vi "VR Controler 8.5.vi"() -> ()   [LabVIEW 2017]
uses:
  Sub VIs/Reward zone location enum.ctl
  Sub VIs/Record enum.ctl
  Sub VIs/Socket enum.ctl
  Sub VIs/Main program enum2.ctl
  <vilib>/vision/Image Controls.llb/IMAQ Image.ctl
  c98a875a-e3b8-49f2-a6fc-eefafe62491b.vi
  5779e0b0-41b7-4506-a67f-138f79383ca8.vi
  b241f941-595d-4c0c-9393-2e10ae48b17b.vi
  1da1cb31-40b1-4a67-a7e6-56ad72bdf787.vi
  <vilib>/DAQmx/write.llb/DAQmx Write (Digital Bool 1Line 1Point).vi
  eb595f88-4225-414f-83f1-01d5d940fc66.vi
  1662c5e6-2776-4c60-b5b4-ceaeea1864d3.vi
  fb6b5c9d-106e-453b-a883-cc93056fac18.vi
  6954e0aa-8682-46cf-8e13-c82c99879c30.vi
  6235507b-2202-4f21-86ca-b7b41428e472.vi
  835dcb76-40d0-41c5-8fe3-3989c1fd9891.vi
  4796a129-a1f4-4c2b-9c8a-39875efc01cf.vi
  bf4008ee-ae26-4c0a-87de-22156137ce73.vi
  cfabecd4-7210-4e1d-87ea-acbfc879dca4.vi
  636e59bd-2132-4706-8f21-063dc2cad597.vi
  fa866b4b-dc6c-4481-bc67-f1512cbbaaf9.vi
  f0a6b648-ccd6-4e98-b62c-d3930b5e7adb.vi
  6f1d6b9c-7e66-4bfa-a54a-0bf9111e914d.vi
  4b664865-0372-4337-9de9-faa9f3913aab.vi
  63df5311-9246-4ffc-851f-b70ac2e65be5.vi
  <vilib>/DAQmx/read.llb/DAQmx Read (Analog 2D DBL NChan NSamp).vi
  <vilib>/DAQmx/read.llb/DAQmx Read (Digital 2D U8 NChan NSamp).vi
  <vilib>/DAQmx/read.llb/DAQmx Read (Counter 1D DBL 1Chan NSamp).vi
  <vilib>/DAQmx/create/channels.llb/DAQmx Create Channel (DO-Digital Output).vi
  <vilib>/Utility/file.llb/Read Delimited Spreadsheet (string).vi
  <vilib>/DAQmx/create/channels.llb/DAQmx Create Channel (CO-Pulse Generation-Frequency).vi
  <vilib>/DAQmx/configure/timing.llb/DAQmx Timing (Implicit).vi
  <vilib>/DAQmx/miscellaneous.llb/DAQmx Fill In Error Info.vi
  <vilib>/DAQmx/create/channels.llb/DAQmx Create Channel (AI-Voltage-Basic).vi
  <vilib>/DAQmx/create/channels.llb/DAQmx Create Channel (DI-Digital Input).vi
  <vilib>/DAQmx/configure/timing.llb/DAQmx Timing (Sample Clock).vi
  <vilib>/Utility/file.llb/Write Delimited Spreadsheet (string).vi
  <vilib>/Analysis/NI_AALBase.lvlib
  3ac8b79d-dcd6-4b4b-a391-90696fb8637b.vi
  <resource>/objmgr/daqmx.rc
  2d51e364-e5e4-467f-ae98-a57dce561a7d.vi
  b1e57f22-ab38-4a20-aa80-3e76a4c4245a.vi
  e4fbd320-8e96-403f-b1da-5dadb21a4556.vi
  13745751-d4af-40e9-a17d-77a3f366e404.vi
  fbb1eb04-9408-43f0-a0c5-a56a247c35dd.vi
  <vilib>/vision/driver/NI_Vision_Acquisition_Software.lvlib
  <vilib>/Analysis/baseanly.llb/Mean (DBL).vi
  <vilib>/DAQmx/configure/task.llb/DAQmx Configure Logging (TDMS).vi
panel:
  out "Start mask stim":bool
  out "Stop mask stim":bool
  out "Mask prot command":u16
  out "Stim prot command":u16
  out "Valve open":bool
  out "Within Reward zone":bool
  out "Reward given":bool
  out "Lick":bool
  out "Masking light 2":bool
  out "Unity connected":bool
  out "Mate":bool
  out "Start light stim":bool
  out "Light ON":bool
  out "Stop light stim":bool
  out "Header":string
  in  "Software version":string
  in  "Shuffle":bool
  out "Write loop stopped":bool
  out "msg tag":string
  in  "Tab Control 4":enum32{"0", "1", "2", "3", "4"}(tab)
  in  "Tab Control 3":enum32{"0", "1", "2", "3", "4"}(tab)
  in  "Gain":dbl
  in  "sound cue presented":bool
  out "Store prev encoder count":dbl
  out "Read loop stopped":bool
  in  "index":i32
  out "Water cnt. reset":i32
  out "lick signal":i8[](array[numeric])
  out "My tdms file":refnum<k34>
  out "Trial counted":bool
  out "Stim trial":bool
  out "Write":bool
  out "read":bool
  in  "select trial":bool
  out "delta distance cm":dbl[](array[numeric])
  in  "VR Controller":enum32{"Main panel", "Settings"}(tab)
  out "Frame signal indicator 2":bool
  in  "Timed reward (s)":u32
  in  "Various GUI elements":enum32{"Misc", "Eye tracker", "Security camera"}(tab)
  in  "VR start pos":T1(ring)
  out "Opt stim command":dbl[](graph)
  out "Current stim. protocol":string
  out "Random start pos":bool=TRUE
  out "Next trial stim. protocol":string
  out "Current mask protocol":string
  out "Next mask protocol":string
  in  "start with ramp":bool
  out "stim loop rate":dbl
  out "Pupille image saved":bool
  in  "Record Button 2":bool
  in  "Black Level":dbl(slide)=0.9896907216494839 min=-32.0 max=31.75 scale=-32.0..32.0
  in  "Gain":dbl(slide)=8.879999999999999 min=0.0 max=24.0 step=1.0 scale=0.0..24.0
  in  "Exposure Time (ms)":dbl(slide)=15144.329896907217 min=1.0 max=15.0 scale=0.0..15.0
  in  "Target frame rate":dbl=60.0 min=1.0 max=144.0 step=1.0
  out "Pupille image":T2(plugin-control)
  out "Frame rate":dbl
  in  "Image Format Control::Offset X":i64(slide) min=0 max=450 step=2 scale=0.0..450.0
  in  "Image Format Control::Offset Y":i64(slide) min=0 max=350 step=2 scale=0.0..350.0
  out "Lost Image Count":u32
  out "Total Images Transferred":u32
  out "Security cam image":T2(plugin-control)
  in  "Cam ON /OFF":bool
  out "Stim. count":i32
  in  "Random reward":bool
  out "Frame signal indicator":bool
  in  "Hybrid licking":bool
  in  "Boolean":bool
  in  "SciScan":bool
  in  "Comment":string
  out "Photodiode":bool
  out "Trial type ettings":enum32{"Page 1", "Page 2"}(tab)
  in  "mask. num. 5":u16
  in  "Mask prot 5":u16(ring) items=["none", "20 Hz sinus from -80 to rew int. 100 % duty cycle 0 %", "20 Hz sinus from -50 to 10 int. 100 % duty cycle 0 %", "20 Hz sinus from 10 to 130 int. 100 % duty cycle 0 %", "20 Hz sinus from 10 to 20 int. 100 % duty cycle 0 %", "20 Hz sinus from 10 to 70 int. 100 % duty cycle 0 %", "20 Hz sinus from 10 to rew int. 100 % duty cycle 0 %", "20 Hz sinus from 0 to 70 int. 100 % duty cycle 0 %", "20 Hz sinus from 0 to 70 int. 50 % duty cycle 0 %", "continuous from 0 to 70 int. 100 % duty cycle 0 %"]
  in  "mask. num. 4":u16
  in  "Mask prot 4":u16(ring) items=["none", "20 Hz sinus from -80 to rew int. 100 % duty cycle 0 %", "20 Hz sinus from -50 to 10 int. 100 % duty cycle 0 %", "20 Hz sinus from 10 to 130 int. 100 % duty cycle 0 %", "20 Hz sinus from 10 to 20 int. 100 % duty cycle 0 %", "20 Hz sinus from 10 to 70 int. 100 % duty cycle 0 %", "20 Hz sinus from 10 to rew int. 100 % duty cycle 0 %", "20 Hz sinus from 0 to 70 int. 100 % duty cycle 0 %", "20 Hz sinus from 0 to 70 int. 50 % duty cycle 0 %", "continuous from 0 to 70 int. 100 % duty cycle 0 %"]
  in  "mask. num. 3":u16
  in  "Mask prot 3":u16(ring) items=["none", "20 Hz sinus from -80 to rew int. 100 % duty cycle 0 %", "20 Hz sinus from -50 to 10 int. 100 % duty cycle 0 %", "20 Hz sinus from 10 to 130 int. 100 % duty cycle 0 %", "20 Hz sinus from 10 to 20 int. 100 % duty cycle 0 %", "20 Hz sinus from 10 to 70 int. 100 % duty cycle 0 %", "20 Hz sinus from 10 to rew int. 100 % duty cycle 0 %", "20 Hz sinus from 0 to 70 int. 100 % duty cycle 0 %", "20 Hz sinus from 0 to 70 int. 50 % duty cycle 0 %", "continuous from 0 to 70 int. 100 % duty cycle 0 %"]
  in  "mask. num. 2":u16
  in  "Mask prot 2":u16(ring) items=["none", "20 Hz sinus from -80 to rew int. 100 % duty cycle 0 %", "20 Hz sinus from -50 to 10 int. 100 % duty cycle 0 %", "20 Hz sinus from 10 to 130 int. 100 % duty cycle 0 %", "20 Hz sinus from 10 to 20 int. 100 % duty cycle 0 %", "20 Hz sinus from 10 to 70 int. 100 % duty cycle 0 %", "20 Hz sinus from 10 to rew int. 100 % duty cycle 0 %", "20 Hz sinus from 0 to 70 int. 100 % duty cycle 0 %", "20 Hz sinus from 0 to 70 int. 50 % duty cycle 0 %", "continuous from 0 to 70 int. 100 % duty cycle 0 %"]
  out "mask. num. 1":u16
  out "Mask prot 1":u16(ring) items=["none", "20 Hz sinus from -80 to rew int. 100 % duty cycle 0 %", "20 Hz sinus from -50 to 10 int. 100 % duty cycle 0 %", "20 Hz sinus from 10 to 130 int. 100 % duty cycle 0 %", "20 Hz sinus from 10 to 20 int. 100 % duty cycle 0 %", "20 Hz sinus from 10 to 70 int. 100 % duty cycle 0 %", "20 Hz sinus from 10 to rew int. 100 % duty cycle 0 %", "20 Hz sinus from 0 to 70 int. 100 % duty cycle 0 %", "20 Hz sinus from 0 to 70 int. 50 % duty cycle 0 %", "continuous from 0 to 70 int. 100 % duty cycle 0 %"]
  in  "stim. num. 5":u16
  in  "Stim. prot 5":u16(ring) items=["none", "20 Hz sinus from -80 to rew int. 100 % duty cycle 0 %", "20 Hz sinus from -50 to 10 int. 100 % duty cycle 0 %", "20 Hz sinus from 10 to 130 int. 100 % duty cycle 0 %", "20 Hz sinus from 10 to 20 int. 100 % duty cycle 0 %", "20 Hz sinus from 10 to 70 int. 100 % duty cycle 0 %", "20 Hz sinus from 10 to rew int. 100 % duty cycle 0 %", "20 Hz sinus from 0 to 70 int. 100 % duty cycle 0 %", "20 Hz sinus from 0 to 70 int. 50 % duty cycle 0 %", "continuous from 0 to 70 int. 100 % duty cycle 0 %"]
  in  "stim. num. 4":u16
  in  "Stim. prot 4":u16(ring) items=["none", "20 Hz sinus from -80 to rew int. 100 % duty cycle 0 %", "20 Hz sinus from -50 to 10 int. 100 % duty cycle 0 %", "20 Hz sinus from 10 to 130 int. 100 % duty cycle 0 %", "20 Hz sinus from 10 to 20 int. 100 % duty cycle 0 %", "20 Hz sinus from 10 to 70 int. 100 % duty cycle 0 %", "20 Hz sinus from 10 to rew int. 100 % duty cycle 0 %", "20 Hz sinus from 0 to 70 int. 100 % duty cycle 0 %", "20 Hz sinus from 0 to 70 int. 50 % duty cycle 0 %", "continuous from 0 to 70 int. 100 % duty cycle 0 %"]
  in  "stim. num. 3":u16
  in  "Stim. prot 3":u16(ring) items=["none", "20 Hz sinus from -80 to rew int. 100 % duty cycle 0 %", "20 Hz sinus from -50 to 10 int. 100 % duty cycle 0 %", "20 Hz sinus from 10 to 130 int. 100 % duty cycle 0 %", "20 Hz sinus from 10 to 20 int. 100 % duty cycle 0 %", "20 Hz sinus from 10 to 70 int. 100 % duty cycle 0 %", "20 Hz sinus from 10 to rew int. 100 % duty cycle 0 %", "20 Hz sinus from 0 to 70 int. 100 % duty cycle 0 %", "20 Hz sinus from 0 to 70 int. 50 % duty cycle 0 %", "continuous from 0 to 70 int. 100 % duty cycle 0 %"]
  in  "stim. num. 2":u16
  in  "Stim. prot 2":u16(ring) items=["none", "20 Hz sinus from -80 to rew int. 100 % duty cycle 0 %", "20 Hz sinus from -50 to 10 int. 100 % duty cycle 0 %", "20 Hz sinus from 10 to 130 int. 100 % duty cycle 0 %", "20 Hz sinus from 10 to 20 int. 100 % duty cycle 0 %", "20 Hz sinus from 10 to 70 int. 100 % duty cycle 0 %", "20 Hz sinus from 10 to rew int. 100 % duty cycle 0 %", "20 Hz sinus from 0 to 70 int. 100 % duty cycle 0 %", "20 Hz sinus from 0 to 70 int. 50 % duty cycle 0 %", "continuous from 0 to 70 int. 100 % duty cycle 0 %"]
  out "stim. num. 1":u16
  out "Stim. prot 1":u16(ring) items=["none", "20 Hz sinus from -80 to rew int. 100 % duty cycle 0 %", "20 Hz sinus from -50 to 10 int. 100 % duty cycle 0 %", "20 Hz sinus from 10 to 130 int. 100 % duty cycle 0 %", "20 Hz sinus from 10 to 20 int. 100 % duty cycle 0 %", "20 Hz sinus from 10 to 70 int. 100 % duty cycle 0 %", "20 Hz sinus from 10 to rew int. 100 % duty cycle 0 %", "20 Hz sinus from 0 to 70 int. 100 % duty cycle 0 %", "20 Hz sinus from 0 to 70 int. 50 % duty cycle 0 %", "continuous from 0 to 70 int. 100 % duty cycle 0 %"]
  in  "Trial block":u16 max=100
  in  "Primary masking light":T3(ring)
  in  "Location of reward zone":T4 items=["80 cm", "120 cm", "180  cm", "270 cm", "400 cm"]
  in  "Enable stim.":bool
  out "GUI version":enum32{"Page 1", "Page 2"}(tab)
  out "Hit trials stim.":i32
  out "?":dbl(slide) scale=-140.0..190.0
  in  "Reset top plot":bool=TRUE caption="Reset"
  in  "Reset bottom plot":bool=TRUE caption="Reset"
  out "Hit trials ctrl.":i32
  out "P stim. Hit":dbl(slide) scale=0.0..1.0
  out "P ctrl. Hit":dbl(slide) scale=0.0..1.0
  out "Control hit trials %":dbl
  out "Stim. hit trials %":dbl
  out "Tab Control":enum32{"0", "1", "2", "3", "4"}(tab)
  out "Tab Control 2":enum32{"0", "1", "2", "3", "4"}(tab)
  out "Next":bool
  out "Top Graph":cluster{"Y":dbl[], "Y":dbl[]}[](graph) caption="XY Graph"
  out "Bottom Graph":cluster{"Y":dbl[], "Y":dbl[]}[](graph) caption="XY Graph"
  out "Hit trials %":dbl format="%#.1g"
  out "Hit trials":i16
  out "Wheel position graph":cluster{"Y":dbl[], "Y":dbl[]}[](graph) caption="XY Graph"
  in  "Reset wheel pos. graph":bool=TRUE caption="Reset"
  out "P hit trials":dbl(slide) scale=0.0..1.0
  out "Lick and reward chart 2":cluster{dbl, i16}(graph)
  out "%":dbl format="%#_3g"
  in  "Weight":dbl
  in  "Lab book notes":string
  in  "Open valve":bool
  in  "Reward freq. (cm)":dbl
  in  "Reward zone":bool
  out "Distance (m)":dbl format="%#.2g"
  in  "Record Button":bool
  in  "Reset water count":bool
  out "Water received (ul)":dbl
  in  "VR Mode":bool
  out "All trials":i32
  out "Ctrl. count":i32
  out "Unique ID":i8 format="%2d"
  in  "Stop recording":bool
  in  "Start recording":bool
  out "Laps":i32
  in  "Exit program":bool
  in  "counter reset (F)":bool caption="stop (F)"
  out "total distance cm":sgl[](array[numeric])
  out "Position on the wheel":dbl(knob) scale=0.0..157.0
  out "Experiment time (s)":dbl
  in  "Give reward":bool
  in  "Repetition":i32
  out "Date":string
  out "Run experiment":bool
  out "Velocity chart":dbl(graph)
  out "Lick and reward chart":cluster{dbl, i16}(graph)
  out "Record":bool
  out "Time (min)":dbl format="%#.2g"
  in  "Active licking":bool
  out "Mouse name":string
  in  "Scrollbar":i32(c297)
  out "Velocity chart 2":dbl(graph)
  out "Laser ON":bool
  in  "Extra stop triggers":bool
  in  "Photo diode threshold":dbl=1.5
  out "stim started":bool
  in  "Eable eye cam":bool
  out "start of stim":bool
  out "Waveform Graph":dynamicdata(graph)
  in  "Duty cycle (%)":u8=50 max=100 step=1
  out "Relative position":dbl
  out "random rew":dbl
  out "offset tag":string
  out "Masking light prot":string
  out "velocity (cm/s)":dbl
  out "Security camera":string
  out "2P imaging":string
  out "hit trial":bool
  out "Session start:":string
  out "miss trial":bool
  out "Distance (cm)":dbl
  out "Prev. rew. pos.":dbl
  out "encoder ticks per rev":dbl
  out "prev. diode position":dbl
  out "Stimulus protocol":string
  out "Laser stimulus calibration":string
  out "Original weight":dbl
  out "Last calibration":string
  in  "Edit mouse list":bool
  out "Socket read loop rate":u32(graph)
  out "Delta time (ms)":u32(graph)
  out "No. of smpl. per ch.":i32
  out "Loop rate":dbl
  out "Sample rate":dbl
  out "reward zone end":dbl
  out "reward zone start":dbl
  in  "Corridor length":i32
  out "delta time (s)":dbl format="%#.8g"
  out "Experiment time (ms)":u32
  out "Start time":u32
  in  "Sound duration (ms)":u32=25
  in  "Valve open dur. (ms)":u32=25
  in  "working directory":path=path ""
  in  "command line":string
  in  "Recording folder":path
  out "Wheel circumference":dbl
  in  "Record enum":T5
  in  "Reward size (ul)":dbl min=0.0 step=inf format="%#.2g"
  in  "working directory 2":path=path ""
  out "Record loop state":T5
  out "Reward read loop rate":u32(graph)
  out "shuffled array":i16[](array[numeric])
  in  "Current mice":string[][](array[string])
  out "Trial types":u16[][](array[numeric])
  out "Last saved reward size":dbl
  out "Encoder count":dbl
  out "Lick indicator":dbl
  out "Lab book file":path
  out "Filename":string
  out "Frame signal":i8[](array[numeric])
  out "Water count":i32
  out "Unity position:":sgl
  out "Raw position:":dbl
  out "Photodiode signal":sgl[](array[numeric])
  out "Trial type array":i8[][](array[numeric])
  out "Valve signal":i8[](array[numeric])
  out "SciScan start":refnum<k21>
  out "Photo stimulus signal":sgl[](array[numeric])
  in  "NBC Gain":dbl
  out "Encoder signal":sgl[](array[numeric])
  out "analog lick":sgl[](array[numeric])
  out "protocol array":string[][](array[string])
  in  "Stim protocols":u16(ring) items=["none", "20 Hz sinus from -80 to rew int. 100 % duty cycle 0 %", "20 Hz sinus from -50 to 10 int. 100 % duty cycle 0 %", "20 Hz sinus from 10 to 130 int. 100 % duty cycle 0 %", "20 Hz sinus from 10 to 20 int. 100 % duty cycle 0 %", "20 Hz sinus from 10 to 70 int. 100 % duty cycle 0 %", "20 Hz sinus from 10 to rew int. 100 % duty cycle 0 %", "20 Hz sinus from 0 to 70 int. 100 % duty cycle 0 %", "20 Hz sinus from 0 to 70 int. 50 % duty cycle 0 %", "continuous from 0 to 70 int. 100 % duty cycle 0 %"]
  in  "Stim type":u16(ring) items=["none", "10 Hz sinus", "20 Hz sinus", "40 Hz sinus", "continuous", "10 Hz square", "20 Hz square", "40 Hz square"]
  in  "from reward":bool
  in  "to reward":bool
  in  "Intensity (%)":u8=100 max=100 step=1
  in  "stop (cm)":i32
  in  "start (cm)":i32
  out "prev. stim. type":string
  out "prev. max stim. V":dbl
  out "Eye cam frame signal":i8[](array[numeric])
  in  "Eable security cam":bool
  out "Eyecam states":T6(ring)
  out "settings folder":path
  out "Pupil Exp day folder":path
  out "ML signal":sgl[](array[numeric])
  out "Frame signal 2":i8[](array[numeric])
  out "Exit":bool
  out "Stop Unity":bool
  # "All"
  # "This session"
  # "Reward conditions"
  # "Trial type settings"
  # "Determine stimulus protocol and \nreperition (numerator) in relation \nto the denominator!"
  # "%"
  # "%"
  # "%"
  # "Edit stimulus protocols for photo stimulation and/or \na secondary masking light. Chose a protocol from the \nlist and define parameters."
  # "Mouse name               Headbar           Original weight"
  # "Variables"
  # "Reward settings"
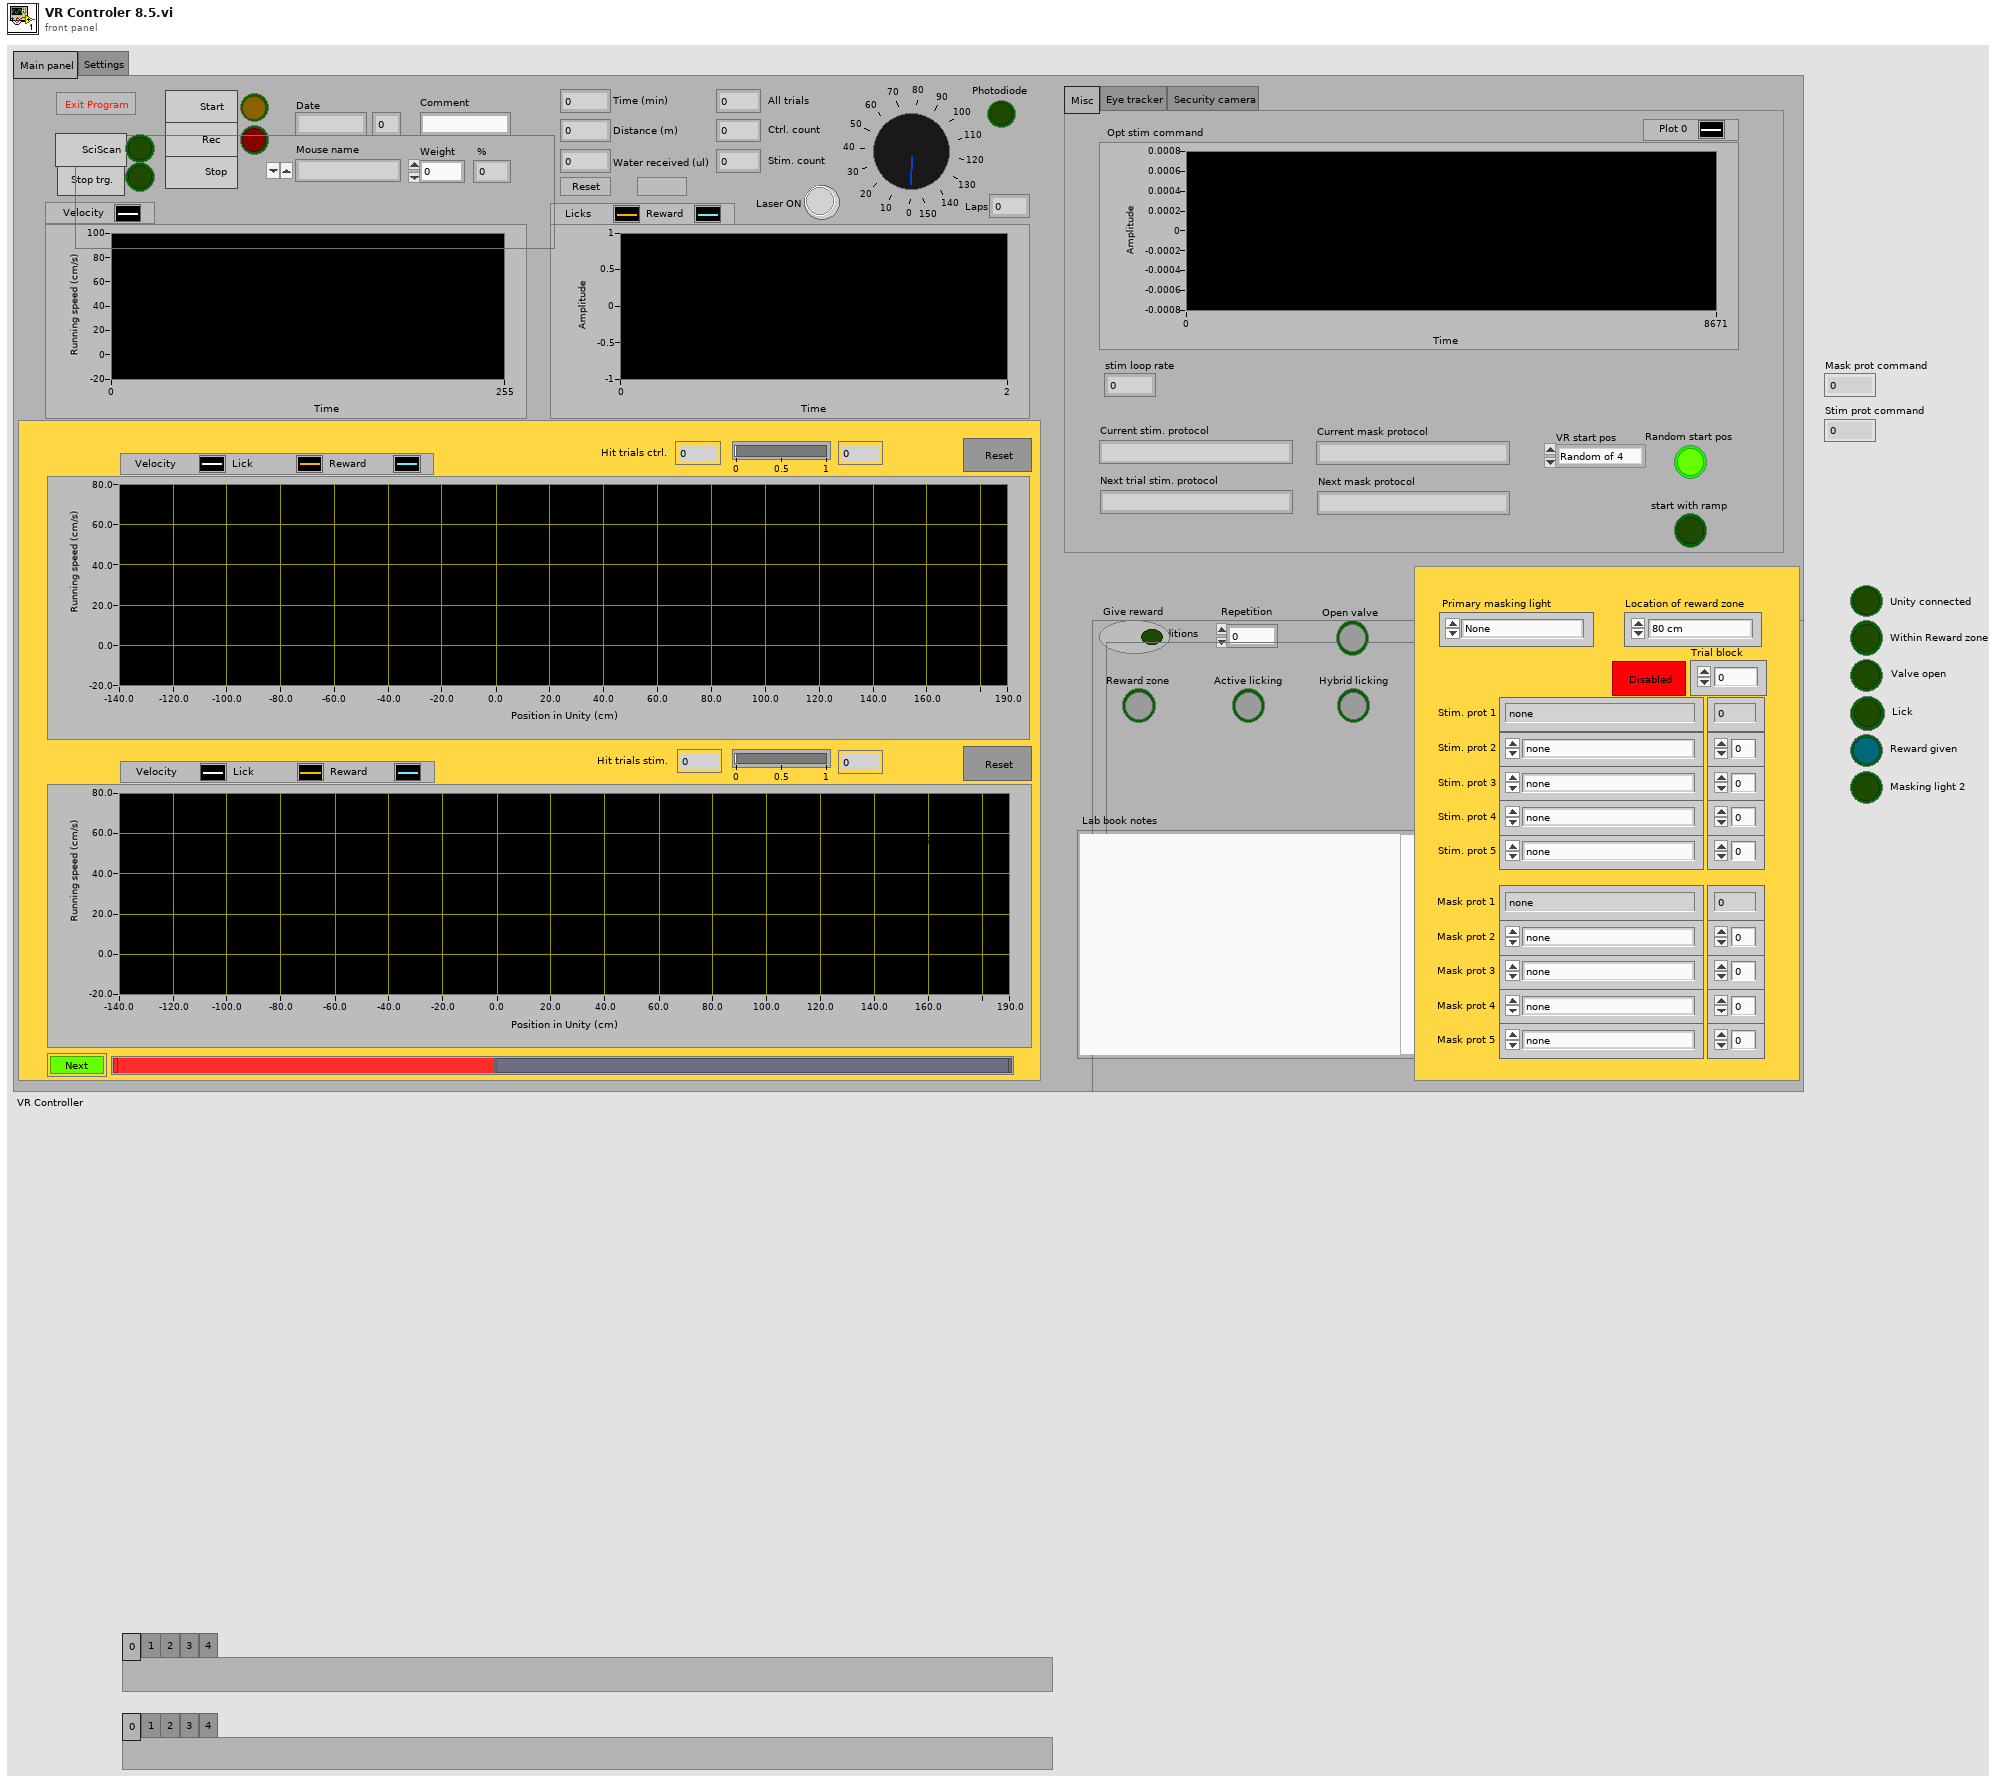
[diagram p1: front panel]
types:
  T1 = enum16{"Random of 4", "Random of 2", "Non-random"}
  T2 = typedef "IMAQ Image.ctl" = refnum<image>
  T3 = enum16{"None", "20 Hz until reward ", "Continuous specified light off trials", "Continuous specified all trials", "20 Hz specified light off trials", "20 Hz specified all trials", "20 Hz full trial", "Continuous full trial"}
  T4 = typedef "Reward zone location enum.ctl" = u16
  T5 = typedef "Record enum.ctl" = enum16{"Idle", "Init recording", "Init data acquisition", "Record VR", "Record", "Stop data acquision"}
  T6 = enum16{"Idle", "Set params", "Start recording", "Record pupille", "Stop recording"}
  T7 = enum8{"Enabled", "Disabled", "Disabled and Grayed Out"}
  T8 = typedef "Main program enum2.ctl" = enum16{"Init program", "Idle", "Init recording ", "Record", "Record VR", "Stop Recording", "Exit program"}
  T9 = typedef "Socket enum.ctl" = enum16{"Socket not connected", "Init socket", "Socket connected", "Close socket"}
  T10 = cluster{"Type":u32, "Version":u32, "Flags":u32, "SerialNumberHigh":u32, "SerialNumberLow":u32, "BusType":u32, "InterfaceName":string, "VendorName":string, "ModelName":string, "CameraFileName":string, "CameraAttributeURL":string}[]
  T11 = enum16{"open", "replace", "create", "open or create", "replace or create", "replace or create with confirmation"}
  T12 = enum16{"Init program", "Idle", "Init recording ", "Record", "Record VR", "Stop Recording", "Exit program"}
  T13 = enum16{"None", "Full trial 40 Hz sinus ", "Full trial 20 Hz sinus", "Continuous light ON", "Until reward 40 Hz sinus"}
  T14 = enum16{"None", "20 Hz until reward ", "Continuous specified light off trials", "Continuous specified all trials", "20 Hz specified light off trials", "20 Hz specified all trials"}
  T15 = typedef "LVStringsAndValuesArrayTypeDef_U16.ctl" = cluster{"String":string, "Value":u16}[]
  T16 = enum16{"open", "open or create", "create or replace", "create", "open (read-only)"}
  T17 = enum16{"Standard", "Buffered", "CRLF", "Immediate"}
  T18 = enum16{"None", "20 Hz until reward ", "Continuous specified light off trials", "Continuous specified all trials", ""}
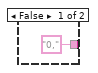
[diagram p2: hidden frame]
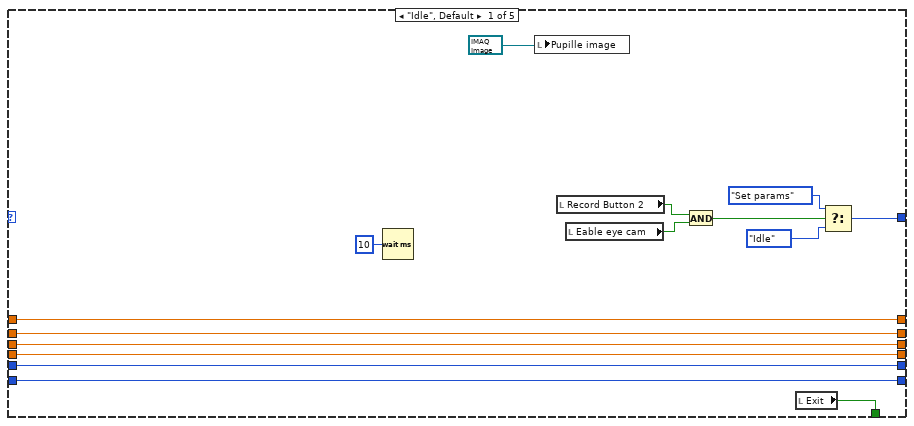
[diagram p5: hidden frame]
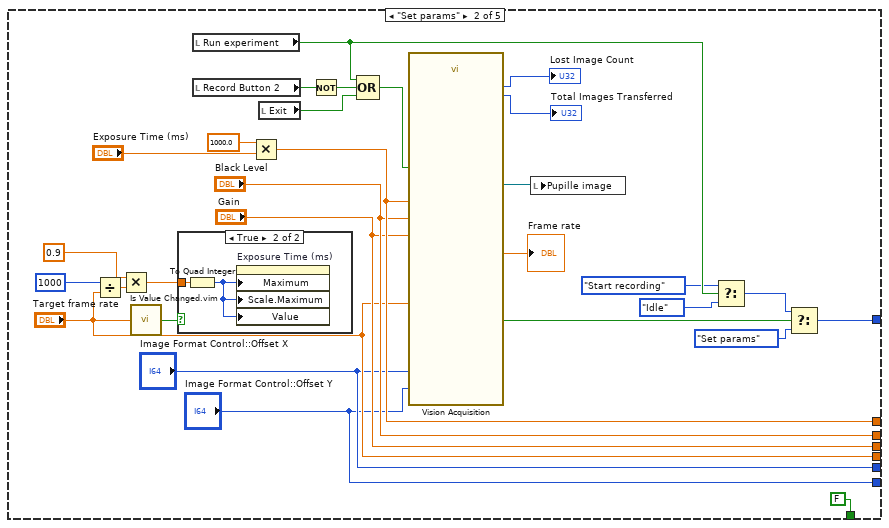
[diagram p6: hidden frame]
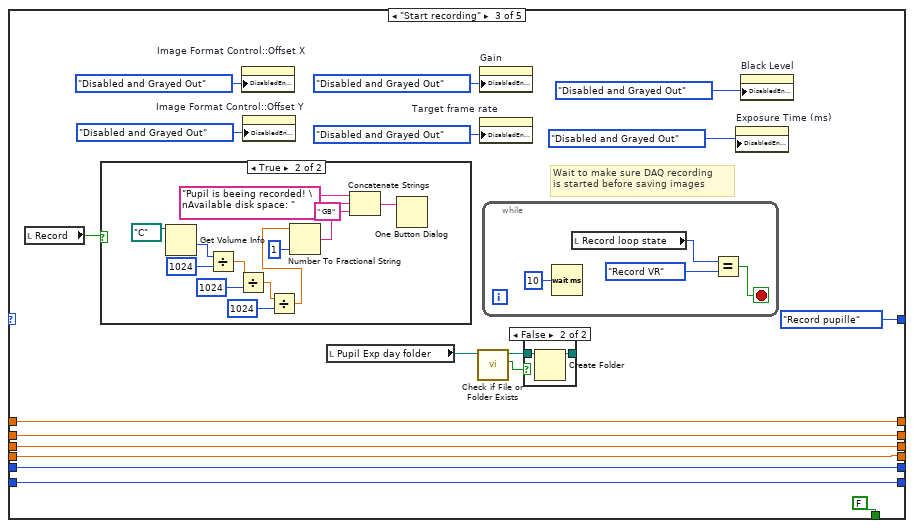
[diagram p8: hidden frame]
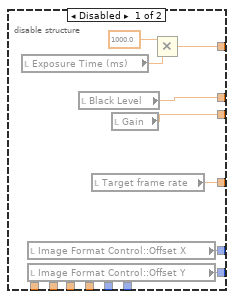
[diagram p11: hidden frame]
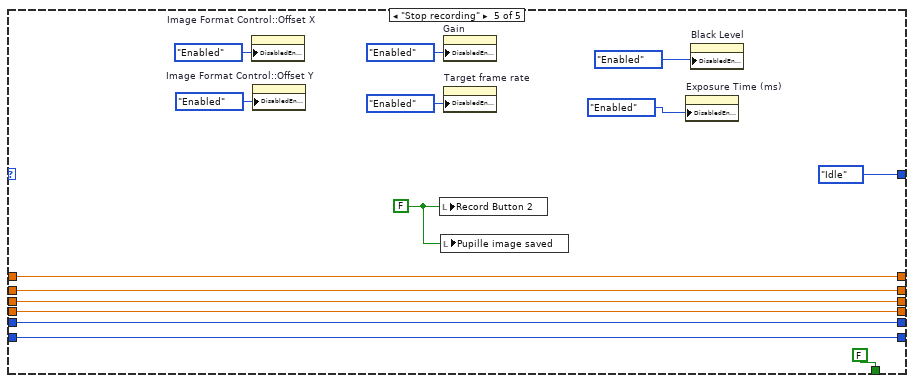
[diagram p12: hidden frame]
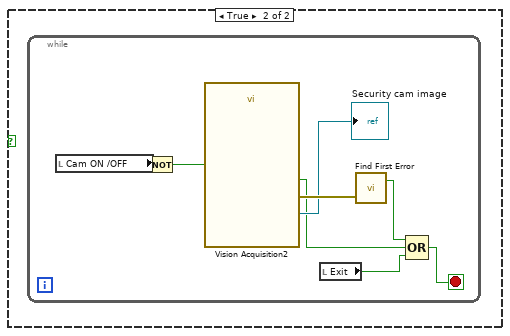
[diagram p13: hidden frame]
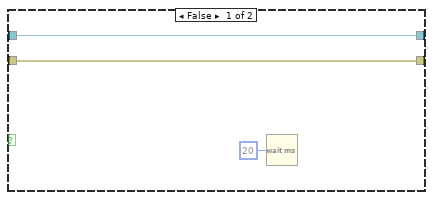
[diagram p18: hidden frame]
diagram:
  w5 = FALSE ("Eable eye cam")
  w6 = FALSE ("Record Button 2")
  w7 = 60 ("y")
  w39 = "rew" ("regular expression")
  w37 = "rew" ("regular expression")
  w31 = "continuous" ("regular expression")
  w33 = "none" ("regular expression")
  w51 = "rew" ("regular expression")
  w53 = "rew" ("regular expression")
  w59 = "continuous" ("regular expression")
  w57 = "none" ("regular expression")
  (unwired) string[] ["Photo-diode", "Time (s)", "Delta Time (ms)", "Distance (cm)", "Valve open", "Frame signal", "Lick signal", "Photo stimulus signal", "Laser ON", "Position in Unity", "Corridor indicator"] ("channel name(s) in (Untitled)")
  (unwired) path "C:/Users/vrsetup/Desktop/VR Controller/Laser stimulus calibration.txt" ("file path (dialog if empty)")
  w77 = FALSE ("Reset")
  # "Defaults"
  # "Keep order of default variables:\nUser:\tMate\nLoop rate:\t100\nSampling rate:\t3000\nEncoder tisks:\t4000\nRecording folder:\tC:\\Users\\vrsetup\\Desktop\nEnable VR more(Y/N):\tY\n..."
  # "File versions:\n-8.5 User profile selector\n\n-8.3 Camera control added> Pupil imaging and security camera\nTimed reward\n\n-8.2 with 8.4 unity version: \nNew task without cue\nImportant bugfixes in photo-stimulation, start stimulus with ramp option is added\nSafety switch shuts off stimulus after 10s \n\n-8.0 - 8.2\nNew task wersionm new optogenetic prorocol solutions\n\n-7.5 - 2019.07.10\nRandom reward option\n\n-7.5\nNew Unity version: coupling error is corrected! (interpolation factor discarded), randomizeable starting point.\nTiki-taka task for Nora\nNew masking light functions : 20Hz specified in light off or all trials\n\n\n-7.3\nMasking light options are added\nMasking light protocol is saved now in labbook\n\n-7.2\nmade GitHub compatible: folder path and some default variables are red from txt file and txt data files are now in separate folder\ndate is formated with different method\n\n-7.1\nsaves Encoder signal and imaging/security camera YES NO indication is added to lab book\nsaves Analog lick signal\n\n-7.0 \nMasking light\n\n-6.9\nData typed are changed back to DBL\n\n-6.8\nDifferent data saving settings to reduce file size by specifying data types\nCorrect trial % corrected after 2018.12.05\nHybrid licking\nPhoto stimulus trials and counting of \"Hit trials \"for Nora\n\n-6.7 \nfor Mate Loop rate from 200 -> 100 Hz  (should not affect VR that is 60 Hz) \nrecorded sampling rate increased 200 -> 3000 Hz\nswitch to show water consumption in current session is added\n\n\n\n..."
  n1 = flat-sequence {
    tunnel: [w137] -> w1
    tunnel: w1 -> [w169]
    tunnel: [Socket_enum."Socket not connected" ("Enum")] -> w129
    tunnel: [Main_program_enum2."Init program" ("main program")] -> w128
    tunnel: [Record_enum."Idle" ("Record enum")] -> w121
    tunnel: [TRUE ("VR Mode")] -> w76
    frame #0 {
      # "Select user profile"
      n2 = call <vilib>:"Recursive File List.vi"("Folder Path"=path "C:/VR Controller/data" ("path")) -> ("All Folders"=w143:path[])  [unwired: 6 in, 4 out]
      n3 = Array Size(array=w143) -> (size(s)=w148:i32)
      n4 = for {
        N: w148 -> [_]
        tunnel: w143 -> [w159] mode=indexing
        shift-right: [w156] -> w145
        shift-left: string[] [] -> [w155]
        i -> [w157]
        n5 = Strip Path(path=w159) -> (name=w158:string)  [unwired: 1 out]
        n6 = Insert Into Array(array=w155, index=w157, new element=w158) -> (w156:string[])
      }
      n7 = Array Size(array=w145) -> (size(s)=w136:i32)
      n8 = Greater?(x=w136, y=1) -> (0:w134:bool)
      n9 = Array Subset(array=w145, index=1, length=w136) -> (w144:string[])
      n10 = case shown="True" w134 {
        tunnel: w144 -> [_ w154]
        tunnel: w143 -> [_ w153]
        tunnel: [path "" ("path") w150] -> w139
        frame False {
        }
        frame True {
          n11 = call "Get User Input.vi"("Strings []"=w154) -> ("user"=w152:u16)  [unwired: 1 in, 9 out]
          n12 = Increment(x=w152) -> (x+1=w151:u16)
          n13 = Index Array(array=w153, index=w151) -> (element=w150:path)
        }
      }
      n14 = Equal?(x=w139, y=path "" ("path")) -> (x = y?=w141:bool)
      n15 = Select(t=path "C:/VR Controller/data", s=w141, f=w139) -> (s? t:f=w137:path)
      "settings folder" <- w137
    }
    frame #1 {
      w174 = 1 ("length")
      w179 = 1 ("length")
      w192 = 1 ("length")
      w195 = 1 ("length")
      w198 = 1 ("length")
      w201 = 1 ("length")
      # "VI version"
      # "Enable VR mode"
      n16 = Build Path(base path=w169, name or relative path="Default variables.txt") -> (appended path=w167:path)
      n17 = call-poly <vilib>:"Read Delimited Spreadsheet.vi"("file path (dialog if empty)"=w167) -> ("all rows"=w170:string[][])  [unwired: 9 in, 5 out]
      n18 = Array Subset(array=w170, index (row)=0 ("index"), length (row)=w201, index (col)=w201, length (col)=w201) -> (w200:string[][])
      n19 = Array Subset(array=w170, index (row)=1 ("index"), length (row)=w198, index (col)=w198, length (col)=w198) -> (w199:string[][])
      n20 = Array Subset(array=w170, index (row)=2 ("index"), length (row)=w179, index (col)=w179, length (col)=w179) -> (w176:string[][])
      n21 = Array Subset(array=w170, index (row)=3 ("index"), length (row)=w195, index (col)=w195, length (col)=w195) -> (w194:string[][])
      n22 = Array Subset(array=w170, index (row)=4 ("index"), length (row)=w192, index (col)=w192, length (col)=w192) -> (w193:string[][])
      n23 = Array Subset(array=w170, index (row)=5 ("index"), length (row)=w174, index (col)=w174, length (col)=w174) -> (w173:string[][])
      n24 = Concatenate Strings(w200) -> (w186:string)
      n25 = Concatenate Strings(w199) -> (w188:string)
      n26 = Concatenate Strings(w176) -> (w180:string)
      n27 = Concatenate Strings(w194) -> (w189:string)
      n28 = Concatenate Strings(w193) -> (w190:string)
      n29 = Concatenate Strings(w173) -> (w172:string)
      n30 = String To Path(string=w190) -> (path=w161:path)
      n31 = Fract/Exp String To Number(string=w180) -> (number=w177:dbl)  [unwired: 3 in, 1 out]
      n32 = Fract/Exp String To Number(string=w189) -> (number=w184:dbl)  [unwired: 3 in, 1 out]
      n33 = Fract/Exp String To Number(string=w188) -> (number=w185:dbl)  [unwired: 3 in, 1 out]
      n34 = Equal?(x=w186, y="Mate") -> (x = y?=w165:bool)
      n35 = Equal?(x=w172, y="Y") -> (x = y?=w166:bool)
      n36 = case shown="True" w166 {
        tunnel: w170 -> [_ w209]
        tunnel: [path "" w207] -> w160
        frame False {
          (unwired) FALSE ("T button?")
        }
        frame True {
          w212 = 1 ("length")
          n37 = Array Subset(array=w209, index (row)=6 ("index"), length (row)=w212, index (col)=w212, length (col)=w212) -> (w210:string[][])
          n38 = Concatenate Strings(w210) -> (w208:string)
          n39 = local write "command line"(w208) -> ()
          n40 = String To Path(string=w208) -> (path=w207:path)
        }
      }
      n41 = local write "Loop rate"(w185) -> ()
      n42 = local write "Sample rate"(w177) -> ()
      n43 = local write "encoder ticks per rev"(w184) -> ()
      n44 = local write "Recording folder"(w161) -> ()
      n45 = local write "Mate"(w165) -> ()
      n46 = case shown="True" w165 {
        frame False {
          n47 = local write "Sound duration (ms)"(u32 0 ("Sound duration (ms)")) -> ()
        }
        frame True {
          n48 = local write "Sound duration (ms)"(u32 5 ("Sound duration (ms)")) -> ()
        }
      }
      n49 = local write "VR Mode"(w166) -> ()
      n50 = Current VI's Path() -> (path=w164:path)
      n51 = case shown="False" w165 {
        tunnel: [enum32{"Page 1", "Page 2"}."Page 2" ("GUI version") w243] -> w204
        tunnel: [enum32{"Page 1", "Page 2"}."Page 1" ("GUI version") w243] -> w203
        frame False {
          n52 = property on="Top Graph" class="XYGraph (strict)"("DisabledEnum"=T7."Disabled" ("Disabled")) -> ()  [unwired: 2 in, 2 out]
          n53 = property on="Bottom Graph" class="XYGraph (strict)"("DisabledEnum"=T7."Disabled" ("Disabled")) -> ()  [unwired: 2 in, 2 out]
          n54 = property on="Wheel position graph" class="XYGraph (strict)"("DisabledEnum"=T7."Enabled" ("Disabled")) -> ()  [unwired: 2 in, 2 out]
          n55 = property on="Lick and reward chart" class="WFChart (strict)"("Visible"=FALSE, "DisabledEnum"=T7."Disabled" ("Disabled")) -> ()  [unwired: 2 in, 2 out]
          n56 = property on="Velocity chart" class="WFChart (strict)"("Visible"=FALSE, "DisabledEnum"=T7."Disabled" ("Disabled")) -> ()  [unwired: 2 in, 2 out]
          n57 = property on="Reset top plot" class="Bool (strict)"("DisabledEnum"=T7."Disabled" ("Disabled")) -> ()  [unwired: 2 in, 2 out]
          n58 = property on="Reset wheel pos. graph" class="Bool (strict)"("DisabledEnum"=T7."Enabled" ("Disabled")) -> ()  [unwired: 2 in, 2 out]
          n59 = property on="Reset bottom plot" class="Bool (strict)"("DisabledEnum"=T7."Disabled" ("Disabled")) -> ()  [unwired: 2 in, 2 out]
          n60 = property on="Lick and reward chart 2" class="WFChart (strict)"("Visible"=TRUE, "DisabledEnum"=T7."Enabled" ("Disabled")) -> ()  [unwired: 2 in, 2 out]
          n61 = property on="Velocity chart 2" class="WFChart (strict)"("Visible"=TRUE, "DisabledEnum"=T7."Enabled" ("Disabled")) -> ()  [unwired: 2 in, 2 out]
        }
        frame True {
          w243 = enum32{"Page 1", "Page 2"}."Page 1" ("GUI version")
          n62 = property on="Lick and reward chart" class="WFChart (strict)"("Visible"=TRUE, "DisabledEnum"=T7."Enabled" ("Disabled")) -> ()  [unwired: 2 in, 2 out]
          n63 = property on="Velocity chart" class="WFChart (strict)"("Visible"=TRUE, "DisabledEnum"=T7."Enabled" ("Disabled")) -> ()  [unwired: 2 in, 2 out]
          n64 = property on="Top Graph" class="XYGraph (strict)"("DisabledEnum"=T7."Enabled" ("Disabled")) -> ()  [unwired: 2 in, 2 out]
          n65 = property on="Bottom Graph" class="XYGraph (strict)"("DisabledEnum"=T7."Enabled" ("Disabled")) -> ()  [unwired: 2 in, 2 out]
          n66 = property on="Wheel position graph" class="XYGraph (strict)"("DisabledEnum"=T7."Disabled" ("Disabled")) -> ()  [unwired: 2 in, 2 out]
          n67 = property on="Reset top plot" class="Bool (strict)"("DisabledEnum"=T7."Enabled" ("Disabled")) -> ()  [unwired: 2 in, 2 out]
          n68 = property on="Reset wheel pos. graph" class="Bool (strict)"("DisabledEnum"=T7."Disabled" ("Disabled")) -> ()  [unwired: 2 in, 2 out]
          n69 = property on="Reset bottom plot" class="Bool (strict)"("DisabledEnum"=T7."Enabled" ("Disabled")) -> ()  [unwired: 2 in, 2 out]
          n70 = property on="Lick and reward chart 2" class="WFChart (strict)"("Visible"=FALSE, "DisabledEnum"=T7."Disabled" ("Disabled")) -> ()  [unwired: 2 in, 2 out]
          n71 = property on="Velocity chart 2" class="WFChart (strict)"("Visible"=FALSE, "DisabledEnum"=T7."Disabled" ("Disabled")) -> ()  [unwired: 2 in, 2 out]
        }
      }
      "GUI version" <- w204
      "Trial type ettings" <- w203
      n72 = Strip Path(path=w164) -> (name=w163:string)  [unwired: 1 out]
      n73 = Strip Path(path=w160) -> (name=w162:string)  [unwired: 1 out]
      n74 = disable-structure shown="Disabled" {
        frame Disabled {
          n75 = local write "command line"("C:\\VR Controller\\corridor1\\LVcontrol_6.exe" ("command line")) -> ()
        }
        frame Enabled {
        }
      }
      n76 = case shown="True" w166 {
        tunnel: ["" ("string") w215] -> w182
        tunnel: w162 -> [_ w214]
        frame False {
        }
        frame True {
          n77 = Concatenate Strings(";    Unity VR version: " ("string"), w214) -> (w215:string)
        }
      }
      n78 = Concatenate Strings(w163, w182, "(2021.11.09)" ("string")) -> (w183:string)
      n79 = local write "Software version"(w183) -> ()
    }
    frame #2 {
      # "Has to be integer!"
      n80 = call <vilib>:"IMAQdx Enumerate Cameras.vi"() -> ("Camera Information Array"=w250:T10)  [unwired: 10 in, 1 out]
      n81 = local read "Sample rate"() -> (w253:dbl)
      n82 = for {
        tunnel: w250 -> [w263] mode=indexing
        # "Eye camera available"
        # "Security camera available"
        n83 = Unbundle By Name(w263) -> ("VendorName"=w260:string)
        n84 = Equal?(x="Microsoft® LifeCam Studio(TM)", y=w260) -> (x = y?=w258:bool)
        n85 = Equal?(x=w260, y="Basler") -> (x = y?=w259:bool)
        n86 = case shown="True" w258 {
          selector: w258 -> [_ w264]
          frame False {
          }
          frame True {
            n87 = local write "Eable security cam"(w264) -> ()
            n88 = property on="Cam ON /OFF" class="Bool (strict)"("DisabledEnum"=T7."Enabled" ("Disabled")) -> ()  [unwired: 2 in, 2 out]
          }
        }
        n89 = case shown="True" w259 {
          selector: w259 -> [_ w266]
          frame False {
          }
          frame True {
            n90 = local write "Eable eye cam"(w266) -> ()
            n91 = property on="Record Button 2" class="Bool (strict)"("DisabledEnum"=T7."Enabled" ("Disabled")) -> ()  [unwired: 2 in, 2 out]
          }
        }
      }
      n92 = local read "Loop rate"() -> (w254:dbl)
      n93 = Divide(x=w253, y=w254) -> (x/y=w255:dbl)
      n94 = local write "No. of smpl. per ch."(w255) -> ()
    }
  }
  n95 = property on="Mate" class="Bool (strict)"("Visible"=FALSE) -> ()  [unwired: 2 in, 2 out]
  n96 = property on="Software version" class="Str"("Visible"=FALSE) -> ()  [unwired: 2 in, 2 out]
  n97 = disable-structure shown="Disabled" {
    frame Disabled {
      n98 = call-poly <vilib>:"DAQmx Configure Logging.vi"() -> ()  [unwired: 14 in, 2 out]
    }
    frame Enabled {
    }
  }
  n99 = disable-structure shown="Disabled" {
    frame Disabled {
      n100 = local read "Unity connected"() -> (w268:bool)
      n101 = case shown="False" w268 {
        frame False {
          n102 = case shown="True" {
            selector: _ -> [_ _]
            frame False {
            }
            frame True {
              n103 = call <vilib>:"System Exec.vi"("wait until completion? (T)"=FALSE, "working directory"="working directory", "command line"="command line") -> ()  [unwired: 5 in, 4 out]
              n104 = Wait (ms)(milliseconds to wait=u32 1000) -> ()  [unwired: 1 out]
            }
          }
        }
        frame True {
        }
      }
    }
    frame Enabled {
    }
  }
  n105 = local write "Eable security cam"(w5) -> ()
  n106 = local write "Eable eye cam"(w5) -> ()
  n107 = property on="Cam ON /OFF" class="Bool (strict)"("DisabledEnum"=T7."Disabled and Grayed Out" ("Disabled")) -> ()  [unwired: 2 in, 2 out]
  n108 = property on="Record Button 2" class="Bool (strict)"("DisabledEnum"=T7."Disabled and Grayed Out" ("Disabled")) -> ()  [unwired: 2 in, 2 out]
  n109 = disable-structure shown="Disabled" {
    frame Disabled {
      # "These computations run only once in a trial when the mouse enters to the RZ"
      n110 = local read "reward zone start"() -> (w277:dbl)
      n111 = local read "Unity position:"() -> (w276:sgl)
      n112 = local read "select trial"() -> (w275:bool)
      n113 = Greater?(x=w276, y=w277) -> (0:w274:bool)
      n114 = Compound Arithmetic op=AND(w274, w275) -> (w273:bool)
      n115 = case shown="True" w273 {
        frame True {
          w280 = FALSE ("Randomize")
          n116 = local read "Random start pos"() -> (w279:bool)
          n117 = local write "Trial counted"(w280) -> ()
          n118 = local write "select trial"(w280) -> ()
          n119 = case shown="True" w279 {
            tunnel: ["0," w282] -> w278
            frame False {
            }
            frame True {
              n120 = Build Array("0,", "2,", "4,", "6,") -> (w285:string[])
              n121 = call "Shuffle 1D Array.vim"("array"=w285) -> ("shuffled array"=w283:string[])  [unwired: 4 in]
              n122 = Index Array(array=w283, index=0) -> (element=w282:string)
            }
          }
          n123 = local write "offset tag"(w278) -> ()
        }
        frame False {
        }
      }
    }
    frame Enabled {
    }
  }
  n124 = property on="Stim trial" class="Bool (strict)"("Visible"=FALSE) -> ()  [unwired: 2 in, 2 out]
  n125 = local write "Reward given"(TRUE ("Reward given")) -> ()
  n126 = property on="msg tag" class="Str"("Visible"=FALSE) -> ()  [unwired: 2 in, 2 out]
  n127 = local write "msg tag"("str," ("msg tag")) -> ()
  n128 = property on="Trial counted" class="Bool (strict)"("Visible"=FALSE) -> ()  [unwired: 2 in, 2 out]
  n129 = property on="VR Mode" class="Bool (strict)"("Visible"=FALSE) -> ()  [unwired: 2 in, 2 out]
  n130 = local write "Security camera"("Security camera: NO" ("Security camera")) -> ()
  n131 = property on="Gain" class="DigNum (strict)"("Visible"=FALSE) -> ()  [unwired: 2 in, 2 out]
  n132 = Divide(x=1000, y=w7) -> (x/y=w9:dbl)
  n133 = property on="lick signal" class="Arr (strict)"("Visible"=FALSE) -> ()  [unwired: 2 in, 2 out]
  n134 = property on="Header" class="Str"("Visible"=FALSE) -> ()  [unwired: 2 in, 2 out]
  n135 = disable-structure shown="Disabled" {
    frame Disabled {
      n136 = Add Array Elements() -> (numeric array=w292:dbl[], sum=w291:dbl)
      n137 = Array Size(array=w292) -> (size(s)=w290:i32)
      n138 = Divide(x=w291, y=w290) -> ()  [unwired: 1 out]
    }
    frame Enabled {
    }
  }
  n139 = local write "Target frame rate"(w7) -> ()
  n140 = local write "Write loop stopped"(TRUE ("Read loop stopped")) -> ()
  n141 = local write "Read loop stopped"(TRUE ("Read loop stopped")) -> ()
  n142 = property on="Read loop stopped" class="Bool (strict)"("Visible"=FALSE) -> ()  [unwired: 2 in, 2 out]
  n143 = property on="Write loop stopped" class="Bool (strict)"("Visible"=FALSE) -> ()  [unwired: 2 in, 2 out]
  n144 = property on="delta distance cm" class="Arr (strict)"("Visible"=FALSE) -> ()  [unwired: 2 in, 2 out]
  n145 = Multiply(x=0.9, y=w9) -> (x*y=w11:dbl)
  n146 = local write "Recording folder"("Recording folder") -> ()
  n147 = To Quad Integer(1:w11) -> (0:w12:i64)
  n148 = Get Date/Time String(date format (0)=enum16{"short", "long", "abbreviated"}."short") -> ()  [unwired: 2 in, 2 out]
  n149 = property on="delta distance cm" class="DigNum (strict)"("Visible"=FALSE) -> ()  [unwired: 2 in, 2 out]
  n150 = local write "to reward"(FALSE ("to reward")) -> ()
  n151 = local write "Encoder count"(0.0 ("Encoder count")) -> ()
  n152 = property on="from reward" class="Bool (strict)"("DisabledEnum"=T7."Disabled and Grayed Out" ("Disabled")) -> ()  [unwired: 2 in, 2 out]
  n153 = property on="Lab book file" class="Path"("Visible"=TRUE) -> ()  [unwired: 2 in, 2 out]
  n154 = local write "Record Button 2"(w6) -> ()
  n155 = property on="Corridor length" class="DigNum (strict)"("Visible"=FALSE) -> ()  [unwired: 2 in, 2 out]
  n156 = local write "Pupille image saved"(w6) -> ()
  n157 = property on="index" class="DigNum (strict)"("Visible"=FALSE) -> ()  [unwired: 2 in, 2 out]
  n158 = property on="Exposure Time (ms)" class="Slide (strict)"("Maximum"=w12, "Scale.Maximum"=w12, "Value"=w12) -> ()  [unwired: 2 in, 2 out]
  n159 = while {
    shift-right: [w293] -> _
    shift-left: w128 -> [w295]
    stop <- w296 stop-if-true
    n160 = case shown="\"Stop Recording\"" w295 {
      tunnel: [T12."Idle" ("main program") w468 w792 T12."Idle" ("main program") T12."Idle" ("main program") w921 w1049] -> w293
      frame "Init program", Default {
        w304 = u16 0 ("Mask prot command")
        w306 = u16 0 items=["none"] ("Stim. prot 1")
        w307 = u16 0 ("stim. num. 2")
        n161 = local write "Unique ID"(i8 0 ("Unique ID")) -> ()
        n162 = local write "Run experiment"(FALSE ("Record")) -> ()
        n163 = local write "SciScan"(FALSE ("SciScan")) -> ()
        n164 = local write "Edit mouse list"(FALSE ("Edit mouse list")) -> ()
        n165 = local write "Trial block"(u16 10 ("Denominator")) -> ()
        n166 = local read "settings folder"() -> (w302:path)
        n167 = call-poly <vilib>:"DAQmx Create Virtual Channel.vi"("lines"=tag "Dev1/port0/line0") -> ("task out"=→"SciScan start":refnum<k21>)  [unwired: 13 in, 1 out]
        n168 = local write "stim. num. 2"(w307) -> ()
        n169 = local write "stim. num. 3"(w307) -> ()
        n170 = local write "stim. num. 4"(w307) -> ()
        n171 = local write "stim. num. 5"(w307) -> ()
        n172 = local write "mask. num. 2"(w307) -> ()
        n173 = local write "mask. num. 3"(w307) -> ()
        n174 = local write "mask. num. 4"(w307) -> ()
        n175 = local write "mask. num. 5"(w307) -> ()
        n176 = Build Path(base path=w302, name or relative path="List of mice.txt") -> (appended path=w301:path)
        n177 = call-poly <vilib>:"Read Delimited Spreadsheet.vi"("file path (dialog if empty)"=w301) -> ("all rows"=w328:string[][])  [unwired: 9 in, 5 out]
        n178 = flat-sequence {
          frame #0 {
            n179 = property on="Stim protocols" class="Ring (strict)"("Strings []"=string[] []) -> ()  [unwired: 2 in, 2 out]
          }
          frame #1 {
            n180 = local read "settings folder"() -> (w333:path)
            n181 = Build Path(base path=w333, name or relative path="Stimprotocols.txt") -> (appended path=w331:path)
            n182 = call-poly <vilib>:"Read Delimited Spreadsheet.vi"("file path (dialog if empty)"=w331) -> ("all rows"=w336:string[][])  [unwired: 9 in, 5 out]
            "protocol array" <- w336
            n183 = Array Size(array=w336) -> (size(s)=w339:i32[])
            n184 = Index Array(array=w339, index=0) -> (element=w337:i32)
            n185 = for {
              N: w337 -> [_]
              tunnel: w336 -> [w350] mode=indexing
              shift-right: [w348] -> w334
              shift-left: string[] [] -> [w347]
              i -> [w349]
              n186 = Concatenate Strings(w350) -> (w344:string)
              n187 = Match Pattern(string=w344, regular expression="none") -> (before substring=w342:string, match substring=w341:string)  [unwired: 1 in, 2 out]
              n188 = Not Equal?(x=w341, y="none") -> (x != y?=w343:bool)
              n189 = Select(t=w342, s=w343, f=w341) -> (s? t:f=w340:string)
              n190 = Insert Into Array(array=w347, index=w349, new element=w340) -> (w348:string[])
            }
            n191 = property on="Stim protocols" class="Ring (strict)"("Strings []"=w334) -> ()  [unwired: 2 in, 2 out]
          }
        }
        n192 = local write "Current mice"(w328) -> ()
        n193 = local write "Enable stim."(TRUE ("Enable stim.")) -> ()
        n194 = local write "Stim. prot 2"(w306) -> ()
        n195 = local write "Stim. prot 3"(w306) -> ()
        n196 = local write "Stim. prot 4"(w306) -> ()
        n197 = local write "Stim. prot 5"(w306) -> ()
        n198 = local write "Mask prot 2"(w306) -> ()
        n199 = local write "Mask prot 3"(w306) -> ()
        n200 = local write "Mask prot 4"(w306) -> ()
        n201 = local write "Mask prot 5"(w306) -> ()
        n202 = local read "settings folder"() -> (w300:path)
        n203 = local write "Mask prot command"(w304) -> ()
        n204 = local write "Stim prot command"(w304) -> ()
        n205 = property on="Stop recording" class="Bool (strict)"("DisabledEnum"=T7."Disabled" ("Disabled")) -> ()  [unwired: 2 in, 2 out]
        n206 = Build Path(base path=w300, name or relative path="Last calibration.txt") -> (appended path=w298:path)
        n207 = Open/Create/Replace File(file path (use dialog)=w298, operation (0:open)=T11."open", access (0:read/write)=enum16{"read/write", "read-only", "write-only"}."read-only") -> (refnum out=w318:refnum<file>)  [unwired: 3 in, 2 out]
        n208 = Read from Text File(file (use dialog)=w318) -> (refnum out=w319:refnum<file>, text=w320:string)  [unwired: 3 in, 2 out]
        n209 = local write "Last calibration"(w320) -> ()
        n210 = Match Pattern(string=w320, regular expression=" ul") -> (before substring=w322:string)  [unwired: 1 in, 3 out]
        n211 = Match Pattern(string=w320, regular expression="ul / ") -> (after substring=w321:string)  [unwired: 1 in, 3 out]
        n212 = Close File(refnum=w319) -> ()  [unwired: 1 in, 2 out]
        n213 = Fract/Exp String To Number(string=w322) -> (number=w323:dbl)  [unwired: 3 in, 1 out]
        "Last saved reward size" <- w323
        n214 = Match Pattern(string=w321, regular expression=" ms ") -> (before substring=w324:string)  [unwired: 1 in, 3 out]
        n215 = local write "Reward size (ul)"(w323) -> ()
        n216 = Decimal String To Number(string=w324) -> (number=w325:i32)  [unwired: 2 in, 1 out]
        n217 = local write "Valve open dur. (ms)"(w325) -> ()
      }
      frame "Idle" {
        w373 = string[] []
        w387 = enum32{"0", "1", "2", "3", "4"}."1" ("Tab Control")
        w365 = u16 0 items=["none"] ("Stim. prot 1")
        w408 = u16[] []
        w379 = u16 0 items=["none"] ("Stim. prot 1")
        w409 = u16[] []
        w451 = 1 ("length")
        w430 = T7."Enabled" ("Disabled")
        # "Save reward calibration data"
        # "Select mouse from the current list of mice"
        n218 = local read "stim. num. 2"() -> (w415:u16)
        n219 = local read "stim. num. 3"() -> (w414:u16)
        n220 = local read "stim. num. 4"() -> (w413:u16)
        n221 = local read "stim. num. 5"() -> (w412:u16)
        n222 = stacked-sequence {
          seq-local: ["Stim protocols" _] -> [_ w531]
          seq-local: [w474 _] -> [_ w554]
          tunnel: [_ w529] -> w425
          frame #0 {
            n223 = call "Is Value Changed.vim"("value"="Stim protocols") -> ("changed or first call?"=w476:bool)
            n224 = local read "protocol array"() -> (w474:string[][])
            n225 = case shown="True" w476 {
              tunnel: w474 -> [_ w480]
              tunnel: "Stim protocols" -> [_ w478]
              frame False {
              }
              frame True {
                n226 = Index Array(array=w480, index (row)=w478, index (col)=2 ("disabled index (col)")) -> (element=w486:string)
                n227 = property on="Stim type" class="Ring (strict)"() -> ("StringsAndValues[]"=w489:T15)  [unwired: 2 in, 2 out]
                n228 = Index Array(array=w480, index (row)=w478, index (col)=0 ("disabled index (col)")) -> (element=w491:string)
                n229 = Index Array(array=w480, index (row)=w478, index (col)=1 ("disabled index (col)")) -> (element=w488:string)
                n230 = Index Array(array=w480, index (row)=w478, index (col)=4 ("disabled index (col)")) -> (element=w479:string)
                n231 = Index Array(array=w480, index (row)=w478, index (col)=3 ("disabled index (col)")) -> (element=w495:string)
                n232 = Match Pattern(string=w486, regular expression="to ") -> (after substring=w487:string)  [unwired: 1 in, 3 out]
                n233 = Match Pattern(string=w488, regular expression="from ") -> (after substring=w501:string)  [unwired: 1 in, 3 out]
                n234 = Not Equal?(x=w487, y="rew") -> (x != y?=w500:bool)
                n235 = Match Pattern(string=w495, regular expression=" int. ") -> (after substring=w494:string)  [unwired: 1 in, 3 out]
                n236 = Not Equal?(x=w501, y="rew") -> (x != y?=w502:bool)
                n237 = Match Pattern(string=w479, regular expression=" duty cycle. ") -> (after substring=w484:string)  [unwired: 1 in, 3 out]
                n238 = Match Pattern(string=w494, regular expression=" %  ") -> (before substring=w493:string)  [unwired: 1 in, 3 out]
                n239 = Match Pattern(string=w484, regular expression=" %  ") -> (before substring=w485:string)  [unwired: 1 in, 3 out]
                n240 = case shown="True" w500 {
                  tunnel: w487 -> [_ w519]
                  frame False {
                    n241 = local write "stop (cm)"(0 ("start (cm)")) -> ()
                    n242 = local write "to reward"(TRUE ("from reward")) -> ()
                  }
                  frame True {
                    n243 = local write "to reward"(FALSE ("from reward")) -> ()
                    n244 = Decimal String To Number(string=w519) -> (number=w518:i32)  [unwired: 2 in, 1 out]
                    n245 = local write "stop (cm)"(w518) -> ()
                  }
                }
                n246 = case shown="True" w502 {
                  tunnel: w501 -> [_ w524]
                  frame False {
                    n247 = local write "from reward"(TRUE ("from reward")) -> ()
                    n248 = local write "start (cm)"(0 ("start (cm)")) -> ()
                  }
                  frame True {
                    n249 = Decimal String To Number(string=w524) -> (number=w523:i32)  [unwired: 2 in, 1 out]
                    n250 = local write "from reward"(FALSE ("from reward")) -> ()
                    n251 = local write "start (cm)"(w523) -> ()
                  }
                }
                n252 = Array Size(array=w489) -> (size(s)=w492:i32)
                n253 = for {
                  N: w492 -> [_]
                  tunnel: w491 -> [w511]
                  tunnel: w489 -> [w510] mode=indexing
                  n254 = Unbundle(w510) -> ("String"=w509:string, "Value"=w513:u16)
                  n255 = Equal?(x=w511, y=w509) -> (x = y?=w512:bool)
                  n256 = case shown="True" w512 {
                    tunnel: w513 -> [_ w514]
                    frame False {
                    }
                    frame True {
                      n257 = local write "Stim type"(w514) -> ()
                    }
                  }
                }
                n258 = Decimal String To Number(string=w485) -> (number=w477:i32)  [unwired: 2 in, 1 out]
                n259 = Decimal String To Number(string=w493) -> (number=w490:i32)  [unwired: 2 in, 1 out]
                n260 = local write "Intensity (%)"(w490) -> ()
                n261 = local write "Duty cycle (%)"(w477) -> ()
              }
            }
          }
          frame #1 {
            w526 = "" ("new element/subarray")
            w528 = 0 ("index (row)")
            n262 = case shown="False" "to reward" {
              tunnel: "stop (cm)" -> [w589 _]
              tunnel: [w588 " to rew"] -> w569
              frame False {
                n263 = Number To Decimal String(number=w589) -> (decimal integer string=w591:string)  [unwired: 1 in]
                n264 = Concatenate Strings(" to " ("string"), w591) -> (w588:string)
                n265 = property on="stop (cm)" class="DigNum (strict)"("DisabledEnum"=T7."Enabled" ("Disabled")) -> ()  [unwired: 2 in, 2 out]
              }
              frame True {
                n266 = property on="stop (cm)" class="DigNum (strict)"("DisabledEnum"=T7."Disabled and Grayed Out" ("Disabled")) -> ()  [unwired: 2 in, 2 out]
              }
            }
            n267 = Number To Decimal String(number="Duty cycle (%)") -> (decimal integer string=w537:string)  [unwired: 1 in]
            n268 = case shown="False" "from reward" {
              tunnel: "start (cm)" -> [_ w586]
              tunnel: [" from rew" w583] -> w568
              frame True {
                n269 = property on="start (cm)" class="DigNum (strict)"("DisabledEnum"=T7."Disabled and Grayed Out" ("Disabled")) -> ()  [unwired: 2 in, 2 out]
              }
              frame False {
                n270 = Number To Decimal String(number=w586) -> (decimal integer string=w584:string)  [unwired: 1 in]
                n271 = property on="start (cm)" class="DigNum (strict)"("DisabledEnum"=T7."Enabled" ("Disabled")) -> ()  [unwired: 2 in, 2 out]
                n272 = Concatenate Strings(" from " ("string"), w584) -> (w583:string)
              }
            }
            n273 = Number To Decimal String(number="Intensity (%)") -> (decimal integer string=w559:string)  [unwired: 1 in]
            n274 = property on="Stim type" class="Ring (strict)"() -> ("RingText.Text"=w540:string)  [unwired: 2 in, 2 out]
            n275 = Concatenate Strings(" int. " ("string"), w559, " %" ("string")) -> (w570:string)
            n276 = Concatenate Strings(" duty cycle " ("string"), w537, " %" ("string")) -> (w533:string)
            n277 = Not Equal?(x=w540, y="none") -> (x != y?=w541:bool)
            n278 = case shown="True" w541 {
              tunnel: w570 -> [w576 _]
              tunnel: w569 -> [w575 _]
              tunnel: w568 -> [w574 _]
              tunnel: [w573 w579] -> w564
              tunnel: w540 -> [w572 w578]
              tunnel: w533 -> [w571 _]
              frame True {
                n279 = Build Array(w572, w574, w575, w576, w571) -> (w573:string[])
              }
              frame False {
                w577 = "" ("element")
                n280 = Build Array(w578, w577, w577, w577, w577) -> (w579:string[])
              }
            }
            n281 = Replace Array Subset(array=w554, new element=w540, index (row)=w531, index (col)=0 ("disabled index (col)")) -> (w565:string[][])
            n282 = Replace Array Subset(array=w565, new element=w568, index (row)=w531, index (col)=1 ("disabled index (col)")) -> (w566:string[][])
            n283 = Replace Array Subset(array=w566, new element=w569, index (row)=w531, index (col)=2 ("disabled index (col)")) -> (w567:string[][])
            n284 = Replace Array Subset(array=w567, new element=w570, index (row)=w531, index (col)=3 ("disabled index (col)")) -> (w532:string[][])
            n285 = Replace Array Subset(array=w532, new element=w533, index (row)=w531, index (col)=4 ("disabled index (col)")) -> (w534:string[][])
            n286 = Replace Array Subset(array=w534, new element="none" ("new element/subarray"), index (row)=w528, index (col)=0 ("disabled index (col)")) -> (w547:string[][])
            n287 = Replace Array Subset(array=w547, new element=w526, index (row)=w528, index (col)=1 ("disabled index (col)")) -> (w546:string[][])
            n288 = Replace Array Subset(array=w546, new element=w526, index (row)=w528, index (col)=2 ("disabled index (col)")) -> (w545:string[][])
            n289 = Replace Array Subset(array=w545, new element=w526, index (row)=w528, index (col)=3 ("disabled index (col)")) -> (w530:string[][])
            n290 = Replace Array Subset(array=w530, new element=w526, index (row)=w528, index (col)=4 ("disabled index (col)")) -> (w529:string[][])
            n291 = local write "protocol array"(w529) -> ()
            n292 = Concatenate Strings(w564) -> (w563:string)
            n293 = property on="Stim protocols" class="Ring (strict)"("RingText.Text"=w563) -> ()  [unwired: 2 in, 2 out]
          }
        }
        n294 = for {
          N: "Trial block" -> [_]
          shift-right: [w690] -> w427
          shift-left: i32[] [] -> [w689]
          i -> [w691]
          n295 = Insert Into Array(array=w689, index=w691, new element=w691) -> (w690:i32[])
        }
        n296 = Compound Arithmetic op=ADD(w415, w414, w413, w412) -> (w411:u16)
        n297 = Build Array(w379, "Stim. prot 2", "Stim. prot 3", "Stim. prot 4", "Stim. prot 5") -> (w374:u16[])
        n298 = for {
          N: "stim. num. 2" -> [_]
          tunnel: "Stim. prot 2" -> [w679]
          shift-right: [w678] -> w423
          shift-left: w409 -> [w677]
          i -> [w680]
          n299 = Insert Into Array(array=w677, index=w680, new element=w679) -> (w678:u16[])
        }
        n300 = for {
          N: "stim. num. 3" -> [_]
          tunnel: "Stim. prot 3" -> [w675]
          shift-right: [w674] -> w424
          shift-left: w409 -> [w673]
          i -> [w676]
          n301 = Insert Into Array(array=w673, index=w676, new element=w675) -> (w674:u16[])
        }
        n302 = for {
          N: "stim. num. 4" -> [_]
          tunnel: "Stim. prot 4" -> [w671]
          shift-right: [w670] -> w421
          shift-left: w409 -> [w669]
          i -> [w672]
          n303 = Insert Into Array(array=w669, index=w672, new element=w671) -> (w670:u16[])
        }
        n304 = for {
          N: "stim. num. 5" -> [_]
          tunnel: "Stim. prot 5" -> [w667]
          shift-right: [w666] -> w420
          shift-left: w409 -> [w665]
          i -> [w668]
          n305 = Insert Into Array(array=w665, index=w668, new element=w667) -> (w666:u16[])
        }
        n306 = Subtract(x="Trial block", y=w411) -> (x-y=w410:u16)
        "stim. num. 1" <- w410
        n307 = for {
          N: w410 -> [_]
          tunnel: w379 -> [w683]
          shift-right: [w682] -> w422
          shift-left: w409 -> [w681]
          i -> [w684]
          n308 = Insert Into Array(array=w681, index=w684, new element=w683) -> (w682:u16[])
        }
        n309 = local write "shuffled array"(w427) -> ()
        n310 = local read "mask. num. 2"() -> (w403:u16)
        n311 = local read "mask. num. 3"() -> (w402:u16)
        n312 = local read "mask. num. 4"() -> (w401:u16)
        n313 = local read "mask. num. 5"() -> (w400:u16)
        n314 = Build Array (concatenate)(w422, w423, w424, w421, w420) -> (w391:u16[])
        n315 = Compound Arithmetic op=ADD(w403, w402, w401, w400) -> (w399:u16)
        n316 = Build Array(w365, "Mask prot 2", "Mask prot 3", "Mask prot 4", "Mask prot 5") -> (w360:u16[])
        n317 = case shown="True" FALSE {
          frame False {
          }
          frame True {
            n318 = One Button Dialog(message="The sum of stimulated trials can lot exceed the denominator!!!") -> ()  [unwired: 1 in, 1 out]
          }
        }
        n319 = Subtract(x="Trial block", y=w399) -> (x-y=w397:u16)
        "mask. num. 1" <- w397
        n320 = for {
          N: "mask. num. 2" -> [_]
          tunnel: "Mask prot 2" -> [w659]
          shift-right: [w658] -> w395
          shift-left: w408 -> [w657]
          i -> [w660]
          n321 = Insert Into Array(array=w657, index=w660, new element=w659) -> (w658:u16[])
        }
        n322 = for {
          N: "mask. num. 3" -> [_]
          tunnel: "Mask prot 3" -> [w655]
          shift-right: [w654] -> w394
          shift-left: w408 -> [w653]
          i -> [w656]
          n323 = Insert Into Array(array=w653, index=w656, new element=w655) -> (w654:u16[])
        }
        n324 = for {
          N: "mask. num. 4" -> [_]
          tunnel: "Mask prot 4" -> [w651]
          shift-right: [w650] -> w393
          shift-left: w408 -> [w649]
          i -> [w652]
          n325 = Insert Into Array(array=w649, index=w652, new element=w651) -> (w650:u16[])
        }
        n326 = for {
          N: w397 -> [_]
          tunnel: w365 -> [w663]
          shift-right: [w662] -> w396
          shift-left: w408 -> [w661]
          i -> [w664]
          n327 = Insert Into Array(array=w661, index=w664, new element=w663) -> (w662:u16[])
        }
        n328 = for {
          N: "mask. num. 5" -> [_]
          tunnel: "Mask prot 5" -> [w647]
          shift-right: [w646] -> w392
          shift-left: w408 -> [w645]
          i -> [w648]
          n329 = Insert Into Array(array=w645, index=w648, new element=w647) -> (w646:u16[])
        }
        n330 = call "Is Value Changed.vim"("value"=w425) -> ("changed or first call?"=w426:bool)
        n331 = case shown="True" w426 {
          tunnel: w425 -> [_ w688]
          frame False {
          }
          frame True {
            n332 = local read "settings folder"() -> (w687:path)
            n333 = Build Path(base path=w687, name or relative path="Stimprotocols.txt") -> (appended path=w685:path)
            n334 = call-poly <vilib>:"Write Delimited Spreadsheet.vi"("file path (dialog if empty)"=w685, "2D data"=w688) -> ()  [unwired: 12 in, 2 out]
          }
        }
        n335 = Build Array (concatenate)(w396, w395, w394, w393, w392) -> (w390:u16[])
        n336 = Build Array(w391, w390) -> (→"Trial types":u16[][])
        n337 = local read "mask. num. 1"() -> (w371:u16)
        n338 = local read "mask. num. 2"() -> (w370:u16)
        n339 = local read "mask. num. 3"() -> (w369:u16)
        n340 = local read "mask. num. 4"() -> (w368:u16)
        n341 = local read "mask. num. 5"() -> (w367:u16)
        n342 = local read "stim. num. 1"() -> (w384:u16)
        n343 = local read "stim. num. 2"() -> (w383:u16)
        n344 = local read "stim. num. 3"() -> (w382:u16)
        n345 = local read "stim. num. 4"() -> (w381:u16)
        n346 = local read "stim. num. 5"() -> (w380:u16)
        n347 = local read "Last saved reward size"() -> (w440:dbl)
        n348 = Build Array(w384, w383, w382, w381, w380) -> (w372:u16[])
        n349 = Build Array(w371, w370, w369, w368, w367) -> (w366:u16[])
        n350 = Array Size(array=w372) -> (size(s)=w386:i32)
        n351 = for {
          N: w386 -> [_]
          tunnel: w360 -> [w608] mode=indexing
          shift-right: [w604] -> w357
          shift-left: w373 -> [w603]
          tunnel: w366 -> [w602] mode=indexing
          tunnel: w374 -> [w596] mode=indexing
          shift-right: [w600] -> w359
          shift-left: w373 -> [w595]
          tunnel: w372 -> [w601] mode=indexing
          i -> [w594]
          n352 = Greater?(x=w602, y=0.0) -> (0:w607:bool)
          n353 = Greater?(x=w601, y=0.0) -> (0:w597:bool)
          n354 = case shown="True" w607 {
            tunnel: w608 -> [_ w643]
            tunnel: w602 -> [_ w642]
            tunnel: ["" w630] -> w605
            frame False {
            }
            frame True {
              n355 = property on="Stim protocols" class="Ring (strict)"() -> ("StringsAndValues[]"=w644:T15)  [unwired: 2 in, 2 out]
              n356 = local read "Trial block"() -> (w635:u16)
              n357 = Number To Decimal String(number=w642) -> (decimal integer string=w637:string)  [unwired: 1 in]
              n358 = Number To Decimal String(number=w635) -> (decimal integer string=w634:string)  [unwired: 1 in]
              n359 = Index Array(array=w644, index=w643) -> (element=w641:cluster{"String":string, "Value":u16})
              n360 = Concatenate Strings(w637, "/" ("string"), w634) -> (w633:string)
              n361 = Unbundle(w641) -> ("String"=w629:string, "Value"=w640:u16)
              n362 = Number To Decimal String(number=w640) -> (decimal integer string=w639:string)  [unwired: 1 in]
              n363 = Match Pattern(string=w629, regular expression="int. ") -> (before substring=w627:string)  [unwired: 1 in, 3 out]
              n364 = Concatenate Strings(w639, ": " ("string"), w633, " " ("string"), w627, "\n" ("string")) -> (w630:string)
            }
          }
          n365 = case shown="True" w597 {
            tunnel: w596 -> [_ w624]
            tunnel: w601 -> [_ w623]
            tunnel: ["" w610] -> w599
            frame False {
            }
            frame True {
              n366 = property on="Stim protocols" class="Ring (strict)"() -> ("StringsAndValues[]"=w625:T15)  [unwired: 2 in, 2 out]
              n367 = local read "Trial block"() -> (w616:u16)
              n368 = Number To Decimal String(number=w623) -> (decimal integer string=w618:string)  [unwired: 1 in]
              n369 = Index Array(array=w625, index=w624) -> (element=w622:cluster{"String":string, "Value":u16})
              n370 = Number To Decimal String(number=w616) -> (decimal integer string=w615:string)  [unwired: 1 in]
              n371 = Unbundle(w622) -> ("String"=w612:string, "Value"=w621:u16)
              n372 = Concatenate Strings(w618, "/" ("string"), w615) -> (w614:string)
              n373 = Number To Decimal String(number=w621) -> (decimal integer string=w620:string)  [unwired: 1 in]
              n374 = Concatenate Strings(w620, ": " ("string"), w614, " " ("string"), w612, "\n" ("string")) -> (w610:string)
            }
          }
          n375 = Insert Into Array(array=w603, index=w594, new element=w605) -> (w604:string[])
          n376 = Insert Into Array(array=w595, index=w594, new element=w599) -> (w600:string[])
        }
        n377 = Not Equal?(x="Reward size (ul)", y=w440) -> (x != y?=w456:bool)
        n378 = case shown="True" w456 {
          tunnel: "Reward size (ul)" -> [_ w703]
          frame False {
          }
          frame True {
            n379 = local write "Last saved reward size"(w703) -> ()
            n380 = local read "settings folder"() -> (w702:path)
            n381 = local read "Valve open dur. (ms)"() -> (w711:u32)
            n382 = local read "Date"() -> (w706:string)
            n383 = Build Path(base path=w702, name or relative path="Last calibration.txt") -> (appended path=w700:path)
            n384 = Number To Decimal String(number=w711) -> (decimal integer string=w712:string)  [unwired: 1 in]
            n385 = Number To Fractional String(number=w703, precision (6)=i16 2) -> (F-format string=w714:string)  [unwired: 2 in]
            n386 = Concatenate Strings(w714, " ul / " ("string"), w712, " ms " ("string"), " (" ("string"), w706, ")" ("string")) -> (w708:string)
            "Last calibration" <- w708
            n387 = Open/Create/Replace File(file path (use dialog)=w700, operation (0:open)=T11."open") -> (refnum out=w715:refnum<file>)  [unwired: 4 in, 2 out]
            n388 = Write to Text File(file (use dialog)=w715, text=w708) -> (refnum out=w716:refnum<file>)  [unwired: 2 in, 2 out]
            n389 = Close File(refnum=w716) -> ()  [unwired: 1 in, 2 out]
          }
        }
        n390 = property on="Stim protocols" class="Ring (strict)"() -> ("Strings []"=w388:string[])  [unwired: 2 in, 2 out]
        n391 = property on="Stim. prot 1" class="Ring (strict)"("Strings []"=w388) -> ()  [unwired: 2 in, 2 out]
        n392 = property on="Stim. prot 2" class="Ring (strict)"("Strings []"=w388) -> ()  [unwired: 2 in, 2 out]
        n393 = property on="Stim. prot 3" class="Ring (strict)"("Strings []"=w388) -> ()  [unwired: 2 in, 2 out]
        n394 = property on="Stim. prot 4" class="Ring (strict)"("Strings []"=w388) -> ()  [unwired: 2 in, 2 out]
        n395 = property on="Stim. prot 5" class="Ring (strict)"("Strings []"=w388) -> ()  [unwired: 2 in, 2 out]
        n396 = local write "Primary masking light"("Primary masking light") -> ()
        n397 = case shown="0, Default" "Location of reward zone" {
          tunnel: [w727 w730 w735 w740 w745] -> w466
          tunnel: [w725 w731 w736 w741 w746] -> w465
          frame 0, Default {
            w727 = 230.0 ("Corridor length")
            n398 = local write "reward zone start"(80.0 ("reward zone start")) -> ()
            n399 = local write "reward zone end"(90.0 ("reward zone end")) -> ()
            n400 = Subtract(x=w727, y=140.0) -> (x-y=w725:dbl)
          }
          frame 1 {
            w730 = 270.0 ("Corridor length")
            n401 = local write "reward zone start"(120.0 ("reward zone start")) -> ()
            n402 = local write "reward zone end"(130.0 ("reward zone end")) -> ()
            n403 = Subtract(x=w730, y=140.0) -> (x-y=w731:dbl)
          }
          frame 2 {
            w735 = 330.0 ("Corridor length")
            n404 = local write "reward zone start"(180.0 ("reward zone start")) -> ()
            n405 = local write "reward zone end"(190.0 ("reward zone end")) -> ()
            n406 = Subtract(x=w735, y=140.0) -> (x-y=w736:dbl)
          }
          frame 3 {
            w740 = 420.0 ("Corridor length")
            n407 = local write "reward zone start"(270.0 ("reward zone start")) -> ()
            n408 = local write "reward zone end"(280.0 ("reward zone end")) -> ()
            n409 = Subtract(x=w740, y=140.0) -> (x-y=w741:dbl)
          }
          frame 4 {
            w745 = 550.0 ("Corridor length")
            n410 = local write "reward zone start"(400.0 ("reward zone start")) -> ()
            n411 = local write "reward zone end"(410.0 ("reward zone end")) -> ()
            n412 = Subtract(x=w745, y=140.0) -> (x-y=w746:dbl)
          }
        }
        n413 = property on="Mask prot 1" class="Ring (strict)"("Strings []"=w388) -> ()  [unwired: 2 in, 2 out]
        n414 = property on="Mask prot 2" class="Ring (strict)"("Strings []"=w388) -> ()  [unwired: 2 in, 2 out]
        n415 = property on="Mask prot 3" class="Ring (strict)"("Strings []"=w388) -> ()  [unwired: 2 in, 2 out]
        n416 = property on="Mask prot 4" class="Ring (strict)"("Strings []"=w388) -> ()  [unwired: 2 in, 2 out]
        n417 = property on="Mask prot 5" class="Ring (strict)"("Strings []"=w388) -> ()  [unwired: 2 in, 2 out]
        n418 = local read "Current mice"() -> (w454:string[][])
        n419 = local write "Run experiment"(FALSE ("Record")) -> ()
        n420 = Array Subset(array=w454, index (row)="Scrollbar", length (row)=w451, index (col)=0 ("index 2"), length (col)=w451) -> (w461:string[][])
        n421 = Array Subset(array=w454, index (row)="Scrollbar", length (row)=w451, index (col)=1 ("index 2"), length (col)=w451) -> (w458:string[][])
        n422 = Array Subset(array=w454, index (row)="Scrollbar", length (row)=w451, index (col)=2 ("index"), length (col)=w451) -> (w450:string[][])
        n423 = local write "Corridor length"(w466) -> ()
        n424 = property class="Slide (strict)"("Scale.Maximum"=w465) -> ()  [unwired: 2 in, 2 out]
        n425 = property on="Top Graph" class="XYGraph (strict)"("XScale.Maximum"=w465) -> ()  [unwired: 2 in, 2 out]
        n426 = property on="Bottom Graph" class="XYGraph (strict)"("XScale.Maximum"=w465) -> ()  [unwired: 2 in, 2 out]
        n427 = Concatenate Strings(w450) -> (w448:string)
        n428 = Format Date/Time String(time format string (%c)="%Y.%m.%d") -> (date/time string=→"Date":string)  [unwired: 2 in]
        n429 = Fract/Exp String To Number(string=w448) -> (number=w447:dbl)  [unwired: 3 in, 1 out]
        "Original weight" <- w447
        n430 = local read "Wheel circumference"() -> (w434:dbl)
        n431 = Concatenate Strings("\nOptical stimulation protocol:\n", w359, "\nMasking protocol (secondary masking light):\n", w357) -> (→"Stimulus protocol":string)
        n432 = local read "Reward freq. (cm)"() -> (w351:dbl)
        n433 = Concatenate Strings(w461, string[][] [["-"]] ("string"), w458) -> (w438:string)
        "Mouse name" <- w438
        n434 = Divide(x="Weight", y=w447) -> (x/y=w445:dbl)
        n435 = case shown="True" "Edit mouse list" {
          frame False {
            n436 = property on="Current mice" class="Arr (strict)"("DisabledEnum"=T7."Disabled and Grayed Out" ("Disabled")) -> ()  [unwired: 2 in, 2 out]
          }
          frame True {
            n437 = local read "settings folder"() -> (w720:path)
            n438 = property on="Current mice" class="Arr (strict)"("DisabledEnum"=T7."Enabled" ("Disabled")) -> ()  [unwired: 2 in, 2 out]
            n439 = Build Path(base path=w720, name or relative path="List of mice.txt") -> (appended path=w718:path)
            n440 = call-poly <vilib>:"Write Delimited Spreadsheet.vi"("file path (dialog if empty)"=w718, "2D data"="Current mice") -> ()  [unwired: 12 in, 2 out]
          }
        }
        n441 = Multiply(x=100.0, y=w445) -> (x*y=→"%":dbl)
        n442 = local read "Exit program"() -> (w471:bool)
        n443 = property on="Primary masking light" class="Enum (strict)"() -> ("RingText.Text"=w353:string)  [unwired: 2 in, 2 out]
        n444 = local read "Mate"() -> (w435:bool)
        n445 = call "Is Value Changed.vim"("value"=w438) -> ("changed or first call?"=w437:bool)
        n446 = local write "Record"("Record Button") -> ()
        n447 = case shown="True" "Record Button" {
          frame False {
          }
          frame True {
            n448 = local read "Unique ID"() -> (w696:i8)
            n449 = Increment(x=w696) -> (x+1=w697:i8)
            n450 = local write "Unique ID"(w697) -> ()
          }
        }
        n451 = Or(x="Start recording", y="Record Button") -> (x .or. y?=w469:bool)
        n452 = case shown="True" w435 {
          tunnel: [w692 w695] -> w436
          tunnel: w351 -> [_ w694]
          tunnel: w434 -> [w692 _]
          frame False {
          }
          frame True {
            n453 = Add(x=w694, y=40.0) -> (x+y=w695:dbl)
          }
        }
        n454 = case shown="True" w437 {
          frame False {
          }
          frame True {
            n455 = local write "Reset water count"(TRUE ("Reset water count")) -> ()
            n456 = local write "Unique ID"(i8 -1 ("Unique ID")) -> ()
          }
        }
        n457 = case shown="False" w471 {
          frame False {
            n458 = flat-sequence {
              frame #0 {
                n459 = Wait (ms)(milliseconds to wait=u32 50) -> ()  [unwired: 1 out]
              }
              frame #1 {
                n460 = local write "Write"(TRUE ("Write")) -> ()
              }
            }
            n461 = local write "read"(FALSE ("read")) -> ()
          }
          frame True {
            n462 = stacked-sequence {
              frame #0 {
                n463 = local write "Encoder count"(100.0 ("Encoder count")) -> ()
                n464 = Wait (ms)(milliseconds to wait=u32 10) -> ()  [unwired: 1 out]
              }
              frame #1 {
                n465 = local write "Encoder count"(110.0 ("Encoder count")) -> ()
                n466 = Wait (ms)(milliseconds to wait=u32 10) -> ()  [unwired: 1 out]
              }
              frame #2 {
                n467 = local write "read"(FALSE ("read")) -> ()
                n468 = local write "Stop Unity"(TRUE ("Exit")) -> ()
              }
            }
            n469 = local read "Write loop stopped"() -> (w751:bool)
            n470 = case shown="True" w751 {
              frame False {
              }
              frame True {
                n471 = local write "Exit program"(FALSE ("Exit program")) -> ()
                n472 = local write "Exit"(TRUE ("Exit")) -> ()
              }
            }
          }
        }
        n473 = property on="Location of reward zone" class="Ring (strict)"("DisabledEnum"=w430) -> ()  [unwired: 2 in, 2 out]
        n474 = property on="Primary masking light" class="Enum (strict)"("DisabledEnum"=w430) -> ()  [unwired: 2 in, 2 out]
        n475 = local write "Valve open dur. (ms)"("Valve open dur. (ms)") -> ()
        n476 = Concatenate Strings("Primary masking light: ", w353) -> (→"Masking light prot":string)
        n477 = property on="Wheel position graph" class="XYGraph (strict)"("XScale.Maximum"=w436) -> ()  [unwired: 2 in, 2 out]
        n478 = local write "Comment"("Comment") -> ()
        n479 = local write "2P imaging"("2P imaging: NO" ("2P imaging")) -> ()
        n480 = local write "msg tag"("str," ("msg tag")) -> ()
        n481 = Select(t=T12."Init recording " ("main program"), s=w469, f=T12."Idle" ("main program")) -> (s? t:f=w468:T12)
        "Tab Control" <- w387
        "Tab Control 2" <- w387
        "Stim. prot 1" <- w379
        "Mask prot 1" <- w365
      }
      frame "Init recording " {
        w761 = T7."Disabled" ("Disabled")
        w765 = u16 0 ("Mask prot command")
        w766 = 0 ("All trials")
        w770 = T7."Disabled and Grayed Out" ("Disabled")
        n482 = local read "reward zone end"() -> (w764:dbl)
        n483 = local write "Edit mouse list"(FALSE ("Edit mouse list")) -> ()
        n484 = Decrement(x=w764) -> (x-1=w763:dbl)
        n485 = local write "Run experiment"(TRUE ("record")) -> ()
        n486 = local write "Write"(TRUE ("Write")) -> ()
        n487 = local write "read"(TRUE ("read")) -> ()
        n488 = local write "Random reward"(FALSE ("Random reward")) -> ()
        n489 = local write "select trial"(TRUE ("Randomize")) -> ()
        n490 = local write "Unity position:"(w763) -> ()
        n491 = local read "VR Mode"() -> (w775:bool)
        n492 = local read "Mate"() -> (w773:bool)
        n493 = property on="Location of reward zone" class="Ring (strict)"("DisabledEnum"=w770) -> ()  [unwired: 2 in, 2 out]
        n494 = property on="Primary masking light" class="Enum (strict)"("DisabledEnum"=w770) -> ()  [unwired: 2 in, 2 out]
        n495 = Not(x=w775) -> (.not. x?=w774:bool)
        n496 = And(x=w773, y=w774) -> (x .and. y?=w772:bool)
        n497 = Not(x=w772) -> (.not. x?=w771:bool)
        n498 = local read "VR Mode"() -> (w776:bool)
        n499 = case shown="False" w771 {
          frame False {
            n500 = local write "Reward zone"(FALSE ("Reward zone")) -> ()
          }
          frame True {
            n501 = local write "Reward zone"(TRUE ("Reward zone")) -> ()
          }
        }
        n502 = case shown="False" w776 {
          frame False {
            n503 = local write "All trials"(-1 ("All trials")) -> ()
          }
          frame True {
            n504 = local write "All trials"(0 ("All trials")) -> ()
          }
        }
        n505 = local write "Mask prot command"(w765) -> ()
        n506 = local write "Stim prot command"(w765) -> ()
        n507 = local write "Prev. rew. pos."(0.0 ("Prev. rew. pos.")) -> ()
        n508 = local write "Active licking"(TRUE ("Active licking")) -> ()
        n509 = local write "Start light stim"(FALSE ("Start light stim")) -> ()
        n510 = local write "miss trial"(FALSE ("miss trial")) -> ()
        n511 = local write "Water count"(0 ("Water count")) -> ()
        n512 = local write "Repetition"(2 ("Repetition")) -> ()
        n513 = local write "Hit trials ctrl."(w766) -> ()
        n514 = local write "Hit trials"(w766) -> ()
        n515 = local write "Hit trials stim."(w766) -> ()
        n516 = local write "Ctrl. count"(w766) -> ()
        n517 = local write "Stim. count"(w766) -> ()
        n518 = local write "Trial type array"(i16[][] [] ("Trial type array")) -> ()
        n519 = local write "Reward given"(TRUE ("Reward given")) -> ()
        n520 = local write "Hybrid licking"(TRUE ("Hybrid licking")) -> ()
        n521 = local write "Trial counted"(FALSE ("Trial counted")) -> ()
        n522 = local write "Shuffle"(FALSE ("Shuffle")) -> ()
        n523 = disable-structure shown="Disabled" {
          frame Disabled {
            n524 = local read "Trial types"() -> (w808:u16[][])
            n525 = local read item#-1() -> ()  [unwired: 1 out]
            n526 = Index Array(array=w808, index (row)=1) -> (element=w810:u16[])  [unwired: 1 in]
            n527 = Add Array Elements(numeric array=w810) -> (sum=w809:u16)
            n528 = Greater?(x=w809, y=i16 0) -> (0:w802:bool)
            n529 = Equal?(y=T13."None" ("Stimulus protocol")) -> (x = y?=w803:bool)  [unwired: 1 in]
            n530 = And(x=w802, y=w803) -> (x .and. y?=w804:bool)
            n531 = case shown="True" w804 {
              frame False {
              }
              frame True {
                n532 = One Button Dialog(message="No stimulus protocol has been selected!") -> ()  [unwired: 1 in, 1 out]
              }
            }
          }
          frame Enabled {
          }
        }
        n533 = local read "SciScan start"() -> (w786:refnum<k21>)
        n534 = local read "Location of reward zone"() -> (w767:T4)
        n535 = local write "SciScan"(FALSE ("SciScan")) -> ()
        n536 = call <vilib>:"DAQmx Start Task.vi"("task/channels in"=w786) -> ("task out"=w787:refnum<k21>, "error out"=w784:errorcluster)  [unwired: 13 in]
        n537 = local write "offset tag"("0," ("offset tag")) -> ()
        n538 = call-poly <vilib>:"DAQmx Write.vi"("task/channels in"=w787, "data"=FALSE, "error in"=w784) -> ("task out"=w783:refnum<k21>)  [unwired: 10 in, 2 out]
        n539 = disable-structure shown="Disabled" {
          frame Disabled {
            n540 = call <vilib>:"DAQmx Stop Task.vi"() -> ()  [unwired: 14 in, 2 out]
          }
          frame Enabled {
          }
        }
        n541 = case shown="4" w767 {
          frame 0, Default {
            n542 = local write "msg tag"("c1") -> ()
          }
          frame 1 {
            n543 = local write "msg tag"("c2") -> ()
          }
          frame 2 {
            n544 = local write "msg tag"("c3") -> ()
          }
          frame 3 {
            n545 = local write "msg tag"("c4") -> ()
          }
          frame 4 {
            n546 = local write "msg tag"("c5") -> ()
          }
        }
        n547 = property on="Record Button" class="Bool (strict)"("DisabledEnum"=w761) -> ()  [unwired: 2 in, 2 out]
        n548 = property on="Stop recording" class="Bool (strict)"("DisabledEnum"=T7."Enabled" ("Disabled")) -> ()  [unwired: 2 in, 2 out]
        n549 = local write "SciScan start"(w783) -> ()
        n550 = property on="Start recording" class="Bool (strict)"("DisabledEnum"=w761) -> ()  [unwired: 2 in, 2 out]
        n551 = local read "VR Mode"() -> (w790:bool)
        n552 = Select(t=T12."Record VR" ("main program"), s=w790, f=T12."Record" ("main program")) -> (s? t:f=w792:T12)
      }
      frame "Stop Recording" {
        w826 = T7."Enabled" ("Disabled")
        n553 = local read "VR Mode"() -> (w831:bool)
        n554 = local write "Run experiment"(FALSE ("Record")) -> ()
        n555 = local write "Start light stim"(FALSE ("Start light stim")) -> ()
        n556 = local write "Timed reward (s)"(u32 0 ("Timed reward (s)")) -> ()
        n557 = local write "Start recording"(FALSE ("Start recording")) -> ()
        n558 = local write "Record Button"(FALSE ("Record Button")) -> ()
        n559 = case shown="True" w831 {
          frame False {
          }
          frame True {
            # "Wait for writing stimulus protocol, etc. to in lab book file"
            n560 = flat-sequence {
              frame #0 {
                n561 = Wait (ms)(milliseconds to wait=u32 100) -> ()  [unwired: 1 out]
              }
              frame #1 {
                n562 = local write "Primary masking light"(T14."None" ("Masking light")) -> ()
              }
            }
          }
        }
        n563 = local read "SciScan start"() -> (w822:refnum<k21>)
        n564 = local write "Frame signal indicator"(FALSE ("Frame signal")) -> ()
        n565 = local write "SciScan"(FALSE ("SciScan")) -> ()
        n566 = case shown="True" "Extra stop triggers" {
          tunnel: w822 -> [w838 w845]
          tunnel: [w837 w840] -> w821
          frame False {
            n567 = call-poly <vilib>:"DAQmx Write.vi"("task/channels in"=w838, "data"=FALSE) -> ("task out"=w837:refnum<k21>)  [unwired: 11 in, 2 out]
          }
          frame True {
            n568 = flat-sequence {
              tunnel: w845 -> [w847]
              tunnel: [w846] -> w844
              tunnel: w844 -> [w851]
              tunnel: [w850] -> w843
              tunnel: w843 -> [w855]
              tunnel: [w854] -> w842
              tunnel: w842 -> [w859]
              tunnel: [w858] -> w841
              tunnel: w841 -> [w864]
              tunnel: [w863] -> w840
              frame #0 {
                n569 = call-poly <vilib>:"DAQmx Write.vi"("task/channels in"=w847, "data"=FALSE) -> ("task out"=w846:refnum<k21>)  [unwired: 11 in, 2 out]
                n570 = Wait (ms)(milliseconds to wait=u32 20) -> ()  [unwired: 1 out]
              }
              frame #1 {
                n571 = call-poly <vilib>:"DAQmx Write.vi"("task/channels in"=w851, "data"=TRUE) -> ("task out"=w850:refnum<k21>)  [unwired: 11 in, 2 out]
                n572 = Wait (ms)(milliseconds to wait=u32 20) -> ()  [unwired: 1 out]
              }
              frame #2 {
                n573 = call-poly <vilib>:"DAQmx Write.vi"("task/channels in"=w855, "data"=FALSE) -> ("task out"=w854:refnum<k21>)  [unwired: 11 in, 2 out]
                n574 = Wait (ms)(milliseconds to wait=u32 50) -> ()  [unwired: 1 out]
              }
              frame #3 {
                n575 = call-poly <vilib>:"DAQmx Write.vi"("task/channels in"=w859, "data"=TRUE) -> ("task out"=w858:refnum<k21>)  [unwired: 11 in, 2 out]
                n576 = Wait (ms)(milliseconds to wait=u32 50) -> ()  [unwired: 1 out]
              }
              frame #4 {
                n577 = call-poly <vilib>:"DAQmx Write.vi"("task/channels in"=w864, "data"=FALSE) -> ("task out"=w863:refnum<k21>)  [unwired: 11 in, 2 out]
                n578 = Wait (ms)(milliseconds to wait=u32 10) -> ()  [unwired: 1 out]
              }
            }
          }
        }
        n579 = property on="Stop recording" class="Bool (strict)"("DisabledEnum"=T7."Disabled" ("Disabled")) -> ()  [unwired: 2 in, 2 out]
        n580 = property on="Record Button" class="Bool (strict)"("DisabledEnum"=w826) -> ()  [unwired: 2 in, 2 out]
        n581 = property on="Start recording" class="Bool (strict)"("DisabledEnum"=w826) -> ()  [unwired: 2 in, 2 out]
        n582 = Wait (ms)(milliseconds to wait=u32 100) -> ()  [unwired: 1 out]
        n583 = call <vilib>:"DAQmx Stop Task.vi"("task/channels in"=w821) -> ("task out"=w823:refnum<k21>)  [unwired: 13 in, 1 out]
        n584 = local write "SciScan start"(w823) -> ()
      }
      frame "Exit program" {
      }
      frame "Record" {
        # "only true if prev. diode pos. <15 cm and reward given changes"
        # "These events happen only once in a trial at the beginning: 10 cm after the diode signal \nand  min ~ 5cm after revard given"
        # "Calculate \"Hit trials\""
        # "These events happen only once in a trial at the second half: 100 cm after diode signal"
        n585 = disable-structure shown="Disabled" {
          frame Disabled {
            # "These events happen only once in a trial at the beginning: 10 cm after the diode signal \nand  min ~ 5cm after revard given"
            n586 = local read "Mate"() -> (w926:bool)
            n587 = case shown="False" w926 {
              tunnel: [w932 w933] -> w928
              frame True {
                n588 = local read "Prev. rew. pos."() -> (w932:dbl)
              }
              frame False {
                n589 = local read "prev. diode position"() -> (w933:dbl)
              }
            }
            n590 = local read "Trial counted"() -> (w931:bool)
            n591 = Not(x=w931) -> (.not. x?=w930:bool)
            n592 = call "Is Value Changed.vim"("value"=w928) -> ("changed or first call?"=w927:bool)
            n593 = And(x=w927, y=w930) -> (x .and. y?=w929:bool)
            n594 = case shown="True" w929 {
              frame False {
              }
              frame True {
                n595 = local read "All trials"() -> (w943:i32)
                n596 = local read "Trial type array"() -> (w940:i8[][])
                n597 = local read "Light ON"() -> (w939:bool)
                n598 = Increment(x=w943) -> (x+1=w934:i32)
                n599 = local write "All trials"(w934) -> ()
                n600 = Boolean To (0,1)(Boolean=w939) -> (0, 1=w938:i16)
                n601 = Build Array(i16 0 ("element"), w938) -> (w937:i16[])
                n602 = Decrement(x=w934) -> (x-1=w936:i32)
                n603 = Insert Into Array(array=w940, index (row)=w936, new element=w937) -> (w941:i8[][])  [unwired: 1 in]
                n604 = local write "Trial type array"(w941) -> ()
                n605 = local write "Trial counted"(TRUE ("Trial counted")) -> ()
              }
            }
          }
          frame Enabled {
          }
        }
        n606 = local read "Trial block"() -> (w884:u16)
        n607 = local read "Trial block"() -> (w890:u16)
        n608 = local read "All trials"() -> (w879:i32)
        n609 = local read "All trials"() -> (w891:i32)
        n610 = local read "Shuffle"() -> (w895:bool)
        n611 = local read "prev. diode position"() -> (w872:dbl)
        n612 = local read "Mate"() -> (w888:bool)
        n613 = case shown="False" w888 {
          tunnel: [w944 w945] -> w887
          frame True {
            n614 = local read "Prev. rew. pos."() -> (w944:dbl)
          }
          frame False {
            n615 = local read "prev. diode position"() -> (w945:dbl)
          }
        }
        n616 = local read "prev. diode position"() -> (w903:dbl)
        n617 = Subtract(x=w884, y=u16 1) -> (x-y=w883:u16)
        n618 = Greater?(x=w879, y=0) -> (0:w877:bool)
        n619 = Quotient & Remainder(x=w891, y=w890) -> (x-y*floor(x/y)=w892:i32)  [unwired: 1 out]
        n620 = local read "total distance cm"() -> (w906:sgl[])
        n621 = local read "Reward given"() -> (w902:bool)
        n622 = local read "Trial counted"() -> (w886:bool)
        n623 = Equal?(x=w892, y=w883) -> (x = y?=w881:bool)
        n624 = Equal?(x=w892, y=0.0) -> (x = y?=w894:bool)
        n625 = First Call?() -> (First Call?: T/F=w873:bool)
        n626 = local read "hit trial"() -> (w885:bool)
        n627 = Compound Arithmetic op=AND(w881, w877) -> (w880:bool)
        n628 = Compound Arithmetic op=AND(w894, w895) -> (w893:bool)
        n629 = Not(x=w873) -> (.not. x?=w870:bool)
        n630 = Greater?(x=w872, y=0.0) -> (0:w869:bool)
        n631 = case shown="True" w880 {
          frame False {
          }
          frame True {
            n632 = local write "Shuffle"(TRUE ("Shuffle")) -> ()
          }
        }
        n633 = case shown="True" w893 {
          frame False {
          }
          frame True {
            n634 = local read "shuffled array"() -> (w999:i16[])
            n635 = call "Shuffle 1D Array.vim"("array"=w999) -> ("shuffled array"=w998:i16[])  [unwired: 4 in]
            n636 = local write "shuffled array"(w998) -> ()
            n637 = local write "Shuffle"(FALSE ("Shuffle")) -> ()
          }
        }
        n638 = Not(x=w886) -> (.not. x?=w875:bool)
        n639 = Array Max & Min(array=w906) -> (max value=w907:sgl)  [unwired: 3 out]
        n640 = call "Is Value Changed.vim"("value"=w887) -> ("changed or first call?"=w874:bool)
        n641 = call "Is Value Changed.vim"("value"=w902) -> ("changed or first call?"=w900:bool)
        n642 = Subtract(x=w907, y=w903) -> (x-y=w904:dbl)
        n643 = Compound Arithmetic op=AND(w874, w875, w870, w869) -> (w876:bool)
        n644 = Less?(x=w904, y=15.0) -> (x < y?=w901:bool)
        n645 = case shown="True" w876 {
          frame False {
          }
          frame True {
            n646 = stacked-sequence {
              frame #0 {
                n647 = local read "Stim trial"() -> (w946:bool)
                n648 = local read "Reward given"() -> (w953:bool)
                n649 = local read "Stim trial"() -> (w948:bool)
                n650 = local read "Reward given"() -> (w951:bool)
                n651 = local read "Stim trial"() -> (w952:bool)
                n652 = local read "hit trial"() -> (w955:bool)
                n653 = local read "hit trial"() -> (w949:bool)
                n654 = case shown="True" w946 {
                  frame False {
                    n655 = local read "Ctrl. count"() -> (w958:i32)
                    n656 = Increment(x=w958) -> (x+1=w959:i32)
                    n657 = local write "Ctrl. count"(w959) -> ()
                  }
                  frame True {
                    n658 = local read "Stim. count"() -> (w961:i32)
                    n659 = Increment(x=w961) -> (x+1=w960:i32)
                    n660 = local write "Stim. count"(w960) -> ()
                  }
                }
                n661 = local read "All trials"() -> (w957:i32)
                n662 = Not(x=w948) -> (.not. x?=w947:bool)
                n663 = Compound Arithmetic op=AND(w953, w955, w947) -> (w954:bool)
                n664 = Compound Arithmetic op=AND(w951, w949, w952) -> (w950:bool)
                n665 = Increment(x=w957) -> (x+1=w956:i32)
                n666 = case shown="True" w954 {
                  frame False {
                  }
                  frame True {
                    n667 = local read "Hit trials ctrl."() -> (w964:i32)
                    n668 = Increment(x=w964) -> (x+1=w965:i32)
                    n669 = local write "Hit trials ctrl."(w965) -> ()
                  }
                }
                n670 = case shown="True" w950 {
                  frame False {
                  }
                  frame True {
                    n671 = local read "Hit trials stim."() -> (w962:i32)
                    n672 = Increment(x=w962) -> (x+1=w963:i32)
                    n673 = local write "Hit trials stim."(w963) -> ()
                  }
                }
                n674 = local write "All trials"(w956) -> ()
              }
              frame #1 {
                w996 = TRUE ("Trial counted")
                # "Build trial type array counting trials \nat the beginning"
                n675 = local read "shuffled array"() -> (w978:i16[])
                n676 = local read "Trial block"() -> (w992:u16)
                n677 = local read "Trial types"() -> (w979:u16[][])
                n678 = local read "All trials"() -> (w990:i32)
                n679 = local write "Trial counted"(w996) -> ()
                n680 = local write "select trial"(w996) -> ()
                n681 = Quotient & Remainder(x=w990, y=w992) -> (x-y*floor(x/y)=w977:i32)  [unwired: 1 out]
                n682 = Increment(x=w977) -> (x+1=w976:i32)
                n683 = Index Array(array=w978, index=w977) -> (element=w991:i16)
                n684 = Index Array(array=w978, index=w976) -> (element=w974:i16)
                n685 = Index Array(array=w979, index (row)=1, index (col)=w991) -> (element=w983:u16)
                n686 = Index Array(array=w979, index (row)=0, index (col)=w991) -> (element=w982:u16)
                n687 = Index Array(array=w979, index (row)=0, index (col)=w974) -> (element=w975:u16)
                n688 = Index Array(array=w979, index (row)=1, index (col)=w974) -> (element=w973:u16)
                n689 = property on="Stim protocols" class="Ring (strict)"() -> ("Strings []"=w989:string[])  [unwired: 2 in, 2 out]
                n690 = Greater?(x=w982, y=i8 0) -> (0:w984:bool)
                n691 = local write "Mask prot command"(w983) -> ()
                n692 = local write "Stim prot command"(w982) -> ()
                n693 = local read "Trial type array"() -> (w994:i8[][])
                n694 = Select(t=TRUE, s=w984, f=FALSE) -> (s? t:f=w981:bool)
                n695 = local read "All trials"() -> (w980:i32)
                n696 = Index Array(array=w989, index=w982) -> (element=w988:string)
                n697 = Index Array(array=w989, index=w975) -> (element=w987:string)
                n698 = Index Array(array=w989, index=w983) -> (element=w986:string)
                n699 = Index Array(array=w989, index=w973) -> (element=w985:string)
                n700 = local write "Stim trial"(w981) -> ()
                n701 = local write "Next mask protocol"(w985) -> ()
                n702 = local write "Current stim. protocol"(w988) -> ()
                n703 = local write "Next trial stim. protocol"(w987) -> ()
                n704 = local write "Current mask protocol"(w986) -> ()
                n705 = Build Array(w982, w983) -> (w993:u16[])
                n706 = Insert Into Array(array=w994, index (row)=w980, new element=w993) -> (w995:i8[][])  [unwired: 1 in]
                n707 = local write "Trial type array"(w995) -> ()
              }
            }
          }
        }
        n708 = Compound Arithmetic op=AND(w900, w885, w901) -> (w899:bool)
        n709 = case shown="True" w899 {
          frame False {
          }
          frame True {
            n710 = local read "Hit trials"() -> (w1008:i16)
            n711 = Increment(x=w1008) -> (x+1=w1007:i16)
            n712 = local write "Hit trials"(w1007) -> ()
          }
        }
        n713 = local read "Mate"() -> (w898:bool)
        n714 = local read "total distance cm"() -> (w909:sgl[])
        n715 = case shown="False" w898 {
          tunnel: [140.0 ("y") w1004] -> w897
          tunnel: [w1001 w1003] -> w896
          frame False {
            n716 = local read "prev. diode position"() -> (w1001:dbl)
          }
          frame True {
            n717 = local read "Prev. rew. pos."() -> (w1003:dbl)
            n718 = local read "Reward freq. (cm)"() -> (w1006:dbl)
            n719 = Subtract(x=w1006, y=15.0) -> (x-y=w1004:dbl)
          }
        }
        n720 = local read "Trial counted"() -> (w917:bool)
        n721 = Array Max & Min(array=w909) -> (max value=w908:sgl)  [unwired: 3 out]
        n722 = Subtract(x=w908, y=w896) -> (x-y=w918:dbl)
        n723 = Greater?(x=w918, y=w897) -> (0:w916:bool)
        n724 = And(x=w916, y=w917) -> (x .and. y?=w915:bool)
        n725 = case shown="True" w915 {
          frame False {
          }
          frame True {
            n726 = local write "Trial counted"(FALSE ("Trial counted")) -> ()
          }
        }
        n727 = local read "SciScan"() -> (w919:bool)
        n728 = local read "Stop recording"() -> (w922:bool)
        n729 = case shown="True" w919 {
          frame False {
          }
          frame True {
            n730 = local read "SciScan start"() -> (w1011:refnum<k21>)
            n731 = local write "2P imaging"("2P imaging: YES" ("2P imaging")) -> ()
            n732 = call-poly <vilib>:"DAQmx Write.vi"("task/channels in"=w1011, "data"=TRUE) -> ()  [unwired: 11 in, 3 out]
          }
        }
        n733 = local read "Exit program"() -> (w923:bool)
        n734 = local read "Hit trials"() -> (w914:i16)
        n735 = local read "All trials"() -> (w913:i32)
        n736 = Divide(x=w914, y=w913) -> (x/y=w911:dbl)
        "P hit trials" <- w911
        n737 = Or(x=w922, y=w923) -> (x .or. y?=w920:bool)
        n738 = Multiply(x=w911, y=100.0) -> (x*y=→"Hit trials %":dbl)
        n739 = Select(t=T12."Stop Recording" ("main program"), s=w920, f=T12."Record" ("main program")) -> (s? t:f=w921:T12)
      }
      frame "Record VR" {
        w1042 = 100.0 ("y")
        # "These computations run only once in a trial when the mouse enters to the RZ"
        # "These computations run only once in a trial at the very beginning"
        n740 = local read "Unity position:"() -> (w1021:sgl)
        n741 = local read "Trial block"() -> (w1013:u16)
        n742 = local read "Trial counted"() -> (w1027:bool)
        n743 = local read "All trials"() -> (w1020:i32)
        n744 = Equal?(x=w1027, y=FALSE) -> (x = y?=w1024:bool)
        n745 = local read "Shuffle"() -> (w1037:bool)
        n746 = Less?(x=w1021, y=0.0) -> (x < y?=w1025:bool)
        n747 = local read "Hit trials stim."() -> (w1044:i32)
        n748 = local read "Stim. count"() -> (w1045:i32)
        n749 = local read "Ctrl. count"() -> (w1047:i32)
        n750 = local read "Hit trials ctrl."() -> (w1046:i32)
        n751 = Compound Arithmetic op=AND(w1024, w1025) -> (w1026:bool)
        n752 = Quotient & Remainder(x=w1020, y=w1013) -> (x-y*floor(x/y)=w1033:i32)  [unwired: 1 out]
        n753 = Decrement(x=w1013) -> (x-1=w1014:u16)
        n754 = case shown="True" w1026 {
          frame False {
          }
          frame True {
            n755 = stacked-sequence {
              frame #0 {
                # "Build trial type array counting trials \nat the beginning"
                n756 = local read "shuffled array"() -> (w1093:i16[])
                n757 = local read "Trial block"() -> (w1114:u16)
                n758 = local read "Trial types"() -> (w1096:u16[][])
                n759 = local read "All trials"() -> (w1112:i32)
                n760 = Quotient & Remainder(x=w1112, y=w1114) -> (x-y*floor(x/y)=w1092:i32)  [unwired: 1 out]
                n761 = Increment(x=w1092) -> (x+1=w1091:i32)
                n762 = Index Array(array=w1093, index=w1092) -> (element=w1113:i16)
                n763 = Index Array(array=w1093, index=w1091) -> (element=w1089:i16)
                n764 = Index Array(array=w1096, index (row)=1, index (col)=w1113) -> (element=w1105:u16)
                n765 = Index Array(array=w1096, index (row)=0, index (col)=w1113) -> (element=w1104:u16)
                n766 = Index Array(array=w1096, index (row)=0, index (col)=w1089) -> (element=w1090:u16)
                n767 = Index Array(array=w1096, index (row)=1, index (col)=w1089) -> (element=w1088:u16)
                n768 = property on="Stim protocols" class="Ring (strict)"() -> ("Strings []"=w1111:string[])  [unwired: 2 in, 2 out]
                n769 = Greater?(x=w1104, y=i8 0) -> (0:w1106:bool)
                n770 = local write "Mask prot command"(w1105) -> ()
                n771 = local write "Stim prot command"(w1104) -> ()
                n772 = local read "Trial type array"() -> (w1116:i8[][])
                n773 = Select(t=TRUE, s=w1106, f=FALSE) -> (s? t:f=w1103:bool)
                n774 = local read "All trials"() -> (w1102:i32)
                n775 = Index Array(array=w1111, index=w1104) -> (element=w1110:string)
                n776 = Index Array(array=w1111, index=w1090) -> (element=w1109:string)
                n777 = Index Array(array=w1111, index=w1105) -> (element=w1108:string)
                n778 = Index Array(array=w1111, index=w1088) -> (element=w1107:string)
                n779 = local write "Stim trial"(w1103) -> ()
                n780 = local write "Next mask protocol"(w1107) -> ()
                n781 = local write "Current stim. protocol"(w1110) -> ()
                n782 = local write "Next trial stim. protocol"(w1109) -> ()
                n783 = local write "Current mask protocol"(w1108) -> ()
                n784 = Build Array(w1104, w1105) -> (w1115:u16[])
                n785 = Insert Into Array(array=w1116, index (row)=w1102, new element=w1115) -> (w1117:i8[][])  [unwired: 1 in]
                n786 = local write "Trial type array"(w1117) -> ()
              }
              frame #1 {
                w1118 = TRUE ("Trial counted")
                n787 = local write "Trial counted"(w1118) -> ()
                n788 = local write "select trial"(w1118) -> ()
                n789 = local read "Stim trial"() -> (w1119:bool)
                n790 = local read "Reward given"() -> (w1126:bool)
                n791 = local read "Stim trial"() -> (w1121:bool)
                n792 = local read "Reward given"() -> (w1124:bool)
                n793 = local read "Stim trial"() -> (w1125:bool)
                n794 = local read "hit trial"() -> (w1128:bool)
                n795 = local read "hit trial"() -> (w1122:bool)
                n796 = case shown="True" w1119 {
                  frame False {
                    n797 = local read "Ctrl. count"() -> (w1131:i32)
                    n798 = Increment(x=w1131) -> (x+1=w1132:i32)
                    n799 = local write "Ctrl. count"(w1132) -> ()
                  }
                  frame True {
                    n800 = local read "Stim. count"() -> (w1134:i32)
                    n801 = Increment(x=w1134) -> (x+1=w1133:i32)
                    n802 = local write "Stim. count"(w1133) -> ()
                  }
                }
                n803 = local read "All trials"() -> (w1130:i32)
                n804 = Not(x=w1121) -> (.not. x?=w1120:bool)
                n805 = Compound Arithmetic op=AND(w1126, w1128, w1120) -> (w1127:bool)
                n806 = Compound Arithmetic op=AND(w1124, w1122, w1125) -> (w1123:bool)
                n807 = Increment(x=w1130) -> (x+1=w1129:i32)
                n808 = case shown="True" w1127 {
                  frame False {
                  }
                  frame True {
                    n809 = local read "Hit trials ctrl."() -> (w1137:i32)
                    n810 = Increment(x=w1137) -> (x+1=w1138:i32)
                    n811 = local write "Hit trials ctrl."(w1138) -> ()
                  }
                }
                n812 = case shown="True" w1123 {
                  frame False {
                  }
                  frame True {
                    n813 = local read "Hit trials stim."() -> (w1135:i32)
                    n814 = Increment(x=w1135) -> (x+1=w1136:i32)
                    n815 = local write "Hit trials stim."(w1136) -> ()
                  }
                }
                n816 = local write "All trials"(w1129) -> ()
              }
            }
          }
        }
        n817 = Equal?(x=w1033, y=w1014) -> (x = y?=w1034:bool)
        n818 = Equal?(x=w1033, y=0.0) -> (x = y?=w1036:bool)
        n819 = Compound Arithmetic op=AND(w1036, w1037) -> (w1035:bool)
        n820 = Divide(x=w1044, y=w1045) -> (x/y=w1040:dbl)
        "P stim. Hit" <- w1040
        n821 = Divide(x=w1046, y=w1047) -> (x/y=w1041:dbl)
        "P ctrl. Hit" <- w1041
        n822 = case shown="True" w1034 {
          frame False {
          }
          frame True {
            n823 = local write "Shuffle"(TRUE ("Shuffle")) -> ()
          }
        }
        n824 = case shown="True" w1035 {
          frame False {
          }
          frame True {
            n825 = local read "shuffled array"() -> (w1144:i16[])
            n826 = call "Shuffle 1D Array.vim"("array"=w1144) -> ("shuffled array"=w1143:i16[])  [unwired: 4 in]
            n827 = local write "shuffled array"(w1143) -> ()
            n828 = local write "Shuffle"(FALSE ("Shuffle")) -> ()
          }
        }
        n829 = Multiply(x=w1041, y=w1042) -> (x*y=→"Control hit trials %":dbl)
        n830 = Multiply(x=w1042, y=w1040) -> (x*y=→"Stim. hit trials %":dbl)
        n831 = local read "reward zone start"() -> (w1015:dbl)
        n832 = local read "Unity position:"() -> (w1016:sgl)
        n833 = local read "select trial"() -> (w1017:bool)
        n834 = Greater?(x=w1016, y=w1015) -> (0:w1018:bool)
        n835 = Compound Arithmetic op=AND(w1018, w1017) -> (w1019:bool)
        n836 = case shown="True" w1019 {
          frame True {
            w1052 = FALSE ("Randomize")
            n837 = disable-structure shown="Disabled" {
              frame Disabled {
                n838 = local read "shuffled array"() -> (w1066:i16[])
                n839 = local read "Trial block"() -> (w1060:u16)
                n840 = local read "Trial types"() -> (w1062:u16[][])
                n841 = local read "All trials"() -> (w1067:i32)
                n842 = Quotient & Remainder(x=w1067, y=w1060) -> (x-y*floor(x/y)=w1065:i32)  [unwired: 1 out]
                n843 = Index Array(array=w1066, index=w1065) -> (element=w1061:i16)
                n844 = Index Array(array=w1062, index (row)=1, index (col)=w1061) -> (element=w1059:u16)
                n845 = Index Array(array=w1062, index (row)=0, index (col)=w1061) -> (element=w1057:u16)
                n846 = Greater?(x=w1057, y=u16 0) -> (0:w1058:bool)
                n847 = local write "Mask prot command"(w1059) -> ()
                n848 = local write "Stim prot command"(w1057) -> ()
                n849 = Select(t=TRUE ("Beaconed"), s=w1058, f=FALSE) -> (s? t:f=w1053:bool)
                n850 = local write "Stim trial"(w1053) -> ()
              }
              frame Enabled {
              }
            }
            n851 = local write "Trial counted"(w1052) -> ()
            n852 = local write "select trial"(w1052) -> ()
            n853 = local read "VR start pos"() -> (w1050:T1)
            n854 = case shown="\"Non-random\"" w1050 {
              tunnel: [w1069 "0," w1080] -> w1051
              frame "Random of 4", Default {
                n855 = local write "Random start pos"(TRUE ("Random start pos")) -> ()
                n856 = Build Array("0,", "2,", "4,", "6,") -> (w1075:string[])
                n857 = call "Shuffle 1D Array.vim"("array"=w1075) -> ("shuffled array"=w1076:string[])  [unwired: 4 in]
                n858 = Index Array(array=w1076, index=0) -> (element=w1069:string)
              }
              frame "Non-random" {
                n859 = local write "Random start pos"(TRUE ("Random start pos")) -> ()
              }
              frame "Random of 2" {
                n860 = local write "Random start pos"(TRUE ("Random start pos")) -> ()
                n861 = Build Array("0,", "6,", "0,", "6,") -> (w1083:string[])
                n862 = call "Shuffle 1D Array.vim"("array"=w1083) -> ("shuffled array"=w1081:string[])  [unwired: 4 in]
                n863 = Index Array(array=w1081, index=0) -> (element=w1080:string)
              }
            }
            n864 = local write "offset tag"(w1051) -> ()
          }
          frame False {
          }
        }
        n865 = local read "SciScan"() -> (w1028:bool)
        n866 = case shown="True" w1028 {
          frame False {
          }
          frame True {
            n867 = local read "SciScan start"() -> (w1140:refnum<k21>)
            n868 = local write "2P imaging"("2P imaging: YES" ("2P imaging")) -> ()
            n869 = call-poly <vilib>:"DAQmx Write.vi"("task/channels in"=w1140, "data"=TRUE) -> ()  [unwired: 11 in, 3 out]
          }
        }
        n870 = local read "Stop recording"() -> (w1029:bool)
        n871 = local read "Exit program"() -> (w1030:bool)
        n872 = disable-structure shown="Disabled" {
          frame Disabled {
            n873 = local write "Gain"("NBC Gain") -> ()
          }
          frame Enabled {
          }
        }
        n874 = Or(x=w1029, y=w1030) -> (x .or. y?=w1048:bool)
        n875 = Select(t=T12."Stop Recording" ("main program"), s=w1048, f=T12."Record VR" ("main program")) -> (s? t:f=w1049:T12)
      }
    }
    n876 = Wait (ms)(milliseconds to wait=u32 3) -> ()  [unwired: 1 out]
    n877 = local read "Exit"() -> (w296:bool)
  }
  n878 = property on="select trial" class="Bool (strict)"("Visible"=FALSE) -> ()  [unwired: 2 in, 2 out]
  n879 = while {
    shift-right: [w1174] -> _
    shift-left: w121 -> [w1173]
    shift-right: [w1170] -> _
    shift-left: _ -> [w1167]
    shift-right: [w1161] -> _
    shift-left: _ -> [w1166]
    shift-right: [w1169] -> _
    shift-left: _ -> [w1163]
    shift-right: [w1168] -> _
    shift-left: _ -> [w1162]
    shift-right: [w1165] -> _
    shift-left: _ -> [w1164]
    shift-right: [w1160] -> _
    shift-left: _ -> [w1159]
    shift-right: [w1156] -> _
    shift-left: _ -> [w1158]
    shift-right: [w1155] -> _
    shift-left: _ -> [w1157]
    shift-right: [w1154] -> _
    shift-left: 0.0 -> [w1153]
    shift-right: [w1152] -> _
    shift-left: _ -> [w1150]
    shift-right: [w1151] -> _
    shift-left: _ -> [w1149]
    shift-right: [w1148] -> _
    shift-left: _ -> [w1147]
    stop <- w1171 stop-if-true
    n880 = case shown="\"Record VR\"" w1173 {
      selector: w1173 -> [w1266 _ w1352 w1383 w1628 w1701]
      tunnel: [w1262 w1312 w1353 Record_enum."Idle" ("Record enum") w1629 w1702] -> w1174
      tunnel: [FALSE ("Exit") FALSE ("Exit") w1351 FALSE ("Exit") FALSE ("Exit") FALSE ("Exit")] -> w1171
      tunnel: [w1210 w1321 w1350 refnum<k21> refnum ("task out") w1610 w1698] -> w1170
      tunnel: [w1208 w1320 w1349 w1372 w1609 w1697] -> w1161
      tunnel: [w1204 w1319 w1346 refnum<k21> refnum ("task out") w1603 w1694] -> w1169
      tunnel: [w1206 w1318 w1345 w1371 w1602 w1693] -> w1168
      tunnel: w1167 -> [w1211 _ w1350 w1375 w1617 w1698]
      tunnel: w1166 -> [w1209 _ w1349 w1376 w1616 w1697]
      tunnel: [w1260 dbl[] [] w1348 w1381 w1542 w1696] -> w1165
      tunnel: w1164 -> [w1260 _ w1348 w1381 w1553 w1696]
      tunnel: w1163 -> [w1205 _ w1346 w1378 w1612 w1694]
      tunnel: w1162 -> [w1207 _ w1345 w1377 w1611 w1693]
      tunnel: [w1259 w1317 w1347 w1380 w1563 w1695] -> w1160
      tunnel: w1159 -> [w1259 _ w1347 w1380 w1599 w1695]
      tunnel: w1158 -> [_ _ _ _ w1588 _]
      tunnel: w1157 -> [_ _ _ _ w1584 _]
      tunnel: [0.0 0.0 0.0 0.0 w1590 0.0] -> w1156
      tunnel: [0.0 0.0 0.0 0.0 w1589 0.0] -> w1155
      tunnel: [w1256 w1307 w1341 w1367 w1567 w1690] -> w1154
      tunnel: w1153 -> [w1256 w1307 w1341 w1367 _ w1690]
      tunnel: [w1202 w1297 w1337 refnum<k21> refnum ("task out") w1559 w1689] -> w1152
      tunnel: [w1200 w1296 w1336 w1362 w1564 w1688] -> w1151
      tunnel: w1150 -> [w1203 _ w1337 w1365 w1562 w1689]
      tunnel: w1149 -> [w1201 _ w1336 w1364 w1565 w1688]
      tunnel: [w1229 dbl[] [] ("data") w1335 w1357 w1517 w1687] -> w1148
      tunnel: w1147 -> [w1229 _ w1335 w1357 _ w1687]
      frame "Init recording" {
        w1186 = " Hz" ("string")
        w1189 = "\n" ("string")
        w1222 = "-" ("string")
        # "Create a \"header\" for the lab book file from those variables that do not change during the recording"
        n881 = local write "Record loop state"(w1266) -> ()
        n882 = local read "Weight"() -> (w1244:dbl)
        n883 = local read "%"() -> (w1242:dbl)
        n884 = local read "Original weight"() -> (w1246:dbl)
        n885 = Number To Fractional String(number=w1242, precision (6)=i16 2) -> (F-format string=w1243:string)  [unwired: 2 in]
        n886 = Number To Fractional String(number=w1244, precision (6)=i16 1) -> (F-format string=w1245:string)  [unwired: 2 in]
        n887 = local read "VR Mode"() -> (w1228:bool)
        n888 = local read "Last calibration"() -> (w1249:string)
        n889 = Number To Fractional String(number=w1246, precision (6)=i16 1) -> (F-format string=w1247:string)  [unwired: 2 in]
        n890 = Concatenate Strings("Weight: " ("string"), w1243, " %   ( " ("string"), w1245, " g ; weight before water restriction: " ("string"), w1247, " g)" ("string")) -> (w1234:string)
        n891 = local read "Sample rate"() -> (w1195:dbl)
        n892 = case shown="True" w1228 {
          tunnel: ["" w1275] -> w1223
          frame False {
          }
          frame True {
            n893 = local read "reward zone start"() -> (w1271:dbl)
            n894 = Number To Decimal String(number=w1271) -> (decimal integer string=w1274:string)  [unwired: 1 in]
            n895 = Concatenate Strings("-" ("string"), w1274, "cm" ("string")) -> (w1275:string)
          }
        }
        n896 = local read "Loop rate"() -> (w1194:dbl)
        n897 = Concatenate Strings("Last calibration of water valve: " ("string"), w1249) -> (w1230:string)
        n898 = Number To Decimal String(number=w1195) -> (decimal integer string=w1192:string)  [unwired: 1 in]
        n899 = Number To Decimal String(number=w1194) -> (decimal integer string=w1188:string)  [unwired: 1 in]
        n900 = local read "Software version"() -> (w1231:string)
        n901 = local read "Mouse name"() -> (w1232:string)
        n902 = call <vilib>:"DAQmx Stop Task.vi"("task/channels in"=w1211, "error in"=w1209) -> ("task out"=w1217:refnum<k21>, "error out"=w1216:errorcluster)  [unwired: 12 in]
        n903 = Concatenate Strings("Sampling rate: " ("string"), w1192, w1186, " Loop rate: " ("string"), w1188, w1186) -> (w1191:string)
        n904 = Format Date/Time String(time format string (%c)="%Y%m%d") -> (date/time string=w1184:string)  [unwired: 2 in]
        n905 = Format Date/Time String(time format string (%c)="%Y.%m.%d %H:%M:%S") -> (date/time string=w1198:string)  [unwired: 2 in]
        n906 = call <vilib>:"DAQmx Start Task.vi"("task/channels in"=w1217, "error in"=w1216) -> ("task out"=w1210:refnum<k21>, "error out"=w1208:errorcluster)  [unwired: 12 in]
        n907 = Concatenate Strings(w1198, "   " ("string"), w1232, w1189, w1189, w1234, w1189, w1230, w1189, w1231, w1189, w1191, w1189, "\n******************************" ("string"), w1189, w1189) -> (w1251:string)
        n908 = local read "Mouse name"() -> (w1227:string)
        n909 = local read "Recording folder"() -> (w1180:path)
        n910 = local read "Unique ID"() -> (w1218:i8)
        n911 = call <vilib>:"DAQmx Stop Task.vi"("task/channels in"=w1205, "error in"=w1207) -> ("task out"=w1214:refnum<k21>, "error out"=w1215:errorcluster)  [unwired: 12 in]
        n912 = local write "Header"(w1251) -> ()
        n913 = local write "Lab book notes"(w1251) -> ()
        n914 = Format Date/Time String(time format string (%c)="%Y.%m.%d") -> (date/time string=w1176:string)  [unwired: 2 in]
        n915 = Format Into String(format string="%02d", w1218) -> (resulting string=w1219:string)  [unwired: 2 in, 1 out]
        n916 = call <vilib>:"DAQmx Start Task.vi"("task/channels in"=w1214, "error in"=w1215) -> ("task out"=w1204:refnum<k21>, "error out"=w1206:errorcluster)  [unwired: 12 in]
        n917 = local read "Comment"() -> (w1221:string)
        n918 = Match Pattern(string=w1227, regular expression="-") -> (before substring=w1225:string, after substring=w1224:string)  [unwired: 1 in, 2 out]
        n919 = Strip Path(path=w1180) -> (stripped path=w1179:path)  [unwired: 1 out]
        n920 = Build Path(base path=w1179, name or relative path="PupilData") -> (appended path=w1177:path)
        n921 = call <vilib>:"DAQmx Stop Task.vi"("task/channels in"=w1203, "error in"=w1201) -> ("task out"=w1213:refnum<k21>, "error out"=w1212:errorcluster)  [unwired: 12 in]
        n922 = Build Path(base path=w1180, name or relative path=w1176) -> (appended path=w1269:path)
        n923 = Build Path(base path=w1177, name or relative path=w1176) -> (appended path=w1175:path)
        n924 = Concatenate Strings(w1225, w1222, w1184, w1222, w1219, w1222, w1224, w1223, w1222, w1221) -> (w1182:string)
        n925 = call <vilib>:"DAQmx Start Task.vi"("task/channels in"=w1213, "error in"=w1212) -> ("task out"=w1202:refnum<k21>, "error out"=w1200:errorcluster)  [unwired: 12 in]
        n926 = call <vilib>:"Check if File or Folder Exists.vi"("path"=w1269) -> ("file or folder exists?"=w1268:bool, "dup path"=w1267:path)  [unwired: 8 in, 1 out]
        n927 = Format Date/Time String(time format string (%c)="Session start: %H:%M:%S\n") -> (date/time string=→"Session start:":string)  [unwired: 2 in]
        n928 = case shown="False" w1268 {
          tunnel: [w1284 w1286] -> w1181
          tunnel: w1267 -> [w1284 w1285]
          frame True {
          }
          frame False {
            n929 = Create Folder(path (use dialog)=w1285) -> (created path=w1286:path)  [unwired: 2 in, 2 out]
          }
        }
        n930 = local write "Pupil Exp day folder"(w1175) -> ()
        n931 = Concatenate Strings(w1182, ".tdms") -> (w1250:string)
        n932 = Concatenate Strings(w1182, ".txt" ("string")) -> (w1254:string)
        n933 = Build Path(base path=w1181, name or relative path=w1254) -> (appended path=w1252:path)
        n934 = Build Path(base path=w1181, name or relative path=w1250) -> (appended path=w1265:path)
        n935 = local write "Filename"(w1182) -> ()
        n936 = local write "Lab book file"(w1252) -> ()
        n937 = call <vilib>:"Check if File or Folder Exists.vi"("path"=w1265) -> ("file or folder exists?"=w1263:bool, "dup path"=w1264:path)  [unwired: 8 in, 1 out]
        n938 = Format Date/Time String() -> ()  [unwired: 3 in, 1 out]
        n939 = case shown="False" w1263 {
          tunnel: w1264 -> [w1280 _]
          tunnel: [Record_enum."Record VR" ("Record enum") Record_enum."Init recording" ("Record enum")] -> w1262
          frame False {
            n940 = TDMS Open(5:FALSE ("create index file? (T)"), 10:T16."create" ("operation (0:open)"), 11:w1280) -> (3:w1277:refnum<k34>)  [unwired: 4 in, 1 out]
            n941 = local write "My tdms file"(w1277) -> ()
          }
          frame True {
            n942 = local read "Unique ID"() -> (w1283:i8)
            n943 = Increment(x=w1283) -> (x+1=w1282:i8)
            n944 = local write "Unique ID"(w1282) -> ()
          }
        }
      }
      frame "Init data acquisition" {
        w1287 = 0 items=["one channel for each line", "one channel for all lines"] ("line grouping")
        w1293 = 10083 items=["Default"=-1, "RSE"=10083, "NRSE"=10078, "Differential"=10106, "Pseudodifferential"=12529] ("input terminal configuration")
        (unwired) tag "Dev1/ai2" ("physical channels")
        w1301 = 10123 items=["Finite Samples"=10178, "Continuous Samples"=10123, "Hardware Timed Single Point"=12522] ("sample mode")
        w1323 = 10123 items=["Finite Samples"=10178, "Continuous Samples"=10123, "Hardware Timed Single Point"=12522] ("sample mode")
        w1329 = 10123 items=["Finite Samples"=10178, "Continuous Samples"=10123, "Hardware Timed Single Point"=12522] ("sample mode")
        (unwired) tag "Dev1/port0/line3" ("lines")
        # "Valve open"
        # "Frame signal"
        # "Encoder"
        # "Lickport"
        n945 = call "Encoder read task.vi"() -> ("error out"=w1328:errorcluster, "task out"=w1327:refnum<k21>)  [unwired: 10 in]
        n946 = local read "Sample rate"() -> (w1324:dbl)
        n947 = call <vilib>:"DAQmx Flatten Channel String.vi"("names in"=string[] ["Dev1/port0/line4", "Dev1/port0/line5", "Dev1/port0/line6", "Dev1/port0/line3"]) -> ("names out"=w1289:string)  [unwired: 13 in, 1 out]
        n948 = call <vilib>:"DAQmx Flatten Channel String.vi"("names in"=string[] ["Dev1/ai0", "Dev1/ai4", "Dev1/ai6", "Dev1/ai1", "Dev1/ai2"]) -> ("names out"=w1299:string)  [unwired: 13 in, 1 out]
        n949 = local read "Sample rate"() -> (w1331:dbl)
        n950 = local read "Sample rate"() -> (w1303:dbl)
        n951 = call-poly <vilib>:"DAQmx Create Virtual Channel.vi"("lines"=w1289, "line grouping"=w1287) -> ("task out"=w1330:refnum<k21>, "error out"=w1332:errorcluster)  [unwired: 12 in]
        n952 = call-poly <vilib>:"DAQmx Create Virtual Channel.vi"("maximum value"=10.0, "minimum value"=-10.0, "input terminal configuration"=w1293, "physical channels"=w1299) -> ("task out"=w1302:refnum<k21>, "error out"=w1304:errorcluster)  [unwired: 10 in]
        n953 = call-poly <vilib>:"DAQmx Timing.vi"("task/channels in"=w1327, "sample mode"=w1323, "rate"=w1324, "source"=tag "/Dev1/di/SampleClock", "error in"=w1328) -> ("task out"=w1325:refnum<k21>, "error out"=w1326:errorcluster)  [unwired: 9 in]
        n954 = call-poly <vilib>:"DAQmx Timing.vi"("task/channels in"=w1330, "sample mode"=w1329, "rate"=w1331, "source"=tag "OnboardClock", "error in"=w1332) -> ("task out"=w1333:refnum<k21>, "error out"=w1334:errorcluster)  [unwired: 9 in]
        n955 = call-poly <vilib>:"DAQmx Timing.vi"("task/channels in"=w1302, "sample mode"=w1301, "rate"=w1303, "source"=tag "/Dev1/di/SampleClock", "error in"=w1304) -> ("task out"=w1305:refnum<k21>, "error out"=w1306:errorcluster)  [unwired: 9 in]
        n956 = call <vilib>:"DAQmx Start Task.vi"("task/channels in"=w1325, "error in"=w1326) -> ("task out"=w1321:refnum<k21>, "error out"=w1320:errorcluster)  [unwired: 12 in]
        n957 = call <vilib>:"DAQmx Start Task.vi"("task/channels in"=w1333, "error in"=w1334) -> ("task out"=w1319:refnum<k21>, "error out"=w1318:errorcluster)  [unwired: 12 in]
        n958 = call <vilib>:"DAQmx Start Task.vi"("task/channels in"=w1305, "error in"=w1306) -> ("task out"=w1297:refnum<k21>, "error out"=w1296:errorcluster)  [unwired: 12 in]
        n959 = local write "prev. diode position"(-157.0 ("prev. diode position")) -> ()
        n960 = local write "Store prev encoder count"(w1307) -> ()
        n961 = local read "Record"() -> (w1315:bool)
        n962 = Tick Count (ms)() -> (millisecond timer value=w1317:u32)
        "Start time" <- w1317
        n963 = local write "index"(0 ("index")) -> ()
        n964 = Select(t=Record_enum."Init recording" ("Record enum"), s=w1315, f=Record_enum."Record VR" ("Record enum")) -> (s? t:f=w1312:T5)
      }
      frame "Idle" {
        n965 = local write "Record loop state"(w1352) -> ()
        n966 = Multiply(x=50.0, y=3.141592653589793) -> (x*y=→"Wheel circumference":dbl)
        n967 = Wait (ms)(milliseconds to wait=u32 20) -> ()  [unwired: 1 out]
        n968 = local read "Run experiment"() -> (w1356:bool)
        n969 = Select(t=Record_enum."Init data acquisition" ("Record enum"), s=w1356, f=Record_enum."Idle" ("Record enum")) -> (s? t:f=w1353:T5)
        n970 = local read "Exit"() -> (w1351:bool)
      }
      frame "Stop data acquision" {
        n971 = local write "Record loop state"(w1383) -> ()
        n972 = local read "Record"() -> (w1370:bool)
        n973 = call <vilib>:"DAQmx Stop Task.vi"("task/channels in"=w1378, "error in"=w1377) -> ("task out"=w1373:refnum<k21>, "error out"=w1379:errorcluster)  [unwired: 12 in]
        n974 = call <vilib>:"DAQmx Stop Task.vi"("task/channels in"=w1365, "error in"=w1364) -> ("task out"=w1363:refnum<k21>, "error out"=w1366:errorcluster)  [unwired: 12 in]
        n975 = call <vilib>:"DAQmx Stop Task.vi"("task/channels in"=w1375, "error in"=w1376) -> ("task out"=w1374:refnum<k21>, "error out"=w1361:errorcluster)  [unwired: 12 in]
        n976 = call <vilib>:"DAQmx Clear Task.vi"("task in"=w1373, "error in"=w1379) -> ("error out"=w1371:errorcluster)  [unwired: 13 in]
        n977 = call <vilib>:"DAQmx Clear Task.vi"("task in"=w1363, "error in"=w1366) -> ("error out"=w1362:errorcluster)  [unwired: 13 in]
        n978 = call <vilib>:"DAQmx Clear Task.vi"("task in"=w1374, "error in"=w1361) -> ("error out"=w1372:errorcluster)  [unwired: 13 in]
        n979 = case shown="True" w1370 {
          frame False {
            n980 = local write "Start recording"(FALSE ("Start recording")) -> ()
          }
          frame True {
            w1387 = "\n"
            # "Write labbook data"
            n981 = local read "My tdms file"() -> (w1429:refnum<k34>)
            n982 = local read "VR Mode"() -> (w1397:bool)
            n983 = local write "Record Button"(FALSE ("Record Button")) -> ()
            n984 = local read "Security camera"() -> (w1389:string)
            n985 = local write "Record"(FALSE ("Logg data")) -> ()
            n986 = local read "2P imaging"() -> (w1388:string)
            n987 = case shown="True" w1397 {
              tunnel: [w1458 w1500] -> w1395
              frame True {
                w1433 = "\n" ("string")
                w1447 = "\n" ("string")
                w1461 = " (" ("string")
                # "VR Variables"
                n988 = local read "Trial types"() -> (w1436:u16[][])
                n989 = local read "Trial type array"() -> (w1446:i8[][])
                n990 = Add Array Elements(numeric array=w1436) -> (sum=w1438:u16)
                n991 = Greater?(x=w1438, y=i16 0) -> (0:w1435:bool)
                n992 = Number To Decimal String(number=w1446) -> (decimal integer string=w1445:string[][])  [unwired: 1 in]
                n993 = case shown="True" w1435 {
                  tunnel: ["" ("Laser stimulus calibration") w1474] -> w1432
                  frame False {
                  }
                  frame True {
                    n994 = local read "Laser stimulus calibration"() -> (w1475:string)
                    n995 = Concatenate Strings("\n" ("string"), w1475) -> (w1474:string)
                  }
                }
                n996 = local read "Stimulus protocol"() -> (w1434:string)
                n997 = Index Array(array=w1445, index (col)=0 ("disabled index (col)")) -> (element=w1444:string[])  [unwired: 1 in]
                n998 = Index Array(array=w1445, index (col)=1 ("disabled index (col)")) -> (element=w1443:string[])  [unwired: 1 in]
                n999 = local read "Masking light prot"() -> (w1456:string)
                n1000 = Concatenate Strings("Trial types (stimulus protocols):\n", w1444, "\nTrial types (masking protocols):\n", w1443) -> (w1431:string)
                n1001 = Concatenate Strings(w1434, w1433, w1431, w1433) -> (w1430:string)
                n1002 = Concatenate Strings(w1447, w1456, w1447, w1430, w1432) -> (w1455:string)
                n1003 = local read "Control hit trials %"() -> (w1449:dbl)
                n1004 = local read "Stim. hit trials %"() -> (w1448:dbl)
                n1005 = local read "Ctrl. count"() -> (w1467:i32)
                n1006 = local read "Stim. count"() -> (w1450:i32)
                n1007 = local read "All trials"() -> (w1470:i32)
                n1008 = local read "reward zone start"() -> (w1457:dbl)
                n1009 = Number To Decimal String(number=w1467) -> (decimal integer string=w1466:string)  [unwired: 1 in]
                n1010 = Number To Decimal String(number=w1470) -> (decimal integer string=w1469:string)  [unwired: 1 in]
                n1011 = Number To Fractional String(number=w1448, precision (6)=i16 2) -> (F-format string=w1460:string)  [unwired: 2 in]
                n1012 = Number To Decimal String(number=w1450) -> (decimal integer string=w1462:string)  [unwired: 1 in]
                n1013 = Number To Fractional String(number=w1449, precision (6)=i16 2) -> (F-format string=w1464:string)  [unwired: 2 in]
                n1014 = Number To Decimal String(number=w1457) -> (decimal integer string=w1453:string)  [unwired: 1 in]
                n1015 = Concatenate Strings("\nReward zone distance: " ("string"), w1453, " cm " ("string"), "\nAll trials: " ("string"), w1469, "\nControl trials: " ("string"), w1466, w1461, w1464, " % hit)\nStimulated trials: " ("string"), w1462, w1461, w1460, " % hit)\n" ("string"), w1455) -> (w1458:string)
              }
              frame False {
                w1476 = "\n" ("string")
                n1016 = local read "Trial types"() -> (w1480:u16[][])
                n1017 = Add Array Elements(numeric array=w1480) -> (sum=w1483:u16)
                n1018 = Greater?(x=w1483, y=i16 0) -> (0:w1482:bool)
                n1019 = case shown="True" w1482 {
                  tunnel: ["" ("Laser stimulus calibration") w1503] -> w1477
                  frame False {
                  }
                  frame True {
                    w1502 = "\n" ("string")
                    n1020 = local read "Stimulus protocol"() -> (w1505:string)
                    n1021 = local read "Laser stimulus calibration"() -> (w1504:string)
                    n1022 = Concatenate Strings(w1505, w1502, w1504, w1502) -> (w1503:string)
                  }
                }
                n1023 = local read "Reward zone"() -> (w1484:bool)
                n1024 = local read "Masking light prot"() -> (w1481:string)
                n1025 = case shown="True" w1484 {
                  tunnel: [w1507 w1510] -> w1485
                  frame True {
                    n1026 = local read "Mate"() -> (w1506:bool)
                    n1027 = case shown="False" w1506 {
                      tunnel: ["Reward zone starts at photo diode (0-6 cm)." ""] -> w1507
                      frame False {
                      }
                      frame True {
                      }
                    }
                  }
                  frame False {
                    n1028 = local read "Reward freq. (cm)"() -> (w1513:dbl)
                    n1029 = Number To Fractional String(number=w1513, precision (6)=i16 0) -> (F-format string=w1511:string)  [unwired: 2 in]
                    n1030 = Concatenate Strings("\nReward frequency (minimum): " ("string"), w1511) -> (w1510:string)
                  }
                }
                n1031 = Concatenate Strings(w1476, w1481, w1476, w1477) -> (w1478:string)
                n1032 = local read "Hit trials"() -> (w1495:i16)
                n1033 = local read "All trials"() -> (w1494:i32)
                n1034 = Divide(x=w1495, y=w1494) -> (x/y=w1493:dbl)
                n1035 = Number To Decimal String(number=w1494) -> (decimal integer string=w1498:string)  [unwired: 1 in]
                n1036 = Multiply(x=w1493, y=100.0) -> (x*y=w1490:dbl)
                n1037 = Number To Decimal String(number=w1495) -> (decimal integer string=w1496:string)  [unwired: 1 in]
                n1038 = Number To Fractional String(number=w1490, precision (6)=i16 2) -> (F-format string=w1488:string)  [unwired: 2 in]
                n1039 = Concatenate Strings(w1485, "\nAll trials: " ("string"), w1498, "\nHit trials: " ("string"), w1496, " (" ("string"), w1488, " % correct)" ("string")) -> (w1486:string)
                n1040 = Concatenate Strings(w1486, w1478) -> (w1500:string)
              }
            }
            n1041 = local read "Reward size (ul)"() -> (w1417:dbl)
            n1042 = TDMS Close(11:w1429) -> ()  [unwired: 1 in, 2 out]
            n1043 = local read "Water count"() -> (w1416:i32)
            n1044 = Concatenate Strings(w1387, w1389, w1387, w1388, w1387) -> (w1386:string)
            n1045 = Multiply(x=w1417, y=w1416) -> (x*y=w1415:dbl)
            n1046 = Number To Fractional String(number=w1415, precision (6)=i16 2) -> (F-format string=w1412:string)  [unwired: 2 in]
            n1047 = Concatenate Strings("\nWater received: " ("string"), w1412, " ul" ("string")) -> (w1396:string)
            n1048 = Format Date/Time String(time format string (%c)="Session stop: %H:%M:%S\n") -> (date/time string=w1391:string)  [unwired: 2 in]
            n1049 = local read "Distance (m)"() -> (w1403:dbl)
            n1050 = local read "Session start:"() -> (w1392:string)
            n1051 = local read "Time (min)"() -> (w1407:dbl)
            n1052 = Number To Fractional String(number=w1407, precision (6)=i16 2) -> (F-format string=w1408:string)  [unwired: 2 in]
            n1053 = local read "Laps"() -> (w1399:i32)
            n1054 = Number To Fractional String(number=w1403, precision (6)=i16 2) -> (F-format string=w1402:string)  [unwired: 2 in]
            n1055 = Number To Decimal String(number=w1399) -> (decimal integer string=w1398:string)  [unwired: 1 in]
            n1056 = Concatenate Strings(w1392, w1391, "Time: " ("string"), w1408, " minutes\n" ("string"), "Distance: " ("string"), w1402, " m\n" ("string"), "Laps completed: " ("string"), w1398, w1396, w1395, w1386, "******************************\n" ("string")) -> (w1394:string)
            n1057 = local read "Lab book notes"() -> (w1424:string)
            n1058 = local read "Lab book file"() -> (w1422:path)
            n1059 = local read "Header"() -> (w1425:string)
            n1060 = Match Pattern(string=w1424, regular expression="***\n") -> (after substring=w1426:string)  [unwired: 1 in, 3 out]
            n1061 = Open/Create/Replace File(file path (use dialog)=w1422, operation (0:open)=T11."create") -> (refnum out=w1423:refnum<file>)  [unwired: 4 in, 2 out]
            n1062 = Concatenate Strings(w1425, w1394, w1426) -> (w1427:string)
            n1063 = Write to Text File(file (use dialog)=w1423, text=w1427) -> (refnum out=w1421:refnum<file>)  [unwired: 2 in, 2 out]
            n1064 = Close File(refnum=w1421) -> ()  [unwired: 1 in, 2 out]
          }
        }
      }
      frame "Record VR" {
        # "Calculate Velocity (cm/s) with 50Hz sampling"
        n1065 = local read "VR Mode"() -> (w1536:bool)
        n1066 = local read "Record"() -> (w1601:bool)
        n1067 = case shown="True" w1601 {
          frame False {
          }
          frame True {
            n1068 = local read "VR Mode"() -> (w1644:bool)
            n1069 = case shown="True" w1644 {
              frame True {
                # "Mate"
                n1070 = local read "Photodiode signal"() -> (w1661:sgl[])
                n1071 = local read "total distance cm"() -> (w1659:sgl[])
                n1072 = local read "Photo stimulus signal"() -> (w1658:sgl[])
                n1073 = local read "Unity position:"() -> (w1662:sgl)
                n1074 = local read "Valve signal"() -> (w1654:i8[])
                n1075 = local read "lick signal"() -> (w1653:i8[])
                n1076 = local read "Frame signal"() -> (w1652:i8[])
                n1077 = local read "Trial type array"() -> (w1664:i8[][])
                n1078 = local read "All trials"() -> (w1665:i32)
                n1079 = local read "No. of smpl. per ch."() -> (w1660:i32)
                n1080 = local read "analog lick"() -> (w1649:sgl[])
                n1081 = local read "Eye cam frame signal"() -> (w1647:i8[])
                n1082 = local read "ML signal"() -> (w1646:sgl[])
                n1083 = local read "Frame signal 2"() -> (w1645:i8[])
                n1084 = local read "Encoder signal"() -> (w1650:sgl[])
                n1085 = Decrement(x=w1665) -> (x-1=w1666:i32)
                n1086 = Index Array(array=w1664, index (row)=w1666, index (col)=0 ("disabled index (col)")) -> (element=w1648:i8)
                n1087 = Initialize Array(w1662, w1660) -> (w1657:sgl[])
                n1088 = Initialize Array(w1648, w1660) -> (w1651:i8[])
                n1089 = Build Array(w1650, w1661, w1659, w1658, w1657, w1654, w1653, w1652, w1651, w1649, w1647, w1646, w1645) -> (w1655:sgl[][])
                n1090 = local read "My tdms file"() -> (w1667:refnum<k34>)
                n1091 = disable-structure shown="Disabled" {
                  frame Disabled {
                    n1092 = local read "Gain"() -> ()  [unwired: 1 out]
                  }
                  frame Enabled {
                  }
                }
                n1093 = TDMS Write(0:w1667, 1:enum16{"decimated", "interleaved"}."decimated" ("data layout (0:decimated)"), 7:string[] ["Encoder signal", "Photo-diode", "Distance (cm)", "Photo stimulus signal", "Position in Unity", "Valve open", "Lick signal", "Frame signal", "Stimulus protocol", "Analog lick signal", "EyeCam frame signal", "Masking light signal", "Frame signal 2"] ("channel name(s) in (Untitled)"), 9:w1655) -> ()  [unwired: 2 in, 4 out]
              }
              frame False {
                # "Nora or Mate non VR"
                n1094 = local read "Encoder signal"() -> (w1671:sgl[])
                n1095 = local read "Photodiode signal"() -> (w1682:sgl[])
                n1096 = local read "total distance cm"() -> (w1680:sgl[])
                n1097 = local read "Photo stimulus signal"() -> (w1679:sgl[])
                n1098 = local read "Valve signal"() -> (w1676:i8[])
                n1099 = local read "lick signal"() -> (w1675:i8[])
                n1100 = local read "Frame signal"() -> (w1674:i8[])
                n1101 = local read "Trial type array"() -> (w1684:i8[][])
                n1102 = local read "All trials"() -> (w1670:i32)
                n1103 = local read "No. of smpl. per ch."() -> (w1681:i32)
                n1104 = local read "Eye cam frame signal"() -> (w1669:i8[])
                n1105 = Index Array(array=w1684, index (row)=w1670, index (col)=0 ("disabled index (col)")) -> (element=w1672:i8)
                n1106 = Initialize Array(w1672, w1681) -> (w1673:i8[])
                n1107 = Build Array(w1671, w1682, w1680, w1679, w1676, w1675, w1674, w1673, w1669) -> (w1677:sgl[][])
                n1108 = local read "My tdms file"() -> (w1685:refnum<k34>)
                n1109 = TDMS Write(0:w1685, 1:enum16{"decimated", "interleaved"}."decimated" ("data layout (0:decimated)"), 7:string[] ["Encoder signal", "Photo-diode", "Distance (cm)", "Photo stimulus signal", "Valve open", "Lick signal", "Frame signal", "Stimulus protocol", "EyeCam frame signal"] ("channel name(s) in (Untitled)"), 9:w1677) -> ()  [unwired: 2 in, 4 out]
              }
            }
          }
        }
        n1110 = case shown="False" w1536 {
          frame True {
          }
          frame False {
            n1111 = local read "prev. diode position"() -> (w1633:dbl)
            n1112 = local read "Distance (cm)"() -> (w1634:dbl)
            n1113 = Subtract(x=w1634, y=w1633) -> (x-y=w1632:dbl)
            n1114 = local write "Relative position"(w1632) -> ()
          }
        }
        n1115 = local read "index"() -> (w1591:i32)
        n1116 = Increment(x=w1591) -> (x+1=w1593:i32)
        n1117 = local read "delta distance cm"() -> (w1573:dbl[])
        n1118 = local read "No. of smpl. per ch."() -> (w1620:i32)
        n1119 = local write "index"(w1593) -> ()
        n1120 = local read "No. of smpl. per ch."() -> (w1566:i32)
        n1121 = local read "Loop rate"() -> (w1579:dbl)
        n1122 = local read "delta time (s)"() -> (w1583:dbl)
        n1123 = local read "No. of smpl. per ch."() -> (w1604:i32)
        n1124 = local read "encoder ticks per rev"() -> (w1543:dbl)
        n1125 = Add Array Elements(numeric array=w1573) -> (sum=w1576:dbl)
        n1126 = Array Size(array=w1573) -> (size(s)=w1575:i32)
        n1127 = local read "Store prev encoder count"() -> (w1569:dbl)
        n1128 = local read "Start time"() -> (w1600:u32)
        n1129 = call-poly <vilib>:"DAQmx Read.vi"("task/channels in"=w1617, "number of samples per channel"=w1620, "error in"=w1616) -> ("task out"=w1610:refnum<k21>, "data"=w1607:dbl[], "error out"=w1609:errorcluster)  [unwired: 10 in]
        n1130 = local read "Wheel circumference"() -> (w1624:dbl)
        n1131 = Divide(x=w1576, y=w1575) -> (x/y=w1574:dbl)
        n1132 = Divide(x=w1579, y=50.0) -> (x/y=w1577:dbl)
        n1133 = Add(x=w1588, y=w1574) -> (x+y=w1582:dbl)
        n1134 = Add(x=w1584, y=w1583) -> (x+y=w1581:dbl)
        n1135 = Subtract(x=w1607, y=40000.0) -> (x-y=w1539:dbl[])
        "Encoder signal" <- w1539
        n1136 = call-poly <vilib>:"DAQmx Read.vi"("task/channels in"=w1562, "number of samples per channel"=w1566, "error in"=w1565) -> ("task out"=w1559:refnum<k21>, "data"=w1526:dbl[][], "error out"=w1564:errorcluster)  [unwired: 10 in]
        n1137 = Index Array(array=w1526, index (row)=2 ("index")) -> (element=→"analog lick":dbl[])  [unwired: 1 in]
        n1138 = Index Array(array=w1526, index (row)=4 ("index")) -> (element=→"ML signal":dbl[])  [unwired: 1 in]
        n1139 = call-poly <vilib>:"DAQmx Read.vi"("task/channels in"=w1612, "number of samples per channel"=w1604, "error in"=w1611) -> ("task out"=w1603:refnum<k21>, "data"=w1518:u8[][], "error out"=w1602:errorcluster)  [unwired: 10 in]
        n1140 = local read "index"() -> (w1592:i32)
        n1141 = Tick Count (ms)() -> (millisecond timer value=w1606:u32)
        n1142 = Index Array(array=w1539, index=0) -> (element=w1568:dbl)
        n1143 = Subtract(x=w1606, y=w1600) -> (x-y=w1563:u32)
        "Experiment time (ms)" <- w1563
        n1144 = Divide(x=w1539, y=w1543) -> (x/y=w1626:dbl[])
        n1145 = Greater Or Equal?(x=w1592, y=w1577) -> (x >= y?=w1580:bool)
        n1146 = Add(x=w1569, y=w1568) -> (x+y=w1567:dbl)
        "Encoder count" <- w1567
        n1147 = Multiply(x=w1626, y=w1624) -> (x*y=w1542:dbl[])
        "total distance cm" <- w1542
        n1148 = Index Array(array=w1518, index (row)=1) -> (element=w1615:u8[])  [unwired: 1 in]
        n1149 = Index Array(array=w1518, index (row)=0) -> (element=w1554:u8[])  [unwired: 1 in]
        n1150 = Index Array(array=w1518, index (row)=3) -> (element=w1519:u8[])  [unwired: 1 in]
        n1151 = Index Array(array=w1526, index (row)=0 ("index")) -> (element=w1523:dbl[])  [unwired: 1 in]
        "Opt stim command" <- w1523
        n1152 = Index Array(array=w1526, index (row)=1 ("index")) -> (element=w1517:dbl[])  [unwired: 1 in]
        "Photodiode signal" <- w1517
        n1153 = Index Array(array=w1526, index (row)=3 ("index")) -> (element=w1529:dbl[])  [unwired: 1 in]
        n1154 = Subtract(x=w1563, y=w1599) -> (x-y=w1586:u32)
        "Delta time (ms)" <- w1586
        n1155 = case shown="True" w1580 {
          tunnel: [w1636 0.0] -> w1589
          tunnel: [w1637 0.0] -> w1590
          tunnel: w1582 -> [w1637 w1641]
          tunnel: w1581 -> [w1636 w1640]
          frame False {
          }
          frame True {
            n1156 = Divide(x=w1641, y=w1640) -> (x/y=w1638:dbl)
            "Velocity chart" <- w1638
            "Velocity chart 2" <- w1638
            n1157 = local write "index"(0 ("index")) -> ()
            n1158 = local write "velocity (cm/s)"(w1638) -> ()
          }
        }
        n1159 = Divide(x=w1615, y=32.0) -> (x/y=w1545:dbl[])
        "lick signal" <- w1545
        n1160 = local write "Photo stimulus signal"(w1523) -> ()
        n1161 = Index Array(array=w1542, index=0) -> (element=w1621:dbl)
        n1162 = Array Max & Min(array=w1517) -> (max value=w1516:dbl)  [unwired: 3 out]
        n1163 = Divide(x=w1554, y=16.0) -> (x/y=→"Frame signal":dbl[])
        n1164 = Divide(x=w1519, y=8.0) -> (x/y=→"Frame signal 2":dbl[])
        n1165 = Divide(x=w1529, y=3.3) -> (x/y=w1530:dbl[])
        n1166 = Quotient & Remainder(x=w1621, y=w1624) -> (x-y*floor(x/y)=→"Position on the wheel":dbl, floor(x/y)=→"Laps":dbl)
        n1167 = Round To Nearest(number=w1530) -> (nearest integer value=→"Eye cam frame signal":dbl[])
        n1168 = Divide(x=w1563, y=1000.0) -> (x/y=w1571:dbl)
        "Experiment time (s)" <- w1571
        n1169 = Divide(x=w1586, y=1000.0) -> (x/y=→"delta time (s)":dbl)
        n1170 = local read "Valve open"() -> (w1597:bool)
        n1171 = Index Array(array=w1518, index (row)=2) -> (element=w1551:u8[])  [unwired: 1 in]
        n1172 = Add Array Elements(numeric array=w1545) -> (sum=w1547:dbl)
        n1173 = Array Size(array=w1545) -> (size(s)=w1546:i32)
        n1174 = Index Array(array=w1545, index=0) -> (element=w1594:dbl)
        n1175 = Array Max & Min(array=w1542) -> (max value=w1541:dbl)  [unwired: 3 out]
        "Distance (cm)" <- w1541
        n1176 = Subtract(x=w1542, y=w1553) -> (x-y=→"delta distance cm":dbl[])
        n1177 = Greater?(x=w1516, y="Photo diode threshold") -> (0:w1552:bool)
        "Photodiode" <- w1552
        n1178 = Divide(x=w1547, y=w1546) -> (x/y=w1544:dbl)
        n1179 = Boolean To (0,1)(Boolean=w1597) -> (0, 1=w1595:i16)
        n1180 = case shown="True" w1552 {
          tunnel: w1541 -> [_ w1635]
          frame False {
          }
          frame True {
            n1181 = local write "prev. diode position"(w1635) -> ()
          }
        }
        n1182 = Array Max & Min(array=w1523) -> (max value=w1535:dbl)  [unwired: 3 out]
        n1183 = local read "Run experiment"() -> (w1631:bool)
        n1184 = Divide(x=w1551, y=64.0) -> (x/y=→"Valve signal":dbl[])
        n1185 = Divide(x=w1541, y=100.0) -> (x/y=→"Distance (m)":dbl)
        n1186 = Divide(x=w1571, y=60.0) -> (x/y=→"Time (min)":dbl)
        n1187 = Bundle(w1594, w1595) -> (→"Lick and reward chart" →"Lick and reward chart 2":cluster{dbl, i16})  [unwired: 1 in]
        n1188 = local write "Lick indicator"(w1544) -> ()
        n1189 = Greater?(x=w1535, y=0.5) -> (0:w1533:bool)
        n1190 = local write "Laser ON"(w1533) -> ()
        n1191 = Select(t=Record_enum."Record VR" ("Record enum"), s=w1631, f=Record_enum."Stop data acquision" ("Record enum")) -> (s? t:f=w1629:T5)
        "Record loop state" <- w1628
      }
      frame "Record" {
        n1192 = local write "Record loop state"(w1701) -> ()
        n1193 = local read "Run experiment"() -> (w1704:bool)
        n1194 = Select(t=Record_enum."Record" ("Record enum"), s=w1704, f=Record_enum."Stop data acquision" ("Record enum")) -> (s? t:f=w1702:T5)
      }
    }
    n1195 = local write "Exit program"("Exit program") -> ()
  }
  n1196 = while {
    shift-right: [w1717] -> _
    shift-left: T6."Idle" ("Eyecam states") -> [w1719]
    shift-right: [w1716] -> _
    shift-left: _ -> [w1710]
    shift-right: [w1715] -> _
    shift-left: _ -> [w1709]
    shift-right: [w1714] -> _
    shift-left: _ -> [w1708]
    shift-right: [w1713] -> _
    shift-left: _ -> [w1707]
    shift-right: [w1712] -> _
    shift-left: _ -> [w1706]
    shift-right: [w1711] -> _
    shift-left: _ -> [w1705]
    stop <- w1718 stop-if-true
    n1197 = case shown="\"Record pupille\"" w1719 {
      tunnel: [w1734 w1758 T6."Record pupille" ("Eyecam states") w1831 T6."Idle" ("Eyecam states")] -> w1717
      tunnel: [w1727 FALSE FALSE ("Exit") FALSE ("Exit") FALSE ("Exit")] -> w1718
      tunnel: [w1720 w1740 w1771 w1809 w1857] -> w1716
      tunnel: [w1721 "Black Level" w1770 w1808 w1856] -> w1715
      tunnel: [w1722 "Gain" w1769 w1807 w1855] -> w1714
      tunnel: [w1723 "Target frame rate" w1768 w1806 w1854] -> w1713
      tunnel: [w1724 "Image Format Control::Offset X" w1767 w1805 w1853] -> w1712
      tunnel: [w1725 "Image Format Control::Offset Y" w1766 w1804 w1852] -> w1711
      tunnel: w1710 -> [w1720 _ w1771 w1809 w1857]
      tunnel: w1709 -> [w1721 _ w1770 w1808 w1856]
      tunnel: w1708 -> [w1722 _ w1769 w1807 w1855]
      tunnel: w1707 -> [w1723 _ w1768 w1806 w1854]
      tunnel: w1706 -> [w1724 _ w1767 w1805 w1853]
      tunnel: w1705 -> [w1725 _ w1766 w1804 w1852]
      frame "Idle", Default {
        n1198 = Wait (ms)(milliseconds to wait=u32 10) -> ()  [unwired: 1 out]
        n1199 = local write "Pupille image"(T2 refnum ("Security cam image")) -> ()
        n1200 = local read "Record Button 2"() -> (w1733:bool)
        n1201 = local read "Eable eye cam"() -> (w1732:bool)
        n1202 = And(x=w1733, y=w1732) -> (x .and. y?=w1731:bool)
        n1203 = local read "Exit"() -> (w1727:bool)
        n1204 = Select(t=T6."Set params" ("Eyecam states"), s=w1731, f=T6."Idle" ("Eyecam states")) -> (s? t:f=w1734:T6)
      }
      frame "Set params" {
        n1205 = Divide(x=1000, y="Target frame rate") -> (x/y=w1748:dbl)
        n1206 = Multiply(x=0.9, y=w1748) -> (x*y=w1746:dbl)
        n1207 = call "Is Value Changed.vim"("value"="Target frame rate") -> ("changed or first call?"=w1743:bool)
        n1208 = case shown="True" w1743 {
          tunnel: w1746 -> [_ w1765]
          frame False {
          }
          frame True {
            n1209 = To Quad Integer(1:w1765) -> (0:w1764:i64)
            n1210 = property on="Exposure Time (ms)" class="Slide (strict)"("Maximum"=w1764, "Scale.Maximum"=w1764, "Value"=w1764) -> ()  [unwired: 2 in, 2 out]
          }
        }
        n1211 = local read "Run experiment"() -> (w1753:bool)
        n1212 = local read "Record Button 2"() -> (w1760:bool)
        n1213 = Multiply(x=1000.0, y="Exposure Time (ms)") -> (x*y=w1740:dbl)
        n1214 = local read "Exit"() -> (w1756:bool)
        n1215 = Not(x=w1760) -> (.not. x?=w1755:bool)
        n1216 = Compound Arithmetic op=OR(w1753, w1755, w1756) -> (w1757:bool)
        n1217 = call "Vision Acquisition"("Analog Control::Gain"="Gain", "Analog Control::Black Level"="Black Level", "Acquisition Control::Exposure Time"=w1740, "Acquisition Control::Acquisition Frame Rate"="Target frame rate", "Image Format Control::Offset X"="Image Format Control::Offset X", "Stop (F)"=w1757, "Image Format Control::Offset Y"="Image Format Control::Offset Y") -> ("Image Out"=w1762:T2, "Lost Image Count"=→"Lost Image Count":u32, "Total Images Transferred"=→"Total Images Transferred":u32, "Frame Rate"=→"Frame rate":dbl, "Stopped"=w1761:bool)  [unwired: 13 in, 3 out]
        n1218 = local write "Pupille image"(w1762) -> ()
        n1219 = Select(t=T6."Start recording" ("Eyecam states"), s=w1753, f=T6."Idle" ("Eyecam states")) -> (s? t:f=w1752:T6)
        n1220 = Select(t=w1752, s=w1761, f=T6."Set params" ("Eyecam states")) -> (s? t:f=w1758:T6)
      }
      frame "Start recording" {
        # "Wait to make sure DAQ recording \nis started before saving images"
        n1221 = local read "Record"() -> (w1772:bool)
        n1222 = case shown="True" w1772 {
          frame False {
          }
          frame True {
            n1223 = Get Volume Info(11:path "C:/" ("path")) -> (1:w1790:i64)  [unwired: 1 in, 5 out]
            n1224 = Divide(x=w1790, y=i64 1024) -> (x/y=w1794:dbl)
            n1225 = Divide(x=w1794, y=i64 1024) -> (x/y=w1795:dbl)
            n1226 = Divide(x=w1795, y=i64 1024) -> (x/y=w1786:dbl)
            n1227 = Number To Fractional String(number=w1786, precision (6)=i16 1) -> (F-format string=w1787:string)  [unwired: 2 in]
            n1228 = Concatenate Strings("Pupil is beeing recorded! \nAvailable disk space: " ("string"), w1787, " GB" ("string")) -> (w1784:string)
            n1229 = One Button Dialog(message=w1784) -> ()  [unwired: 1 in, 1 out]
          }
        }
        n1230 = property on="Image Format Control::Offset X" class="Slide (strict)"("DisabledEnum"=T7."Disabled and Grayed Out" ("Disabled")) -> ()  [unwired: 2 in, 2 out]
        n1231 = property on="Image Format Control::Offset Y" class="Slide (strict)"("DisabledEnum"=T7."Disabled and Grayed Out" ("Disabled")) -> ()  [unwired: 2 in, 2 out]
        n1232 = local read "Pupil Exp day folder"() -> (w1773:path)
        n1233 = call <vilib>:"Check if File or Folder Exists.vi"("path"=w1773) -> ("file or folder exists?"=w1775:bool, "dup path"=w1774:path)  [unwired: 8 in, 1 out]
        n1234 = property on="Gain" class="Slide (strict)"("DisabledEnum"=T7."Disabled and Grayed Out" ("Disabled")) -> ()  [unwired: 2 in, 2 out]
        n1235 = property on="Target frame rate" class="DigNum (strict)"("DisabledEnum"=T7."Disabled and Grayed Out" ("Disabled")) -> ()  [unwired: 2 in, 2 out]
        n1236 = while {
          stop <- w1801 stop-if-true
          n1237 = Wait (ms)(milliseconds to wait=u32 10) -> ()  [unwired: 1 out]
          n1238 = local read "Record loop state"() -> (w1803:T5)
          n1239 = Equal?(x=w1803, y=Record_enum."Record VR" ("Record loop state")) -> (x = y?=w1801:bool)
        }
        n1240 = case shown="False" w1775 {
          tunnel: [w1797 w1799] -> _
          tunnel: w1774 -> [w1797 w1798]
          frame True {
          }
          frame False {
            n1241 = Create Folder(path (use dialog)=w1798) -> (created path=w1799:path)  [unwired: 2 in, 2 out]
          }
        }
        n1242 = property on="Exposure Time (ms)" class="Slide (strict)"("DisabledEnum"=T7."Disabled and Grayed Out" ("Disabled")) -> ()  [unwired: 2 in, 2 out]
        n1243 = property on="Black Level" class="Slide (strict)"("DisabledEnum"=T7."Disabled and Grayed Out" ("Disabled")) -> ()  [unwired: 2 in, 2 out]
      }
      frame "Record pupille" {
        n1244 = disable-structure shown="Enabled" {
          disable-tunnel: [w1845 w1846] -> w1837
          disable-tunnel: [w1844 w1847] -> w1836
          disable-tunnel: [w1843 w1848] -> w1834
          disable-tunnel: [w1842 w1849] -> w1833
          disable-tunnel: [w1841 w1850] -> w1832
          disable-tunnel: [w1838 w1851] -> w1810
          disable-tunnel: w1809 -> [_ w1851]
          disable-tunnel: w1808 -> [_ w1850]
          disable-tunnel: w1807 -> [_ w1849]
          disable-tunnel: w1806 -> [_ w1848]
          disable-tunnel: w1805 -> [_ w1847]
          disable-tunnel: w1804 -> [_ w1846]
          frame Disabled {
            n1245 = local read "Exposure Time (ms)"() -> (w1839:dbl)
            n1246 = local read "Image Format Control::Offset X"() -> (w1844:i64)
            n1247 = local read "Image Format Control::Offset Y"() -> (w1845:i64)
            n1248 = local read "Black Level"() -> (w1841:dbl)
            n1249 = local read "Target frame rate"() -> (w1843:dbl)
            n1250 = local read "Gain"() -> (w1842:dbl)
            n1251 = Multiply(x=1000.0, y=w1839) -> (x*y=w1838:dbl)
          }
          frame Enabled {
          }
        }
        n1252 = local read "Run experiment"() -> (w1829:bool)
        n1253 = local read "Exit"() -> (w1828:bool)
        n1254 = Not(x=w1829) -> (.not. x?=w1827:bool)
        n1255 = Compound Arithmetic op=OR(w1827, w1828) -> (w1826:bool)
        n1256 = call "Vision Acquisition3"("Analog Control::Gain"=w1833, "Analog Control::Black Level"=w1832, "Acquisition Control::Exposure Time"=w1810, "Acquisition Control::Acquisition Frame Rate"=w1834, "Image Format Control::Offset X"=w1836, "Stop (F)"=w1826, "Image Format Control::Offset Y"=w1837) -> ("Image Out"=w1825:T2, "Lost Image Count"=w1811:u32, "Total Images Transferred"=w1812:u32, "Frame Rate"=w1835:dbl, "Stopped"=w1824:bool)  [unwired: 13 in, 3 out]
        n1257 = local write "Frame rate"(w1835) -> ()
        n1258 = local write "Pupille image"(w1825) -> ()
        n1259 = local write "Lost Image Count"(w1811) -> ()
        n1260 = local write "Total Images Transferred"(w1812) -> ()
        n1261 = local read "Pupil Exp day folder"() -> (w1820:path)
        n1262 = local read "Run experiment"() -> (w1815:bool)
        n1263 = local read "Exit"() -> (w1817:bool)
        n1264 = local read "Record"() -> (w1814:bool)
        n1265 = local read "Filename"() -> (w1818:string)
        n1266 = Not(x=w1817) -> (.not. x?=w1816:bool)
        n1267 = Compound Arithmetic op=AND(w1814, w1815, w1816) -> (w1813:bool)
        n1268 = call "SavePupilCameraImages.vi"("Save Format"=enum16{"Png", "Raw"}."Raw", "Save Image?"=w1813, "Block Folder"=w1820, "Subfolder"=w1818, "Refnum in"=w1825) -> ("ImageSaved"=w1819:bool)  [unwired: 5 in, 1 out]
        n1269 = local write "Pupille image saved"(w1819) -> ()
        n1270 = Select(t=T6."Stop recording" ("Eyecam states"), s=w1824, f=T6."Record pupille" ("Eyecam states")) -> (s? t:f=w1831:T6)
      }
      frame "Stop recording" {
        w1858 = FALSE ("Record Button 2")
        n1271 = property on="Image Format Control::Offset X" class="Slide (strict)"("DisabledEnum"=T7."Enabled" ("Disabled")) -> ()  [unwired: 2 in, 2 out]
        n1272 = property on="Image Format Control::Offset Y" class="Slide (strict)"("DisabledEnum"=T7."Enabled" ("Disabled")) -> ()  [unwired: 2 in, 2 out]
        n1273 = local write "Record Button 2"(w1858) -> ()
        n1274 = local write "Pupille image saved"(w1858) -> ()
        n1275 = property on="Gain" class="Slide (strict)"("DisabledEnum"=T7."Enabled" ("Disabled")) -> ()  [unwired: 2 in, 2 out]
        n1276 = property on="Target frame rate" class="DigNum (strict)"("DisabledEnum"=T7."Enabled" ("Disabled")) -> ()  [unwired: 2 in, 2 out]
        n1277 = property on="Exposure Time (ms)" class="Slide (strict)"("DisabledEnum"=T7."Enabled" ("Disabled")) -> ()  [unwired: 2 in, 2 out]
        n1278 = property on="Black Level" class="Slide (strict)"("DisabledEnum"=T7."Enabled" ("Disabled")) -> ()  [unwired: 2 in, 2 out]
      }
    }
    "Eyecam states" <- w1717
  }
  n1279 = while {
    stop <- w1870 stop-if-true
    n1280 = local read "Eable security cam"() -> (w1868:bool)
    n1281 = local read "Cam ON /OFF"() -> (w1869:bool)
    n1282 = Wait (ms)(milliseconds to wait=u32 20) -> ()  [unwired: 1 out]
    n1283 = And(x=w1869, y=w1868) -> (x .and. y?=w1867:bool)
    n1284 = case shown="False" w1867 {
      frame False {
        n1285 = local write "Security cam image"(T2 refnum ("Security cam image")) -> ()
      }
      frame True {
        n1286 = while {
          stop <- w1874 stop-if-true
          n1287 = local read "Cam ON /OFF"() -> (w1880:bool)
          n1288 = Not(x=w1880) -> (.not. x?=w1879:bool)
          n1289 = call "Vision Acquisition2"("Stop (F)"=w1879) -> ("Image Out"=→"Security cam image":T2, "Stopped"=w1876:bool, "error out"=w1878:errorcluster)  [unwired: 24 in]
          n1290 = local read "Exit"() -> (w1873:bool)
          n1291 = call <vilib>:"Find First Error.vi"("error in (no error)"=w1878) -> ("error?"=w1875:bool)  [unwired: 3 in, 1 out]
          n1292 = Compound Arithmetic op=OR(w1875, w1876, w1873) -> (w1874:bool)
        }
      }
    }
    n1293 = local read "Exit"() -> (w1870:bool)
  }
  n1294 = while {
    shift-right: [w1886] -> _
    shift-left: _ -> [w1885]
    shift-right: [w1887] -> _
    shift-left: _ -> [w1884]
    shift-right: [w1882] -> _
    shift-left: w129 -> [w1883]
    stop <- w1881 stop-if-true
    n1295 = case shown="\"Socket connected\"" w1883 {
      tunnel: [w1895 w1931 w2027 w2038] -> w1887
      tunnel: [w1896 w1933 w2028 w2039] -> w1886
      tunnel: w1885 -> [_ w1933 w2030 w2039]
      tunnel: w1884 -> [_ w1931 w2029 w2038]
      tunnel: [w1892 w1930 Socket_enum."Socket not connected" ("Enum") w2037] -> w1882
      tunnel: [w1891 FALSE FALSE ("Exit") w2033] -> w1881
      frame "Init socket", Default {
        n1296 = local read "Unity connected"() -> (w1890:bool)
        n1297 = local write "Read loop stopped"(FALSE ("Read loop stopped")) -> ()
        n1298 = local write "Write loop stopped"(FALSE ("Read loop stopped")) -> ()
        n1299 = local write "Unity connected"(FALSE ("Unity connected")) -> ()
        n1300 = case shown="False" w1890 {
          frame False {
            n1301 = flat-sequence {
              frame #0 {
                n1302 = Wait (ms)(milliseconds to wait=u32 200) -> ()  [unwired: 1 out]
              }
              frame #1 {
                n1303 = local read "command line"() -> (w1903:string)
                n1304 = property on="working directory 2" class="Path"("Visible"=FALSE) -> ()  [unwired: 2 in, 2 out]
                n1305 = call <vilib>:"System Exec.vi"("run minimized? (F)"=FALSE, "wait until completion? (T)"=FALSE, "working directory"="working directory 2", "command line"=w1903) -> ()  [unwired: 4 in, 4 out]
              }
              frame #2 {
                n1306 = Wait (ms)(milliseconds to wait=u32 800) -> ()  [unwired: 1 out]
              }
            }
          }
          frame True {
          }
        }
        n1307 = call <vilib>:"TCP Listen.vi"("timeout ms (wait forever: -1)"=10000, "port"=u16 11000) -> ("error out"=w1893:errorcluster, "connection ID"=w1894:refnum<k5>)  [unwired: 5 in, 3 out]
        n1308 = case shown="No Error" w1893 {
          tunnel: [w1916 w1922] -> w1896
          tunnel: [w1915 w1921] -> w1895
          tunnel: w1894 -> [w1914 w1922]
          tunnel: w1893 -> [w1913 w1921]
          tunnel: [Socket_enum."Socket connected" ("Enum") w1919] -> w1892
          frame No Error {
            n1309 = TCP Write(connection ID=w1914, data in="Start", error in (no error)=w1913, 9:-1 ("timeout ms (25000)")) -> (connection ID out=w1910:refnum<k5>, error out=w1908:errorcluster)  [unwired: 1 out]
            n1310 = TCP Write(connection ID=w1910, data in="Start", error in (no error)=w1908) -> (connection ID out=w1916:refnum<k5>, error out=w1915:errorcluster)  [unwired: 1 in, 1 out]
          }
          frame Error {
            n1311 = local read "VR Mode"() -> (w1920:bool)
            n1312 = Select(t=Socket_enum."Init socket" ("Enum"), s=w1920, f=Socket_enum."Socket not connected" ("Enum")) -> (s? t:f=w1919:T9)
          }
        }
        n1313 = local read "Exit"() -> (w1891:bool)
      }
      frame "Socket connected" {
        n1314 = Tick Count (ms)() -> (millisecond timer value=w1923:u32)
        n1315 = while {
          tunnel: w1933 -> [w1990]
          tunnel: w1931 -> [w1989]
          stop <- w1987 stop-if-true
          n1316 = local read "Write"() -> (w1988:bool)
          n1317 = case shown="True" w1988 {
            tunnel: w1990 -> [_ w2001]
            tunnel: w1989 -> [_ w1998]
            tunnel: [w1991 w1999] -> w1987
            frame False {
              n1318 = local read "Exit"() -> (w1991:bool)
            }
            frame True {
              n1319 = local read "Encoder count"() -> (w1993:dbl)
              n1320 = case shown="False" FALSE {
                tunnel: w1993 -> [w2006 w2009]
                tunnel: [w2005 w2008] -> w1994
                frame False {
                  n1321 = local read "encoder ticks per rev"() -> (w2004:dbl)
                  n1322 = Divide(x=4000.0 ("y"), y=w2004) -> (x/y=w2002:dbl)
                  n1323 = Multiply(x=w2002, y=w2006) -> (x*y=w2005:dbl)
                }
                frame True {
                  n1324 = local read "Gain"() -> (w2010:dbl)
                  n1325 = Multiply(x=w2010, y=w2009) -> (x*y=w2007:dbl)
                  n1326 = To Long Integer(number=w2007) -> (32bit integer=w2008:i32)
                }
              }
              n1327 = local read "Read loop stopped"() -> (w1995:bool)
              n1328 = local read "Stop Unity"() -> (w1997:bool)
              n1329 = And(x=w1997, y=w1995) -> (x .and. y?=w1996:bool)
              n1330 = case shown="False" w1996 {
                tunnel: ["ext,\r\n" w2023] -> w2000
                tunnel: w1994 -> [_ w2022]
                tunnel: [TRUE FALSE] -> w1999
                frame True {
                  n1331 = local write "Write loop stopped"(TRUE ("Read loop stopped")) -> ()
                  n1332 = local write "Write"(FALSE ("Write")) -> ()
                  n1333 = local write "Unity connected"(FALSE ("Unity connected")) -> ()
                  n1334 = Wait (ms)(milliseconds to wait=u32 20) -> ()  [unwired: 1 out]
                }
                frame False {
                  n1335 = local read "offset tag"() -> (w2017:string)
                  n1336 = local read "msg tag"() -> (w2018:string)
                  n1337 = Number To Decimal String(number=w2022) -> (decimal integer string=w2020:string)  [unwired: 1 in]
                  n1338 = Concatenate Strings(w2018, w2017, w2020, "\r\n" ("string")) -> (w2023:string)
                }
              }
              n1339 = TCP Write(connection ID=w2001, data in=w2000, error in (no error)=w1998) -> ()  [unwired: 1 in, 3 out]
            }
          }
          n1340 = Wait (ms)(milliseconds to wait=u32 5) -> ()  [unwired: 1 out]
        }
        n1341 = while {
          tunnel: w1933 -> [w1940]
          tunnel: w1931 -> [w1941]
          shift-right: [w1935] -> _
          shift-left: w1923 -> [w1936]
          stop <- w1939 stop-if-true
          n1342 = local read "read"() -> (w1938:bool)
          n1343 = case shown="True" w1938 {
            tunnel: w1940 -> [_ w1955]
            tunnel: w1941 -> [_ w1956]
            tunnel: [w1944 FALSE] -> w1939
            frame False {
              n1344 = disable-structure shown="Disabled" {
                frame Disabled {
                  n1345 = local write "msg tag"("str," ("msg tag")) -> ()
                }
                frame Enabled {
                }
              }
              n1346 = local write "Read loop stopped"(TRUE ("Read loop stopped")) -> ()
              n1347 = local read "Exit"() -> (w1944:bool)
            }
            frame True {
              # "Correction factor"
              # "msg format: pos + CorridorIndicator + \",\" Position"
              n1348 = TCP Read(connection ID=w1955, bytes to read=20, error in (no error)=w1956, 7:T17."CRLF" ("mode (standard)"), 9:-1 ("timeout ms (25000)")) -> (data out=w1964:string)  [unwired: 2 out]
              n1349 = Match Pattern(string=w1964, regular expression=",", offset (0)=0) -> (after substring=w1970:string)  [unwired: 3 out]
              n1350 = Match Pattern(string=w1964, regular expression="pos") -> (after substring=w1961:string)  [unwired: 1 in, 3 out]
              n1351 = Match Pattern(string=w1961, regular expression="," ("after substring")) -> (before substring=w1960:string)  [unwired: 1 in, 3 out]
              n1352 = Match Pattern(string=w1970, regular expression="\\r\\n" ("after substring")) -> (before substring=w1968:string)  [unwired: 1 in, 3 out]
              n1353 = Decimal String To Number(string=w1960) -> (number=w1950:i32)  [unwired: 2 in, 1 out]
              n1354 = Fract/Exp String To Number(string=w1968) -> (number=w1959:dbl)  [unwired: 3 in, 1 out]
              n1355 = disable-structure shown="Disabled" {
                disable-tunnel: w1959 -> [w1972 _]
                frame Disabled {
                  "Raw position:" <- w1972
                }
                frame Enabled {
                }
              }
              n1356 = Add(x=0.0 ("Correction factor"), y=w1959) -> (x+y=w1966:dbl)
              n1357 = Greater?(x=w1966, y=10.0) -> (0:w1967:bool)
              n1358 = case shown="True" w1967 {
                tunnel: w1966 -> [w1974 w1985]
                tunnel: [w1974 w1984] -> w1949
                tunnel: w1950 -> [w1973 w1975]
                tunnel: [w1973 w1975] -> _
                frame False {
                }
                frame True {
                  n1359 = local read "Corridor length"() -> (w1983:i32)
                  n1360 = local read "offset tag"() -> (w1980:string)
                  n1361 = Decimal String To Number(string=w1980) -> (number=w1979:i32)  [unwired: 2 in, 1 out]
                  n1362 = Subtract(x=w1983, y=60) -> (x-y=w1977:i32)
                  n1363 = Multiply(x=w1979, y=10) -> (x*y=w1981:i32)
                  n1364 = Add(x=w1977, y=w1981) -> (x+y=w1976:i32)
                  n1365 = Subtract(x=w1985, y=w1976) -> (x-y=w1984:dbl)
                }
              }
              n1366 = local read "reward zone start"() -> (w1947:dbl)
              n1367 = local write "Read loop stopped"(FALSE ("Read loop stopped")) -> ()
              n1368 = Add(x=w1949, y=w1947) -> (x+y=w1946:dbl)
              "?" <- w1946
              "Unity position:" <- w1946
              n1369 = local write "Relative position"(w1946) -> ()
            }
          }
          n1370 = local write "Unity connected"(TRUE ("Unity connected")) -> ()
          n1371 = Tick Count (ms)() -> (millisecond timer value=w1935:u32)
          n1372 = Subtract(x=w1935, y=w1936) -> (x-y=→"Socket read loop rate":u32)
          n1373 = Wait (ms)(milliseconds to wait=u32 1) -> ()  [unwired: 1 out]
        }
        n1374 = local read "Stop Unity"() -> (w1927:bool)
        n1375 = local read "Exit"() -> (w1926:bool)
        n1376 = Compound Arithmetic op=OR(w1926, w1927) -> (w1925:bool)
        n1377 = Wait (ms)(milliseconds to wait=u32 10) -> ()  [unwired: 1 out]
        n1378 = Select(t=Socket_enum."Close socket" ("Enum"), s=w1925, f=Socket_enum."Socket connected" ("Enum")) -> (s? t:f=w1930:T9)
      }
      frame "Close socket" {
        n1379 = TCP Close Connection(connection ID=w2030, error in (no error)=w2029) -> (connection ID out=w2028:refnum<k5>, error out=w2027:errorcluster)  [unwired: 1 in]
        n1380 = local write "Unity connected"(FALSE ("Unity connected")) -> ()
      }
      frame "Socket not connected" {
        n1381 = local write "Unity connected"(FALSE ("Unity connected")) -> ()
        n1382 = Wait (ms)(milliseconds to wait=u32 1000) -> ()  [unwired: 1 out]
        n1383 = local read "VR Mode"() -> (w2036:bool)
        n1384 = local read "Exit"() -> (w2033:bool)
        n1385 = Select(t=Socket_enum."Init socket" ("Enum"), s=w2036, f=Socket_enum."Socket not connected" ("Enum")) -> (s? t:f=w2037:T9)
      }
    }
  }
  n1386 = property on="Shuffle" class="Bool (strict)"("Visible"=FALSE) -> ()  [unwired: 2 in, 2 out]
  n1387 = property on="Exit" class="Bool (strict)"("Visible"=FALSE) -> ()  [unwired: 2 in, 2 out]
  n1388 = property on="Stop Unity" class="Bool (strict)"("Visible"=FALSE) -> ()  [unwired: 2 in, 2 out]
  n1389 = local write "Exit program"(FALSE ("Exit program")) -> ()
  n1390 = local write "Stop Unity"(FALSE ("Stop Unity")) -> ()
  n1391 = local write "Exit"(FALSE ("Exit")) -> ()
  n1392 = local write "Record"(FALSE ("Logg data")) -> ()
  n1393 = local write "Reward given"(FALSE ("Reward given")) -> ()
  n1394 = local write "Start recording"(FALSE ("Start recording")) -> ()
  n1395 = local write "Record Button"(FALSE ("Record Button")) -> ()
  n1396 = local write "Gain"(1.0 ("Gain")) -> ()
  n1397 = property on="Write" class="Bool (strict)"("Visible"=FALSE) -> ()  [unwired: 2 in, 2 out]
  n1398 = property on="read" class="Bool (strict)"("Visible"=FALSE) -> ()  [unwired: 2 in, 2 out]
  n1399 = local read "Stim prot command"() -> (w64:u16)
  n1400 = local read "Stim prot command"() -> (w26:u16)
  n1401 = local read "protocol array"() -> (w68:string[][])
  n1402 = local read "protocol array"() -> (w23:string[][])
  n1403 = property on="total distance cm" class="Arr (strict)"("Visible"=FALSE) -> ()  [unwired: 2 in, 2 out]
  n1404 = property on="Experiment time (s)" class="DigNum (strict)"("Visible"=FALSE) -> ()  [unwired: 2 in, 2 out]
  n1405 = local write "Store prev encoder count"(0.0 ("Store prev encoder count")) -> ()
  n1406 = property on="Store prev encoder count" class="DigNum (strict)"("Visible"=FALSE) -> ()  [unwired: 2 in, 2 out]
  n1407 = property on="My tdms file" class="Ref (strict)"("Visible"=FALSE) -> ()  [unwired: 2 in, 2 out]
  n1408 = disable-structure shown="Disabled" {
    frame Disabled {
      n1409 = local read "total distance cm"() -> (w2040:sgl[])
      n1410 = local read "prev. diode position"() -> (w2043:dbl)
      n1411 = local read item#-1() -> (w2042)
      n1412 = Array Max & Min(array=w2040) -> ()  [unwired: 4 out]
      n1413 = Subtract(y=w2043) -> (x-y=w2041:dbl)  [unwired: 1 in]
      n1414 = Greater?(x=w2041, y=w2042) -> ()  [unwired: 1 out]
    }
    frame Enabled {
    }
  }
  n1415 = Index Array(array=w68, index (row)=w64, index (col)=0 ("index (row)")) -> (element=w61:string)
  n1416 = Index Array(array=w68, index (row)=w64, index (col)=1 ("disabled index (col)")) -> (element=w52:string)
  n1417 = Index Array(array=w68, index (row)=w64, index (col)=2 ("disabled index (col)")) -> (element=w47:string)
  n1418 = Index Array(array=w68, index (row)=w64, index (col)=3 ("disabled index (col)")) -> (element=w46:string)
  n1419 = Index Array(array=w23, index (row)=w26, index (col)=0 ("index (row)")) -> (element=w29:string)
  n1420 = Index Array(array=w23, index (row)=w26, index (col)=1 ("disabled index (col)")) -> (element=w38:string)
  n1421 = Index Array(array=w23, index (row)=w26, index (col)=2 ("disabled index (col)")) -> (element=w43:string)
  n1422 = local write "Open valve"(FALSE ("Open valve")) -> ()
  n1423 = local write "Reward freq. (cm)"(100.0 ("Reward freq. (cm)")) -> ()
  n1424 = local write "Timed reward (s)"(u32 0 ("Timed reward (s)")) -> ()
  n1425 = local write "random rew"(0.5 ("random rew")) -> ()
  n1426 = Match Pattern(string=w61, regular expression=w57) -> (match substring=w58:string)  [unwired: 1 in, 3 out]
  n1427 = Match Pattern(string=w61, regular expression=" Hz") -> (before substring=w62:string)  [unwired: 1 in, 3 out]
  n1428 = Match Pattern(string=w61, regular expression=w59) -> (match substring=w60:string)  [unwired: 1 in, 3 out]
  n1429 = Match Pattern(string=w52, regular expression="from ") -> (after substring=w55:string)  [unwired: 1 in, 3 out]
  n1430 = Match Pattern(string=w52, regular expression=w53) -> (match substring=w54:string)  [unwired: 1 in, 3 out]
  n1431 = Match Pattern(string=w47, regular expression="to ") -> (after substring=w49:string)  [unwired: 1 in, 3 out]
  n1432 = Match Pattern(string=w47, regular expression=w51) -> (match substring=w50:string)  [unwired: 1 in, 3 out]
  n1433 = Match Pattern(string=w46, regular expression=" %") -> (before substring=w44:string)  [unwired: 1 in, 3 out]
  n1434 = Match Pattern(string=w29, regular expression=w33) -> (match substring=w32:string)  [unwired: 1 in, 3 out]
  n1435 = Match Pattern(string=w29, regular expression=" Hz") -> (before substring=w28:string)  [unwired: 1 in, 3 out]
  n1436 = Match Pattern(string=w29, regular expression=w31) -> (match substring=w30:string)  [unwired: 1 in, 3 out]
  n1437 = Match Pattern(string=w38, regular expression="from ") -> (after substring=w35:string)  [unwired: 1 in, 3 out]
  n1438 = Match Pattern(string=w38, regular expression=w37) -> (match substring=w36:string)  [unwired: 1 in, 3 out]
  n1439 = Match Pattern(string=w43, regular expression="to ") -> (after substring=w41:string)  [unwired: 1 in, 3 out]
  n1440 = Match Pattern(string=w43, regular expression=w39) -> (match substring=w40:string)  [unwired: 1 in, 3 out]
  n1441 = local write "Water cnt. reset"(0 ("Waret received")) -> ()
  n1442 = call-poly <vilib>:"DAQmx Create Virtual Channel.vi"("lines"=tag "Dev1/port2/line6") -> ("task out"=w101:refnum<k21>)  [unwired: 13 in, 1 out]
  n1443 = call-poly <vilib>:"DAQmx Create Virtual Channel.vi"("lines"=tag "Dev1/port2/line5") -> ("task out"=w103:refnum<k21>)  [unwired: 13 in, 1 out]
  n1444 = local write "Valve open"(FALSE ("Valve open")) -> ()
  n1445 = local write "Repetition"(2 ("Repetition")) -> ()
  n1446 = local write "miss trial"(FALSE ("miss trial")) -> ()
  n1447 = property on="Water cnt. reset" class="DigNum (strict)"("Visible"=FALSE) -> ()  [unwired: 2 in, 2 out]
  n1448 = property on="sound cue presented" class="Bool (strict)"("Visible"=FALSE) -> ()  [unwired: 2 in, 2 out]
  n1449 = Equal?(x=w58, y=w57) -> ()  [unwired: 1 out]
  n1450 = Equal?(x=w60, y=w59) -> ()  [unwired: 1 out]
  n1451 = Equal?(x=w54, y=w53) -> ()  [unwired: 1 out]
  n1452 = Equal?(x=w50, y=w51) -> ()  [unwired: 1 out]
  n1453 = Equal?(x=w32, y=w33) -> ()  [unwired: 1 out]
  n1454 = Equal?(x=w30, y=w31) -> ()  [unwired: 1 out]
  n1455 = Equal?(x=w36, y=w37) -> ()  [unwired: 1 out]
  n1456 = Equal?(x=w40, y=w39) -> ()  [unwired: 1 out]
  n1457 = Decimal String To Number(string=w62) -> ()  [unwired: 2 in, 2 out]
  n1458 = Decimal String To Number(string=w55) -> ()  [unwired: 2 in, 2 out]
  n1459 = Decimal String To Number(string=w49) -> ()  [unwired: 2 in, 2 out]
  n1460 = Decimal String To Number(string=w44) -> ()  [unwired: 2 in, 2 out]
  n1461 = Decimal String To Number(string=w28) -> ()  [unwired: 2 in, 2 out]
  n1462 = Decimal String To Number(string=w35) -> ()  [unwired: 2 in, 2 out]
  n1463 = Decimal String To Number(string=w41) -> ()  [unwired: 2 in, 2 out]
  n1464 = Tick Count (ms)() -> (millisecond timer value=w88:u32)
  n1465 = disable-structure shown="Disabled" {
    frame Disabled {
      w2047 = 10.0 ("y")
      n1466 = local read "delta distance cm"() -> (w2050:dbl[])
      n1467 = local read "delta time (s)"() -> (w2051:dbl)
      n1468 = local read "index"() -> (w2053:i32)
      n1469 = Increment(x=w2053) -> (x+1=w2044:i32)
      n1470 = Insert Into Array(index=w2053, new element=w2050) -> (w2052:dbl[])  [unwired: 1 in]
      n1471 = Insert Into Array(index=w2053, new element=w2051) -> (w2049:dbl[])  [unwired: 1 in]
      n1472 = local write "index"(w2044) -> ()
      n1473 = local read "index"() -> (w2045:i32)
      n1474 = Array Size(array=w2049) -> (size(s)=w2046:i32)
      n1475 = Greater Or Equal?(x=w2045, y=w2047) -> ()  [unwired: 1 out]
      n1476 = Equal?(x=w2046, y=w2047) -> (x = y?=w2048:bool)
      n1477 = case shown="True" w2048 {
        tunnel: w2052 -> [w2055 w2057]
        tunnel: [w2055 _] -> _
        tunnel: [w2054 _] -> _
        tunnel: w2049 -> [w2054 w2058]
        tunnel: [_ 0.0] -> _
        frame False {
        }
        frame True {
          n1478 = Index Array(array=w2057, index=9) -> ()  [unwired: 1 out]
          n1479 = Index Array(array=w2058, index=9) -> ()  [unwired: 1 out]
        }
      }
      n1480 = call-poly <vilib>:"Mean.vi"() -> ()  [unwired: 1 in, 2 out]
    }
    frame Enabled {
    }
  }
  n1481 = while {
    tunnel: w103 -> [w2080]
    tunnel: w101 -> [w2070]
    shift-right: [w2072] -> _
    shift-left: w88 -> [w2071]
    shift-right: [w2062] -> _
    shift-left: _ -> [w2061]
    stop <- w2087 stop-if-true
    n1482 = local read "Repetition"() -> (w2082:i32)
    n1483 = local read "Reward zone"() -> (w2074:bool)
    n1484 = case shown="False" w2074 {
      tunnel: [TRUE w2143] -> w2085
      tunnel: [w2098 w2142] -> w2075
      tunnel: w2061 -> [w2095 _]
      frame False {
        n1485 = local read "Random reward"() -> (w2096:bool)
        n1486 = case shown="True" w2096 {
          tunnel: [w2100 w2119] -> w2098
          tunnel: w2095 -> [w2101 w2127]
          frame True {
            n1487 = local read "Timed reward (s)"() -> (w2110:u32)
            n1488 = local read "Reward freq. (cm)"() -> (w2115:dbl)
            n1489 = local read "random rew"() -> (w2113:dbl)
            n1490 = local read "Prev. rew. pos."() -> (w2117:dbl)
            n1491 = local read "Distance (cm)"() -> (w2118:dbl)
            n1492 = Tick Count (ms)() -> (millisecond timer value=w2109:u32)
            n1493 = Multiply(x=w2110, y=u32 1000) -> (x*y=w2106:u32)
            n1494 = Multiply(x=w2115, y=2.0) -> (x*y=w2112:dbl)
            n1495 = Add(x=w2101, y=w2106) -> (x+y=w2108:u32)
            n1496 = Multiply(x=w2112, y=w2113) -> (x*y=w2111:dbl)
            n1497 = Greater?(x=w2106, y=u32 999) -> (0:w2105:bool)
            n1498 = Greater?(x=w2109, y=w2108) -> (0:w2107:bool)
            n1499 = Add(x=w2117, y=w2111) -> (x+y=w2116:dbl)
            n1500 = And(x=w2107, y=w2105) -> (x .and. y?=w2104:bool)
            n1501 = Greater?(x=w2118, y=w2116) -> (0:w2099:bool)
            n1502 = Or(x=w2099, y=w2104) -> (x .or. y?=w2100:bool)
          }
          frame False {
            n1503 = local read "Timed reward (s)"() -> (w2130:u32)
            n1504 = local read "Reward freq. (cm)"() -> (w2134:dbl)
            n1505 = local read "Reward freq. (cm)"() -> (w2138:dbl)
            n1506 = local read "Prev. rew. pos."() -> (w2135:dbl)
            n1507 = local read "Distance (cm)"() -> (w2136:dbl)
            n1508 = local read "Prev. rew. pos."() -> (w2139:dbl)
            n1509 = local read "Distance (cm)"() -> (w2140:dbl)
            n1510 = Tick Count (ms)() -> (millisecond timer value=w2128:u32)
            n1511 = Multiply(x=w2130, y=u32 1000) -> (x*y=w2124:u32)
            n1512 = Add(x=w2127, y=w2124) -> (x+y=w2126:u32)
            n1513 = Compound Arithmetic op=ADD(w2135, w2134, 20.0 ("value")) -> (w2132:dbl)
            n1514 = Add(x=w2139, y=w2138) -> (x+y=w2137:dbl)
            n1515 = Greater?(x=w2124, y=u32 999) -> (0:w2122:bool)
            n1516 = Greater?(x=w2128, y=w2126) -> (0:w2125:bool)
            n1517 = Greater?(x=w2136, y=w2132) -> (0:w2131:bool)
            n1518 = Greater?(x=w2140, y=w2137) -> (0:w2120:bool)
            n1519 = local write "miss trial"(w2131) -> ()
            n1520 = And(x=w2125, y=w2122) -> (x .and. y?=w2121:bool)
            n1521 = Or(x=w2120, y=w2121) -> (x .or. y?=w2119:bool)
          }
        }
      }
      frame True {
        n1522 = local read "VR Mode"() -> (w2141:bool)
        n1523 = case shown="True" w2141 {
          tunnel: [w2152 w2171] -> w2143
          tunnel: [w2153 w2163] -> w2142
          frame False {
            n1524 = local read "Hybrid licking"() -> (w2144:bool)
            n1525 = local read "Distance (cm)"() -> (w2148:dbl)
            n1526 = local read "prev. diode position"() -> (w2151:dbl)
            n1527 = Subtract(x=w2148, y=w2151) -> (x-y=w2146:dbl)
            n1528 = case shown="True" w2144 {
              tunnel: w2146 -> [_ w2159]
              tunnel: [FALSE w2155] -> w2145
              frame False {
              }
              frame True {
                n1529 = local read "Reward given"() -> (w2161:bool)
                n1530 = Less Or Equal?(x=w2159, y=15.0) -> (x <= y?=w2156:bool)
                n1531 = Greater Or Equal?(x=w2159, y=4.0) -> (x >= y?=w2157:bool)
                n1532 = Not(x=w2161) -> (.not. x?=w2158:bool)
                n1533 = Compound Arithmetic op=AND(w2156, w2157, w2158) -> (w2155:bool)
                n1534 = local write "miss trial"(w2155) -> ()
              }
            }
            n1535 = Less?(x=w2146, y=4.0) -> (x < y?=w2147:bool)
            n1536 = Greater?(x=w2146, y=30.0) -> (0:w2153:bool)
            n1537 = Or(x=w2147, y=w2145) -> (x .or. y?=w2152:bool)
          }
          frame True {
            n1538 = local read "Hybrid licking"() -> (w2168:bool)
            n1539 = local read "Unity position:"() -> (w2166:sgl)
            n1540 = case shown="True" w2168 {
              tunnel: [FALSE w2176] -> w2169
              frame False {
              }
              frame True {
                n1541 = local read "Reward given"() -> (w2180:bool)
                n1542 = local read "Unity position:"() -> (w2181:sgl)
                n1543 = Not(x=w2180) -> (.not. x?=w2179:bool)
                n1544 = Less?(x=w2181, y=sgl -10.0) -> (x < y?=w2178:bool)
                n1545 = Compound Arithmetic op=AND(w2178, w2179) -> (w2176:bool)
                n1546 = local write "miss trial"(w2176) -> ()
              }
            }
            n1547 = local read "reward zone start"() -> (w2173:dbl)
            n1548 = local read "Unity position:"() -> (w2174:sgl)
            n1549 = Greater Or Equal?(x=w2174, y=w2173) -> (x >= y?=w2170:bool)
            n1550 = Less?(x=w2166, y=10.0) -> (x < y?=w2164:bool)
            n1551 = Greater?(x=w2166, y=sgl 0.0) -> (0:w2167:bool)
            n1552 = Compound Arithmetic op=OR(w2170, w2169) -> (w2171:bool)
            n1553 = And(x=w2164, y=w2167) -> (x .and. y?=w2163:bool)
          }
        }
        "Within Reward zone" <- w2143
      }
    }
    n1554 = case shown="True" "Give reward" {
      tunnel: w2070 -> [_ w2185]
      tunnel: w2082 -> [_ w2184]
      frame False {
      }
      frame True {
        n1555 = flat-sequence {
          tunnel: w2185 -> [w2191]
          tunnel: w2184 -> [w2186]
          frame #0 {
            n1556 = local read "Water cnt. reset"() -> (w2189:i32)
            n1557 = for {
              N: w2186 -> [_]
              tunnel: w2191 -> [w2193]
              n1558 = local read "Valve open dur. (ms)"() -> (w2192:u32)
              n1559 = local write "Valve open"(TRUE ("Valve open")) -> ()
              n1560 = call "SendTriggerPulse.vi"("Trigger Duration (ms)"=w2192, "Refnum in"=w2193) -> ()  [unwired: 9 in, 1 out]
            }
            n1561 = local read "Water count"() -> (w2187:i32)
            n1562 = Add(x=w2186, y=w2189) -> (x+y=w2190:i32)
            n1563 = Add(x=w2186, y=w2187) -> (x+y=w2188:i32)
            n1564 = local write "Water cnt. reset"(w2190) -> ()
            n1565 = local write "Water count"(w2188) -> ()
          }
          frame #1 {
            n1566 = local write "Valve open"(FALSE ("Valve open")) -> ()
          }
        }
      }
    }
    n1567 = case shown="True" w2085 {
      tunnel: w2080 -> [_ w2208]
      tunnel: w2070 -> [_ w2206]
      tunnel: [w2197 w2199] -> w2062
      tunnel: w2061 -> [w2197 w2198]
      frame False {
      }
      frame True {
        n1568 = local read "Active licking"() -> (w2204:bool)
        n1569 = local read "miss trial"() -> (w2202:bool)
        n1570 = local read "Reward given"() -> (w2205:bool)
        n1571 = case shown="False" w2204 {
          tunnel: [TRUE w2212] -> w2200
          frame False {
          }
          frame True {
            n1572 = local read "Lick indicator"() -> (w2211:dbl)
            n1573 = Greater?(x=w2211, y=0.1) -> (0:w2212:bool)
          }
        }
        n1574 = Not(x=w2205) -> (.not. x?=w2203:bool)
        n1575 = Compound Arithmetic op=OR(w2200, w2202) -> (w2201:bool)
        n1576 = Compound Arithmetic op=AND(w2201, w2203) -> (w2207:bool)
        n1577 = case shown="True" w2207 {
          tunnel: w2208 -> [_ w2218]
          tunnel: w2206 -> [_ w2217]
          tunnel: [w2213 w2214] -> w2199
          tunnel: w2198 -> [w2213 _]
          frame False {
          }
          frame True {
            n1578 = flat-sequence {
              tunnel: w2218 -> [w2223]
              tunnel: w2217 -> [w2222]
              tunnel: [w2222] -> w2216
              tunnel: [w2219] -> w2215
              tunnel: w2216 -> [w2236]
              tunnel: w2215 -> [w2229]
              tunnel: [w2228] -> w2214
              frame #0 {
                n1579 = local read "miss trial"() -> (w2220:bool)
                n1580 = case shown="False" w2220 {
                  tunnel: w2223 -> [_ w2227]
                  tunnel: [1 ("Repetition") w2225] -> w2219
                  frame True {
                  }
                  frame False {
                    n1581 = local read "Sound duration (ms)"() -> (w2226:u32)
                    n1582 = local read "Repetition"() -> (w2225:i32)
                    n1583 = call "SendTriggerPulse.vi"("Trigger Duration (ms)"=w2226, "Refnum in"=w2227) -> ()  [unwired: 9 in, 1 out]
                  }
                }
                n1584 = Not(x=w2220) -> (.not. x?=w2221:bool)
                n1585 = local write "hit trial"(w2221) -> ()
              }
              frame #1 {
                n1586 = Random Number (0-1)() -> (number: 0 to 1=w2230:dbl)
                n1587 = local read "Water cnt. reset"() -> (w2234:i32)
                n1588 = local write "Reward given"(TRUE ("Reward given")) -> ()
                n1589 = local read "Water count"() -> (w2231:i32)
                n1590 = local write "random rew"(w2230) -> ()
                n1591 = Add(x=w2229, y=w2234) -> (x+y=w2233:i32)
                n1592 = Add(x=w2229, y=w2231) -> (x+y=w2232:i32)
                n1593 = for {
                  N: w2229 -> [_]
                  tunnel: w2236 -> [w2237]
                  n1594 = stacked-sequence {
                    tunnel: w2237 -> [w2240 _]
                    frame #0 {
                      n1595 = local read "Valve open dur. (ms)"() -> (w2238:u32)
                      n1596 = local write "Valve open"(TRUE ("Valve open")) -> ()
                      n1597 = call "SendTriggerPulse.vi"("Trigger Duration (ms)"=w2238, "Refnum in"=w2240) -> ()  [unwired: 9 in, 1 out]
                      n1598 = Wait (ms)(milliseconds to wait=w2238) -> ()  [unwired: 1 out]
                    }
                    frame #1 {
                      n1599 = local read "Distance (cm)"() -> (w2241:dbl)
                      n1600 = local write "Valve open"(FALSE ("Valve open")) -> ()
                      n1601 = local write "Prev. rew. pos."(w2241) -> ()
                      n1602 = Wait (ms)(milliseconds to wait=u32 50) -> ()  [unwired: 1 out]
                    }
                  }
                }
                n1603 = local write "Water count"(w2232) -> ()
                n1604 = local write "Water cnt. reset"(w2233) -> ()
                n1605 = Tick Count (ms)() -> (millisecond timer value=w2228:u32)
              }
            }
          }
        }
      }
    }
    n1606 = case shown="True" w2075 {
      frame False {
      }
      frame True {
        n1607 = local write "Reward given"(FALSE ("Reward given")) -> ()
      }
    }
    n1608 = Tick Count (ms)() -> (millisecond timer value=w2072:u32)
    n1609 = local write "Active licking"("Active licking") -> ()
    n1610 = Subtract(x=w2072, y=w2071) -> (x-y=→"Reward read loop rate":u32)
    n1611 = local read "Lick indicator"() -> (w2078:dbl)
    n1612 = call "Is Value Changed.vim"("value"="Open valve") -> ("changed or first call?"=w2064:bool)
    n1613 = case shown="True" w2064 {
      tunnel: w2070 -> [_ w2092]
      tunnel: "Open valve" -> [_ w2091]
      frame False {
      }
      frame True {
        n1614 = call <vilib>:"DAQmx Start Task.vi"("task/channels in"=w2092) -> ("task out"=w2094:refnum<k21>)  [unwired: 13 in, 1 out]
        n1615 = call-poly <vilib>:"DAQmx Write.vi"("task/channels in"=w2094, "data"=w2091) -> ("task out"=w2093:refnum<k21>)  [unwired: 11 in, 2 out]
        n1616 = call <vilib>:"DAQmx Stop Task.vi"("task/channels in"=w2093) -> ()  [unwired: 13 in, 2 out]
      }
    }
    n1617 = Greater?(x=w2078, y=i8 0) -> (0:→"Lick":bool)
    n1618 = case shown="True" "Hybrid licking" {
      frame False {
      }
      frame True {
        n1619 = local write "Active licking"(TRUE ("Active licking")) -> ()
      }
    }
    n1620 = local read "Valve open"() -> (→"Valve open":bool)
    n1621 = case shown="False" "Boolean" {
      tunnel: [w2089 w2090] -> w2067
      frame False {
        n1622 = local read "Water cnt. reset"() -> (w2089:i32)
      }
      frame True {
        n1623 = local read "Water count"() -> (w2090:i32)
      }
    }
    n1624 = local read "Reward size (ul)"() -> (w2069:dbl)
    n1625 = case shown="True" "Reset water count" {
      frame False {
      }
      frame True {
        n1626 = local write "Water cnt. reset"(0 ("Waret received")) -> ()
        n1627 = local write "Reset water count"(FALSE ("Reset water count")) -> ()
      }
    }
    n1628 = local read "Exit"() -> (w2087:bool)
    n1629 = Multiply(x=w2067, y=w2069) -> (x*y=→"Water received (ul)":dbl)
    n1630 = Wait (ms)(milliseconds to wait=u32 5) -> ()  [unwired: 1 out]
  }
  n1631 = case shown="True" w76 {
    frame False {
    }
    frame True {
      n1632 = local read "settings folder"() -> (w2246:path)
      n1633 = Build Path(base path=w2246, name or relative path="Laser stimulus calibration.txt") -> (appended path=w2244:path)
      n1634 = Open/Create/Replace File(file path (use dialog)=w2244, operation (0:open)=T11."open", access (0:read/write)=enum16{"read/write", "read-only", "write-only"}."read-only") -> (refnum out=w2259:refnum<file>)  [unwired: 3 in, 2 out]
      n1635 = Read from Text File(file (use dialog)=w2259) -> (refnum out=w2258:refnum<file>, text=w2260:string)  [unwired: 3 in, 2 out]
      "Laser stimulus calibration" <- w2260
      n1636 = Match Pattern(string=w2260, regular expression="Max output: ") -> (after substring=w2261:string)  [unwired: 1 in, 3 out]
      n1637 = Match Pattern(string=w2260, regular expression="Min output: ") -> (after substring=w2257:string)  [unwired: 1 in, 3 out]
      n1638 = Close File(refnum=w2258) -> ()  [unwired: 1 in, 2 out]
      n1639 = Match Pattern(string=w2261, regular expression=" V") -> (before substring=w2263:string)  [unwired: 1 in, 3 out]
      n1640 = Match Pattern(string=w2257, regular expression=" V") -> (before substring=w2262:string)  [unwired: 1 in, 3 out]
      n1641 = Fract/Exp String To Number(string=w2262) -> (number=w2250:dbl)  [unwired: 3 in, 1 out]
      n1642 = Fract/Exp String To Number(string=w2263) -> (number=w2249:dbl)  [unwired: 3 in, 1 out]
      n1643 = while {
        shift-right: [w2268] -> w2248
        shift-left: _ -> [w2270]
        shift-right: [w2267] -> w2247
        shift-left: _ -> [w2269]
        shift-right: [w2265] -> _
        shift-left: _ -> [w2264]
        stop <- w2266 stop-if-true
        n1644 = case shown="\"20 Hz full trial\"" w2264 {
          selector: w2264 -> [_ w2345 w2379 w2438 w2499 w2527 w2599 w2664]
          tunnel: w2270 -> [w2273 w2350 w2383 w2448 w2509 w2525 w2597 w2675]
          tunnel: w2269 -> [w2271 w2349 w2382 w2447 w2508 w2524 w2596 w2674]
          tunnel: [w2274 w2348 w2381 w2444 w2505 w2523 w2595 w2671] -> w2268
          tunnel: [w2272 w2347 w2380 w2443 w2504 w2522 w2594 w2670] -> w2267
          tunnel: [w2275 w2341 w2376 w2437 w2498 w2526 w2598 w2665] -> w2265
          frame "None", Default {
            n1645 = local read "Primary masking light"() -> (w2275:T3)
            n1646 = case shown="\"Continuous specified light off trials\"" w2275 {
              tunnel: [w2278 w2280 w2293 w2306 w2319 w2332 w2335 w2338] -> w2274
              tunnel: w2273 -> [w2278 w2282 w2295 w2308 w2321 _ _ _]
              tunnel: [w2277 w2279 w2292 w2305 w2318 w2331 w2334 w2337] -> w2272
              tunnel: w2271 -> [w2277 w2281 w2294 w2307 w2320 _ _ _]
              frame "None", Default {
              }
              frame "20 Hz until reward " {
                w2286 = 10123 items=["Finite Samples"=10178, "Continuous Samples"=10123, "Hardware Timed Single Point"=12522]  # Sample Mode
                n1647 = call <vilib>:"DAQmx Clear Task.vi"("task in"=w2282, "error in"=w2281) -> ()  [unwired: 13 in, 1 out]
                n1648 = call-poly <vilib>:"DAQmx Create Virtual Channel.vi"("frequency"=20.0, "duty cycle"=0.5 ("Duty Cycle"), "counter"=tag "Dev1/ctr3" ("Counter")) -> ("task out"=w2291:refnum<k21>, "error out"=w2290:errorcluster)  [unwired: 11 in]
                n1649 = property class="DAQmx Channel"(reference=w2291, error in=w2290, "CO.Pulse.Term"=tag "/Dev1/PFI15" ("Output Terminal")) -> (reference out=w2288:refnum<k21>, error out=w2289:errorcluster)
                n1650 = call-poly <vilib>:"DAQmx Timing.vi"("task/channels in"=w2288, "sample mode"=w2286, "error in"=w2289) -> ("task out"=w2280:refnum<k21>, "error out"=w2279:errorcluster)  [unwired: 11 in]
              }
              frame "20 Hz specified light off trials" {
                w2299 = 10123 items=["Finite Samples"=10178, "Continuous Samples"=10123, "Hardware Timed Single Point"=12522]  # Sample Mode
                n1651 = call <vilib>:"DAQmx Clear Task.vi"("task in"=w2295, "error in"=w2294) -> ()  [unwired: 13 in, 1 out]
                n1652 = call-poly <vilib>:"DAQmx Create Virtual Channel.vi"("frequency"=20.0, "duty cycle"=0.5 ("Duty Cycle"), "counter"=tag "Dev1/ctr3" ("Counter")) -> ("task out"=w2304:refnum<k21>, "error out"=w2303:errorcluster)  [unwired: 11 in]
                n1653 = property class="DAQmx Channel"(reference=w2304, error in=w2303, "CO.Pulse.Term"=tag "/Dev1/PFI15" ("Output Terminal")) -> (reference out=w2301:refnum<k21>, error out=w2302:errorcluster)
                n1654 = call-poly <vilib>:"DAQmx Timing.vi"("task/channels in"=w2301, "sample mode"=w2299, "error in"=w2302) -> ("task out"=w2293:refnum<k21>, "error out"=w2292:errorcluster)  [unwired: 11 in]
              }
              frame "20 Hz specified all trials" {
                w2312 = 10123 items=["Finite Samples"=10178, "Continuous Samples"=10123, "Hardware Timed Single Point"=12522]  # Sample Mode
                n1655 = call <vilib>:"DAQmx Clear Task.vi"("task in"=w2308, "error in"=w2307) -> ()  [unwired: 13 in, 1 out]
                n1656 = call-poly <vilib>:"DAQmx Create Virtual Channel.vi"("frequency"=20.0, "duty cycle"=0.5 ("Duty Cycle"), "counter"=tag "Dev1/ctr3" ("Counter")) -> ("task out"=w2317:refnum<k21>, "error out"=w2316:errorcluster)  [unwired: 11 in]
                n1657 = property class="DAQmx Channel"(reference=w2317, error in=w2316, "CO.Pulse.Term"=tag "/Dev1/PFI15" ("Output Terminal")) -> (reference out=w2314:refnum<k21>, error out=w2315:errorcluster)
                n1658 = call-poly <vilib>:"DAQmx Timing.vi"("task/channels in"=w2314, "sample mode"=w2312, "error in"=w2315) -> ("task out"=w2306:refnum<k21>, "error out"=w2305:errorcluster)  [unwired: 11 in]
              }
              frame "20 Hz full trial" {
                w2325 = 10123 items=["Finite Samples"=10178, "Continuous Samples"=10123, "Hardware Timed Single Point"=12522]  # Sample Mode
                n1659 = call <vilib>:"DAQmx Clear Task.vi"("task in"=w2321, "error in"=w2320) -> ()  [unwired: 13 in, 1 out]
                n1660 = call-poly <vilib>:"DAQmx Create Virtual Channel.vi"("frequency"=20.0, "duty cycle"=0.5 ("Duty Cycle"), "counter"=tag "Dev1/ctr3" ("Counter")) -> ("task out"=w2330:refnum<k21>, "error out"=w2329:errorcluster)  [unwired: 11 in]
                n1661 = property class="DAQmx Channel"(reference=w2330, error in=w2329, "CO.Pulse.Term"=tag "/Dev1/PFI15" ("Output Terminal")) -> (reference out=w2327:refnum<k21>, error out=w2328:errorcluster)
                n1662 = call-poly <vilib>:"DAQmx Timing.vi"("task/channels in"=w2327, "sample mode"=w2325, "error in"=w2328) -> ("task out"=w2319:refnum<k21>, "error out"=w2318:errorcluster)  [unwired: 11 in]
              }
              frame "Continuous specified light off trials" {
                n1663 = call-poly <vilib>:"DAQmx Create Virtual Channel.vi"("lines"=tag "Dev1/port2/line7") -> ("task out"=w2332:refnum<k21>, "error out"=w2331:errorcluster)  [unwired: 13 in]
              }
              frame "Continuous specified all trials" {
                n1664 = call-poly <vilib>:"DAQmx Create Virtual Channel.vi"("lines"=tag "Dev1/port2/line7") -> ("task out"=w2335:refnum<k21>, "error out"=w2334:errorcluster)  [unwired: 13 in]
              }
              frame "Continuous full trial" {
                n1665 = call-poly <vilib>:"DAQmx Create Virtual Channel.vi"("lines"=tag "Dev1/port2/line7") -> ("task out"=w2338:refnum<k21>, "error out"=w2337:errorcluster)  [unwired: 13 in]
              }
            }
            n1666 = Wait (ms)(milliseconds to wait=u32 20) -> ()  [unwired: 1 out]
          }
          frame "20 Hz until reward " {
            n1667 = local read "Reward given"() -> (w2346:bool)
            n1668 = Not(x=w2346) -> (.not. x?=w2342:bool)
            n1669 = case shown="True" w2342 {
              tunnel: w2350 -> [w2353 w2359]
              tunnel: w2349 -> [w2352 w2361]
              tunnel: [w2353 w2354] -> w2348
              tunnel: [w2352 w2355] -> w2347
              frame False {
                n1670 = Wait (ms)(milliseconds to wait=u32 20) -> ()  [unwired: 1 out]
              }
              frame True {
                n1671 = call <vilib>:"DAQmx Start Task.vi"("task/channels in"=w2359, "error in"=w2361) -> ("task out"=w2358:refnum<k21>, "error out"=w2360:errorcluster)  [unwired: 12 in]
                n1672 = while {
                  tunnel: w2358 -> [w2373]
                  tunnel: w2360 -> [w2372]
                  tunnel: [w2370] -> w2356
                  tunnel: [w2371] -> w2357
                  stop <- w2368 stop-if-true
                  n1673 = local read "Primary masking light"() -> (w2363:T3)
                  n1674 = call <vilib>:"DAQmx Is Task Done.vi"("task/channels in"=w2373, "error in"=w2372) -> ("task out"=w2371:refnum<k21>, "error out"=w2370:errorcluster)  [unwired: 11 in, 1 out]
                  n1675 = local read "Reward given"() -> (w2367:bool)
                  n1676 = Unbundle By Name(w2370) -> ("status"=w2365:bool)
                  n1677 = local read "Exit"() -> (w2366:bool)
                  n1678 = Not Equal?(x=w2363, y=T14."20 Hz until reward ") -> (x != y?=w2364:bool)
                  n1679 = Wait (ms)(milliseconds to wait=u32 20) -> ()  [unwired: 1 out]
                  n1680 = Compound Arithmetic op=OR(w2365, w2366, w2367, w2364) -> (w2368:bool)
                }
                n1681 = call <vilib>:"DAQmx Stop Task.vi"("task/channels in"=w2357, "error in"=w2356) -> ("task out"=w2354:refnum<k21>, "error out"=w2355:errorcluster)  [unwired: 12 in]
              }
            }
            n1682 = local read "Primary masking light"() -> (w2343:T3)
            n1683 = Equal?(x=w2343, y=w2345) -> (x = y?=w2344:bool)
            n1684 = Select(t=w2343, s=w2344, f=T14."None") -> (s? t:f=w2341:T3)
          }
          frame "20 Hz full trial" {
            n1685 = local read "Run experiment"() -> (w2374:bool)
            n1686 = case shown="True" w2374 {
              tunnel: w2383 -> [w2386 w2392]
              tunnel: w2382 -> [w2385 w2394]
              tunnel: [w2386 w2387] -> w2381
              tunnel: [w2385 w2388] -> w2380
              frame False {
                n1687 = Wait (ms)(milliseconds to wait=u32 20) -> ()  [unwired: 1 out]
              }
              frame True {
                n1688 = call <vilib>:"DAQmx Start Task.vi"("task/channels in"=w2392, "error in"=w2394) -> ("task out"=w2391:refnum<k21>, "error out"=w2393:errorcluster)  [unwired: 12 in]
                n1689 = while {
                  tunnel: w2391 -> [w2403]
                  tunnel: w2393 -> [w2402]
                  tunnel: [w2413] -> w2389
                  tunnel: [w2414] -> w2390
                  stop <- w2411 stop-if-true
                  n1690 = local read "stim started"() -> (w2398:bool)
                  n1691 = Equal?(x=w2398, y=TRUE) -> (x = y?=w2396:bool)
                  n1692 = call "Is Value Changed.vim"("value"=w2398) -> ("changed or first call?"=w2397:bool)
                  n1693 = And(x=w2397, y=w2396) -> (x .and. y?=w2395:bool)
                  n1694 = case shown="True" w2395 {
                    tunnel: w2403 -> [w2416 w2423]
                    tunnel: w2402 -> [w2415 w2424]
                    tunnel: [w2416 w2418] -> w2401
                    tunnel: [w2415 w2417] -> w2400
                    frame False {
                    }
                    frame True {
                      n1695 = flat-sequence {
                        tunnel: w2424 -> [w2426]
                        tunnel: w2423 -> [w2425]
                        tunnel: [w2428] -> w2422
                        tunnel: [w2427] -> w2421
                        tunnel: w2422 -> [w2431]
                        tunnel: w2421 -> [w2430]
                        tunnel: [w2431] -> w2420
                        tunnel: [w2430] -> w2419
                        tunnel: w2420 -> [w2433]
                        tunnel: w2419 -> [w2432]
                        tunnel: [w2435] -> w2418
                        tunnel: [w2434] -> w2417
                        frame #0 {
                          n1696 = call <vilib>:"DAQmx Stop Task.vi"("task/channels in"=w2425, "error in"=w2426) -> ("task out"=w2428:refnum<k21>, "error out"=w2427:errorcluster)  [unwired: 12 in]
                        }
                        frame #1 {
                          n1697 = Wait (ms)(milliseconds to wait=u32 5) -> ()  [unwired: 1 out]
                        }
                        frame #2 {
                          n1698 = call <vilib>:"DAQmx Start Task.vi"("task/channels in"=w2433, "error in"=w2432) -> ("task out"=w2435:refnum<k21>, "error out"=w2434:errorcluster)  [unwired: 12 in]
                        }
                      }
                    }
                  }
                  n1699 = local read "Primary masking light"() -> (w2407:T3)
                  n1700 = local read "Run experiment"() -> (w2406:bool)
                  n1701 = call <vilib>:"DAQmx Is Task Done.vi"("task/channels in"=w2401, "error in"=w2400) -> ("task out"=w2414:refnum<k21>, "error out"=w2413:errorcluster)  [unwired: 11 in, 1 out]
                  n1702 = local read "Exit"() -> (w2410:bool)
                  n1703 = Unbundle By Name(w2413) -> ("status"=w2409:bool)
                  n1704 = Not(x=w2406) -> (.not. x?=w2405:bool)
                  n1705 = Not Equal?(x=w2407, y=T3."20 Hz full trial") -> (x != y?=w2408:bool)
                  n1706 = Wait (ms)(milliseconds to wait=u32 2) -> ()  [unwired: 1 out]
                  n1707 = Compound Arithmetic op=OR(w2409, w2410, w2405, w2408) -> (w2411:bool)
                }
                n1708 = call <vilib>:"DAQmx Stop Task.vi"("task/channels in"=w2390, "error in"=w2389) -> ("task out"=w2387:refnum<k21>, "error out"=w2388:errorcluster)  [unwired: 12 in]
              }
            }
            n1709 = local read "Primary masking light"() -> (w2377:T3)
            n1710 = Equal?(x=w2377, y=w2379) -> (x = y?=w2378:bool)
            n1711 = Select(t=w2377, s=w2378, f=T14."None") -> (s? t:f=w2376:T3)
          }
          frame "Continuous specified light off trials" {
            n1712 = call <vilib>:"DAQmx Start Task.vi"("task/channels in"=w2448, "error in"=w2447) -> ("task out"=w2446:refnum<k21>, "error out"=w2445:errorcluster)  [unwired: 12 in]
            n1713 = disable-structure shown="Disabled" {
              disable-tunnel: w2446 -> [w2452 _]
              disable-tunnel: w2445 -> [w2451 _]
              disable-tunnel: [w2450 _] -> w2442
              disable-tunnel: [w2449 _] -> w2441
              frame Disabled {
                n1714 = while {
                  tunnel: w2452 -> [w2465]
                  tunnel: w2451 -> [w2464]
                  tunnel: [w2463] -> w2449
                  tunnel: [w2462] -> w2450
                  stop <- w2457 stop-if-true
                  n1715 = local read "VR Mode"() -> (w2459:bool)
                  n1716 = case shown="True" w2459 {
                    tunnel: [w2468 w2486] -> w2460
                    frame False {
                      n1717 = local read "prev. diode position"() -> (w2466:dbl)
                      n1718 = local read "total distance cm"() -> (w2477:sgl[])
                      n1719 = local read "total distance cm"() -> (w2478:sgl[])
                      n1720 = local read "prev. diode position"() -> (w2467:dbl)
                      n1721 = local read item#-1() -> ()  [unwired: 1 out]
                      n1722 = local read item#-1() -> ()  [unwired: 1 out]
                      n1723 = Subtract() -> (x-y=w2473:dbl)  [unwired: 2 in]
                      n1724 = Divide(x=w2473, y=2.0) -> (x/y=w2471:dbl)
                      n1725 = Absolute Value(x=w2471) -> (abs(x)=w2470:dbl)
                      n1726 = Add(y=w2470) -> (x+y=w2469:dbl)  [unwired: 1 in]
                      n1727 = Array Max & Min(array=w2477) -> (max value=w2476:sgl)  [unwired: 3 out]
                      n1728 = Array Max & Min(array=w2478) -> (max value=w2479:sgl)  [unwired: 3 out]
                      n1729 = Subtract(x=w2476, y=w2466) -> (x-y=w2475:dbl)
                      n1730 = Subtract(x=w2479, y=w2467) -> (x-y=w2480:dbl)
                      n1731 = Greater?(x=w2475) -> (0:w2474:bool)  [unwired: 1 in]
                      n1732 = case shown="True" w2474 {
                        frame False {
                        }
                        frame True {
                          n1733 = local write "Masking light 2"(FALSE ("Masking light")) -> ()
                        }
                      }
                      n1734 = Greater?(x=w2480) -> (0:w2482:bool)  [unwired: 1 in]
                      n1735 = Less?(x=w2480, y=w2469) -> (x < y?=w2481:bool)
                      n1736 = And(x=w2481, y=w2482) -> (x .and. y?=w2468:bool)
                    }
                    frame True {
                      n1737 = local read "Unity position:"() -> (w2491:sgl)
                      n1738 = local read "Unity position:"() -> (w2492:sgl)
                      n1739 = local read "Unity position:"() -> (w2488:sgl)
                      n1740 = local read item#-1() -> ()  [unwired: 1 out]
                      n1741 = local read item#-1() -> ()  [unwired: 1 out]
                      n1742 = local read item#-1() -> ()  [unwired: 1 out]
                      n1743 = Add(y=15.0) -> (x+y=w2484:dbl)  [unwired: 1 in]
                      n1744 = Less?(x=w2492, y=w2484) -> (x < y?=w2489:bool)
                      n1745 = Greater?(x=w2488) -> (0:w2487:bool)  [unwired: 1 in]
                      n1746 = Greater?(x=w2491) -> (0:w2490:bool)  [unwired: 1 in]
                      n1747 = case shown="True" w2490 {
                        frame False {
                        }
                        frame True {
                          n1748 = local write "Masking light 2"(FALSE ("Masking light")) -> ()
                        }
                      }
                      n1749 = And(x=w2489, y=w2487) -> (x .and. y?=w2486:bool)
                    }
                  }
                  n1750 = Wait (ms)(milliseconds to wait=u32 10) -> ()  [unwired: 1 out]
                  n1751 = local read "Primary masking light"() -> (w2455:T3)
                  n1752 = case shown="True" w2460 {
                    frame False {
                    }
                    frame True {
                      n1753 = local read "Light ON"() -> (w2495:bool)
                      n1754 = Not(x=w2495) -> (.not. x?=w2494:bool)
                      n1755 = case shown="True" w2494 {
                        frame False {
                        }
                        frame True {
                          n1756 = local write "Masking light 2"(TRUE ("Masking light")) -> ()
                        }
                      }
                    }
                  }
                  n1757 = local read "Masking light 2"() -> (w2458:bool)
                  n1758 = Not Equal?(x=w2455, y=T14."Continuous specified light off trials") -> (x != y?=w2454:bool)
                  n1759 = local read "Exit"() -> (w2456:bool)
                  n1760 = call-poly <vilib>:"DAQmx Write.vi"("task/channels in"=w2465, "data"=w2458, "error in"=w2464) -> ("task out"=w2463:refnum<k21>, "error out"=w2462:errorcluster)  [unwired: 10 in, 1 out]
                  n1761 = Compound Arithmetic op=OR(w2454, w2456) -> (w2457:bool)
                }
              }
              frame Enabled {
              }
            }
            n1762 = local read "Primary masking light"() -> (w2439:T3)
            n1763 = Equal?(x=w2439, y=w2438) -> (x = y?=w2440:bool)
            n1764 = Select(t=w2439, s=w2440, f=T14."None") -> (s? t:f=w2437:T3)
            n1765 = call <vilib>:"DAQmx Stop Task.vi"("task/channels in"=w2441, "error in"=w2442) -> ("task out"=w2444:refnum<k21>, "error out"=w2443:errorcluster)  [unwired: 12 in]
          }
          frame "Continuous full trial" {
            n1766 = call <vilib>:"DAQmx Start Task.vi"("task/channels in"=w2509, "error in"=w2508) -> ("task out"=w2507:refnum<k21>, "error out"=w2506:errorcluster)  [unwired: 12 in]
            n1767 = while {
              tunnel: w2507 -> [w2520]
              tunnel: w2506 -> [w2519]
              tunnel: [w2518] -> w2502
              tunnel: [w2517] -> w2503
              stop <- w2515 stop-if-true
              n1768 = Wait (ms)(milliseconds to wait=u32 10) -> ()  [unwired: 1 out]
              n1769 = local read "Primary masking light"() -> (w2513:T3)
              n1770 = local read "Run experiment"() -> (w2511:bool)
              n1771 = Not Equal?(x=w2513, y=T3."Continuous full trial") -> (x != y?=w2512:bool)
              n1772 = local read "Exit"() -> (w2514:bool)
              n1773 = call-poly <vilib>:"DAQmx Write.vi"("task/channels in"=w2520, "data"=w2511, "error in"=w2519) -> ("task out"=w2518:refnum<k21>, "error out"=w2517:errorcluster)  [unwired: 10 in, 1 out]
              n1774 = Compound Arithmetic op=OR(w2512, w2514) -> (w2515:bool)
            }
            n1775 = local read "Primary masking light"() -> (w2500:T3)
            n1776 = Equal?(x=w2500, y=w2499) -> (x = y?=w2501:bool)
            n1777 = Select(t=w2500, s=w2501, f=T14."None") -> (s? t:f=w2498:T3)
            n1778 = call <vilib>:"DAQmx Stop Task.vi"("task/channels in"=w2502, "error in"=w2503) -> ("task out"=w2505:refnum<k21>, "error out"=w2504:errorcluster)  [unwired: 12 in]
          }
          frame "20 Hz specified light off trials" {
            n1779 = disable-structure shown="Disabled" {
              disable-tunnel: w2525 -> [w2534 _]
              disable-tunnel: w2524 -> [w2533 _]
              disable-tunnel: [w2532 _] -> w2523
              disable-tunnel: [w2531 _] -> w2522
              frame Disabled {
                n1780 = local read "VR Mode"() -> (w2535:bool)
                n1781 = case shown="False" w2535 {
                  tunnel: [w2537 w2551] -> w2536
                  frame False {
                    n1782 = local read "total distance cm"() -> (w2543:sgl[])
                    n1783 = local read "prev. diode position"() -> (w2544:dbl)
                    n1784 = local read item#-1() -> ()  [unwired: 1 out]
                    n1785 = Subtract() -> (x-y=w2542:dbl)  [unwired: 2 in]
                    n1786 = Divide(x=w2542, y=2.0) -> (x/y=w2540:dbl)
                    n1787 = Absolute Value(x=w2540) -> (abs(x)=w2539:dbl)
                    n1788 = local read item#-1() -> ()  [unwired: 1 out]
                    n1789 = Add(y=w2539) -> (x+y=w2538:dbl)  [unwired: 1 in]
                    n1790 = Array Max & Min(array=w2543) -> (max value=w2545:sgl)  [unwired: 3 out]
                    n1791 = Subtract(x=w2545, y=w2544) -> (x-y=w2546:dbl)
                    n1792 = Greater?(x=w2546) -> (0:w2548:bool)  [unwired: 1 in]
                    n1793 = Less?(x=w2546, y=w2538) -> (x < y?=w2547:bool)
                    n1794 = And(x=w2547, y=w2548) -> (x .and. y?=w2537:bool)
                  }
                  frame True {
                    n1795 = local read "Unity position:"() -> (w2555:sgl)
                    n1796 = local read "Unity position:"() -> (w2553:sgl)
                    n1797 = local read item#-1() -> ()  [unwired: 1 out]
                    n1798 = local read item#-1() -> ()  [unwired: 1 out]
                    n1799 = Add(y=15.0) -> (x+y=w2549:dbl)  [unwired: 1 in]
                    n1800 = Less?(x=w2555, y=w2549) -> (x < y?=w2554:bool)
                    n1801 = Greater?(x=w2553) -> (0:w2552:bool)  [unwired: 1 in]
                    n1802 = And(x=w2554, y=w2552) -> (x .and. y?=w2551:bool)
                  }
                }
                n1803 = case shown="True" w2536 {
                  frame False {
                  }
                  frame True {
                    n1804 = local read "Light ON"() -> (w2557:bool)
                    n1805 = Not(x=w2557) -> (.not. x?=w2556:bool)
                    n1806 = case shown="True" w2556 {
                      frame False {
                      }
                      frame True {
                        n1807 = local write "Masking light 2"(TRUE ("Masking light")) -> ()
                      }
                    }
                  }
                }
                n1808 = local read "Masking light 2"() -> (w2530:bool)
                n1809 = case shown="True" w2530 {
                  tunnel: w2534 -> [w2561 w2567]
                  tunnel: w2533 -> [w2560 w2569]
                  tunnel: [w2561 w2562] -> w2532
                  tunnel: [w2560 w2563] -> w2531
                  frame False {
                    n1810 = Wait (ms)(milliseconds to wait=u32 20) -> ()  [unwired: 1 out]
                  }
                  frame True {
                    n1811 = call <vilib>:"DAQmx Start Task.vi"("task/channels in"=w2567, "error in"=w2569) -> ("task out"=w2566:refnum<k21>, "error out"=w2568:errorcluster)  [unwired: 12 in]
                    n1812 = while {
                      tunnel: w2566 -> [w2583]
                      tunnel: w2568 -> [w2582]
                      tunnel: [w2580] -> w2564
                      tunnel: [w2581] -> w2565
                      stop <- w2578 stop-if-true
                      n1813 = local read "VR Mode"() -> (w2570:bool)
                      n1814 = case shown="False" w2570 {
                        frame False {
                          n1815 = local read "prev. diode position"() -> (w2584:dbl)
                          n1816 = local read "total distance cm"() -> (w2588:sgl[])
                          n1817 = local read item#-1() -> ()  [unwired: 1 out]
                          n1818 = Array Max & Min(array=w2588) -> (max value=w2587:sgl)  [unwired: 3 out]
                          n1819 = Subtract(x=w2587, y=w2584) -> (x-y=w2586:dbl)
                          n1820 = Greater?(x=w2586) -> (0:w2585:bool)  [unwired: 1 in]
                          n1821 = case shown="True" w2585 {
                            frame False {
                            }
                            frame True {
                              n1822 = local write "Masking light 2"(FALSE ("Masking light")) -> ()
                            }
                          }
                        }
                        frame True {
                          n1823 = local read "Unity position:"() -> (w2591:sgl)
                          n1824 = local read item#-1() -> ()  [unwired: 1 out]
                          n1825 = Greater?(x=w2591) -> (0:w2590:bool)  [unwired: 1 in]
                          n1826 = case shown="True" w2590 {
                            frame False {
                            }
                            frame True {
                              n1827 = local write "Masking light 2"(FALSE ("Masking light")) -> ()
                            }
                          }
                        }
                      }
                      n1828 = local read "Primary masking light"() -> (w2574:T3)
                      n1829 = call <vilib>:"DAQmx Is Task Done.vi"("task/channels in"=w2583, "error in"=w2582) -> ("task out"=w2581:refnum<k21>, "error out"=w2580:errorcluster)  [unwired: 11 in, 1 out]
                      n1830 = local read "Masking light 2"() -> (w2572:bool)
                      n1831 = Unbundle By Name(w2580) -> ("status"=w2576:bool)
                      n1832 = local read "Exit"() -> (w2577:bool)
                      n1833 = Not(x=w2572) -> (.not. x?=w2571:bool)
                      n1834 = Not Equal?(x=w2574, y=T14."20 Hz specified light off trials") -> (x != y?=w2575:bool)
                      n1835 = Compound Arithmetic op=OR(w2576, w2577, w2571, w2575) -> (w2578:bool)
                      n1836 = Wait (ms)(milliseconds to wait=u32 20) -> ()  [unwired: 1 out]
                    }
                    n1837 = call <vilib>:"DAQmx Stop Task.vi"("task/channels in"=w2565, "error in"=w2564) -> ("task out"=w2562:refnum<k21>, "error out"=w2563:errorcluster)  [unwired: 12 in]
                  }
                }
              }
              frame Enabled {
              }
            }
            n1838 = local read "Primary masking light"() -> (w2528:T3)
            n1839 = Equal?(x=w2528, y=w2527) -> (x = y?=w2529:bool)
            n1840 = Select(t=w2528, s=w2529, f=T14."None") -> (s? t:f=w2526:T3)
          }
          frame "20 Hz specified all trials" {
            n1841 = disable-structure shown="Disabled" {
              disable-tunnel: w2597 -> [w2606 _]
              disable-tunnel: w2596 -> [w2605 _]
              disable-tunnel: [w2604 _] -> w2595
              disable-tunnel: [w2603 _] -> w2594
              frame Disabled {
                n1842 = local read "VR Mode"() -> (w2607:bool)
                n1843 = case shown="False" w2607 {
                  tunnel: [w2610 w2623] -> w2608
                  frame False {
                    n1844 = local read "total distance cm"() -> (w2616:sgl[])
                    n1845 = local read "prev. diode position"() -> (w2609:dbl)
                    n1846 = local read item#-1() -> ()  [unwired: 1 out]
                    n1847 = Subtract() -> (x-y=w2615:dbl)  [unwired: 2 in]
                    n1848 = Divide(x=w2615, y=2.0) -> (x/y=w2613:dbl)
                    n1849 = Absolute Value(x=w2613) -> (abs(x)=w2612:dbl)
                    n1850 = local read item#-1() -> ()  [unwired: 1 out]
                    n1851 = Add(y=w2612) -> (x+y=w2611:dbl)  [unwired: 1 in]
                    n1852 = Array Max & Min(array=w2616) -> (max value=w2617:sgl)  [unwired: 3 out]
                    n1853 = Subtract(x=w2617, y=w2609) -> (x-y=w2618:dbl)
                    n1854 = Greater?(x=w2618) -> (0:w2620:bool)  [unwired: 1 in]
                    n1855 = Less?(x=w2618, y=w2611) -> (x < y?=w2619:bool)
                    n1856 = And(x=w2619, y=w2620) -> (x .and. y?=w2610:bool)
                  }
                  frame True {
                    n1857 = local read "Unity position:"() -> (w2627:sgl)
                    n1858 = local read "Unity position:"() -> (w2625:sgl)
                    n1859 = local read item#-1() -> ()  [unwired: 1 out]
                    n1860 = local read item#-1() -> ()  [unwired: 1 out]
                    n1861 = Add(y=15.0) -> (x+y=w2621:dbl)  [unwired: 1 in]
                    n1862 = Less?(x=w2627, y=w2621) -> (x < y?=w2626:bool)
                    n1863 = Greater?(x=w2625) -> (0:w2624:bool)  [unwired: 1 in]
                    n1864 = And(x=w2626, y=w2624) -> (x .and. y?=w2623:bool)
                  }
                }
                n1865 = case shown="True" w2608 {
                  frame False {
                  }
                  frame True {
                    n1866 = local write "Masking light 2"(TRUE ("Masking light")) -> ()
                  }
                }
                n1867 = local read "Masking light 2"() -> (w2602:bool)
                n1868 = case shown="True" w2602 {
                  tunnel: w2606 -> [w2631 w2637]
                  tunnel: w2605 -> [w2630 w2639]
                  tunnel: [w2631 w2632] -> w2604
                  tunnel: [w2630 w2633] -> w2603
                  frame False {
                    n1869 = Wait (ms)(milliseconds to wait=u32 20) -> ()  [unwired: 1 out]
                  }
                  frame True {
                    n1870 = call <vilib>:"DAQmx Start Task.vi"("task/channels in"=w2637, "error in"=w2639) -> ("task out"=w2636:refnum<k21>, "error out"=w2638:errorcluster)  [unwired: 12 in]
                    n1871 = while {
                      tunnel: w2636 -> [w2653]
                      tunnel: w2638 -> [w2652]
                      tunnel: [w2650] -> w2634
                      tunnel: [w2651] -> w2635
                      stop <- w2648 stop-if-true
                      n1872 = local read "VR Mode"() -> (w2640:bool)
                      n1873 = case shown="False" w2640 {
                        frame False {
                          n1874 = local read "prev. diode position"() -> (w2654:dbl)
                          n1875 = local read "total distance cm"() -> (w2658:sgl[])
                          n1876 = local read item#-1() -> ()  [unwired: 1 out]
                          n1877 = Array Max & Min(array=w2658) -> (max value=w2657:sgl)  [unwired: 3 out]
                          n1878 = Subtract(x=w2657, y=w2654) -> (x-y=w2656:dbl)
                          n1879 = Greater?(x=w2656) -> (0:w2655:bool)  [unwired: 1 in]
                          n1880 = case shown="True" w2655 {
                            frame False {
                            }
                            frame True {
                              n1881 = local write "Masking light 2"(FALSE ("Masking light")) -> ()
                            }
                          }
                        }
                        frame True {
                          n1882 = local read "Unity position:"() -> (w2661:sgl)
                          n1883 = local read item#-1() -> ()  [unwired: 1 out]
                          n1884 = Greater?(x=w2661) -> (0:w2660:bool)  [unwired: 1 in]
                          n1885 = case shown="True" w2660 {
                            frame False {
                            }
                            frame True {
                              n1886 = local write "Masking light 2"(FALSE ("Masking light")) -> ()
                            }
                          }
                        }
                      }
                      n1887 = local read "Primary masking light"() -> (w2644:T3)
                      n1888 = call <vilib>:"DAQmx Is Task Done.vi"("task/channels in"=w2653, "error in"=w2652) -> ("task out"=w2651:refnum<k21>, "error out"=w2650:errorcluster)  [unwired: 11 in, 1 out]
                      n1889 = local read "Masking light 2"() -> (w2642:bool)
                      n1890 = Unbundle By Name(w2650) -> ("status"=w2646:bool)
                      n1891 = local read "Exit"() -> (w2647:bool)
                      n1892 = Not(x=w2642) -> (.not. x?=w2641:bool)
                      n1893 = Not Equal?(x=w2644, y=T14."20 Hz specified all trials") -> (x != y?=w2645:bool)
                      n1894 = Compound Arithmetic op=OR(w2646, w2647, w2641, w2645) -> (w2648:bool)
                      n1895 = Wait (ms)(milliseconds to wait=u32 20) -> ()  [unwired: 1 out]
                    }
                    n1896 = call <vilib>:"DAQmx Stop Task.vi"("task/channels in"=w2635, "error in"=w2634) -> ("task out"=w2632:refnum<k21>, "error out"=w2633:errorcluster)  [unwired: 12 in]
                  }
                }
              }
              frame Enabled {
              }
            }
            n1897 = local read "Primary masking light"() -> (w2600:T3)
            n1898 = Equal?(x=w2600, y=w2599) -> (x = y?=w2601:bool)
            n1899 = Select(t=w2600, s=w2601, f=T14."None") -> (s? t:f=w2598:T3)
          }
          frame "Continuous specified all trials" {
            n1900 = call <vilib>:"DAQmx Start Task.vi"("task/channels in"=w2675, "error in"=w2674) -> ("task out"=w2673:refnum<k21>, "error out"=w2672:errorcluster)  [unwired: 12 in]
            n1901 = disable-structure shown="Disabled" {
              disable-tunnel: w2673 -> [w2679 _]
              disable-tunnel: w2672 -> [w2678 _]
              disable-tunnel: [w2677 _] -> w2669
              disable-tunnel: [w2676 _] -> w2668
              frame Disabled {
                n1902 = while {
                  tunnel: w2679 -> [w2692]
                  tunnel: w2678 -> [w2691]
                  tunnel: [w2690] -> w2676
                  tunnel: [w2689] -> w2677
                  stop <- w2681 stop-if-true
                  n1903 = local read "VR Mode"() -> (w2686:bool)
                  n1904 = case shown="False" w2686 {
                    tunnel: [w2695 w2713] -> w2687
                    frame False {
                      n1905 = local read "prev. diode position"() -> (w2693:dbl)
                      n1906 = local read "total distance cm"() -> (w2704:sgl[])
                      n1907 = local read "total distance cm"() -> (w2705:sgl[])
                      n1908 = local read item#-1() -> ()  [unwired: 1 out]
                      n1909 = local read "prev. diode position"() -> (w2694:dbl)
                      n1910 = local read item#-1() -> ()  [unwired: 1 out]
                      n1911 = Subtract() -> (x-y=w2700:dbl)  [unwired: 2 in]
                      n1912 = Divide(x=w2700, y=2.0) -> (x/y=w2698:dbl)
                      n1913 = Absolute Value(x=w2698) -> (abs(x)=w2697:dbl)
                      n1914 = Add(y=w2697) -> (x+y=w2696:dbl)  [unwired: 1 in]
                      n1915 = Array Max & Min(array=w2704) -> (max value=w2703:sgl)  [unwired: 3 out]
                      n1916 = Array Max & Min(array=w2705) -> (max value=w2706:sgl)  [unwired: 3 out]
                      n1917 = Subtract(x=w2703, y=w2693) -> (x-y=w2702:dbl)
                      n1918 = Subtract(x=w2706, y=w2694) -> (x-y=w2707:dbl)
                      n1919 = Greater?(x=w2702) -> (0:w2701:bool)  [unwired: 1 in]
                      n1920 = case shown="True" w2701 {
                        frame False {
                        }
                        frame True {
                          n1921 = local write "Masking light 2"(FALSE ("Masking light")) -> ()
                        }
                      }
                      n1922 = Greater?(x=w2707) -> (0:w2709:bool)  [unwired: 1 in]
                      n1923 = Less?(x=w2707, y=w2696) -> (x < y?=w2708:bool)
                      n1924 = And(x=w2708, y=w2709) -> (x .and. y?=w2695:bool)
                    }
                    frame True {
                      n1925 = local read "Unity position:"() -> (w2718:sgl)
                      n1926 = local read "Unity position:"() -> (w2719:sgl)
                      n1927 = local read "Unity position:"() -> (w2715:sgl)
                      n1928 = local read item#-1() -> ()  [unwired: 1 out]
                      n1929 = local read item#-1() -> ()  [unwired: 1 out]
                      n1930 = local read item#-1() -> ()  [unwired: 1 out]
                      n1931 = Add(y=15.0) -> (x+y=w2711:dbl)  [unwired: 1 in]
                      n1932 = Less?(x=w2719, y=w2711) -> (x < y?=w2716:bool)
                      n1933 = Greater?(x=w2715) -> (0:w2714:bool)  [unwired: 1 in]
                      n1934 = Greater?(x=w2718) -> (0:w2717:bool)  [unwired: 1 in]
                      n1935 = case shown="True" w2717 {
                        frame False {
                        }
                        frame True {
                          n1936 = local write "Masking light 2"(FALSE ("Masking light")) -> ()
                        }
                      }
                      n1937 = And(x=w2716, y=w2714) -> (x .and. y?=w2713:bool)
                    }
                  }
                  n1938 = Wait (ms)(milliseconds to wait=u32 10) -> ()  [unwired: 1 out]
                  n1939 = local read "Primary masking light"() -> (w2683:T3)
                  n1940 = case shown="True" w2687 {
                    frame False {
                    }
                    frame True {
                      n1941 = local write "Masking light 2"(TRUE ("Masking light")) -> ()
                    }
                  }
                  n1942 = local read "Masking light 2"() -> (w2685:bool)
                  n1943 = Not Equal?(x=w2683, y=T14."Continuous specified all trials") -> (x != y?=w2682:bool)
                  n1944 = local read "Exit"() -> (w2684:bool)
                  n1945 = call-poly <vilib>:"DAQmx Write.vi"("task/channels in"=w2692, "data"=w2685, "error in"=w2691) -> ("task out"=w2690:refnum<k21>, "error out"=w2689:errorcluster)  [unwired: 10 in, 1 out]
                  n1946 = Compound Arithmetic op=OR(w2682, w2684) -> (w2681:bool)
                }
              }
              frame Enabled {
              }
            }
            n1947 = local read "Primary masking light"() -> (w2666:T3)
            n1948 = Equal?(x=w2666, y=w2664) -> (x = y?=w2667:bool)
            n1949 = Select(t=w2666, s=w2667, f=T14."None") -> (s? t:f=w2665:T3)
            n1950 = call <vilib>:"DAQmx Stop Task.vi"("task/channels in"=w2668, "error in"=w2669) -> ("task out"=w2671:refnum<k21>, "error out"=w2670:errorcluster)  [unwired: 12 in]
          }
        }
        n1951 = local read "Exit"() -> (w2266:bool)
      }
      n1952 = while {
        tunnel: w2249 -> [w2729]
        tunnel: w2250 -> [w2739]
        shift-right: [w2734] -> _
        shift-left: _ -> [w2733]
        shift-right: [w2725] -> _
        shift-left: _ -> [w2726]
        stop <- w2794 stop-if-true
        w2766 = "none" ("regular expression")
        w2744 = " %" ("regular expression")
        w2787 = "rew" ("regular expression")
        w2785 = "rew" ("regular expression")
        # "safety switch"
        # "Stop DAQ asistant first"
        n1953 = disable-structure shown="Disabled" {
          disable-tunnel: [w2795 _] -> w2769
          frame Disabled {
            w2803 = "rew" ("regular expression")
            w2805 = "rew" ("regular expression")
            w2811 = "none" ("regular expression")
            w2809 = "continuous" ("regular expression")
            n1954 = local read "Mask prot command"() -> (w2816:u16)
            n1955 = local read "protocol array"() -> (w2818:string[][])
            n1956 = Index Array(array=w2818, index (row)=w2816, index (col)=0 ("index (row)")) -> (element=w2813:string)
            n1957 = Index Array(array=w2818, index (row)=w2816, index (col)=1 ("disabled index (col)")) -> (element=w2804:string)
            n1958 = Index Array(array=w2818, index (row)=w2816, index (col)=2 ("disabled index (col)")) -> (element=w2799:string)
            n1959 = local read "Relative position"() -> (w2827:dbl)
            n1960 = Match Pattern(string=w2813, regular expression=w2809) -> (match substring=w2810:string)  [unwired: 1 in, 3 out]
            n1961 = Match Pattern(string=w2813, regular expression=" Hz") -> (before substring=w2814:string)  [unwired: 1 in, 3 out]
            n1962 = Match Pattern(string=w2813, regular expression=w2811) -> (match substring=w2812:string)  [unwired: 1 in, 3 out]
            n1963 = Match Pattern(string=w2804, regular expression="from ") -> (after substring=w2807:string)  [unwired: 1 in, 3 out]
            n1964 = Match Pattern(string=w2804, regular expression=w2805) -> (match substring=w2806:string)  [unwired: 1 in, 3 out]
            n1965 = Match Pattern(string=w2799, regular expression="to ") -> (after substring=w2801:string)  [unwired: 1 in, 3 out]
            n1966 = Match Pattern(string=w2799, regular expression=w2803) -> (match substring=w2802:string)  [unwired: 1 in, 3 out]
            n1967 = Equal?(x=w2810, y=w2809) -> (x = y?=w2822:bool)
            n1968 = Equal?(x=w2812, y=w2811) -> (x = y?=w2823:bool)
            n1969 = Equal?(x=w2806, y=w2805) -> (x = y?=w2825:bool)
            n1970 = Equal?(x=w2802, y=w2803) -> (x = y?=w2828:bool)
            n1971 = Decimal String To Number(string=w2814) -> (number=w2820:i32)  [unwired: 2 in, 1 out]
            n1972 = Decimal String To Number(string=w2807) -> (number=w2824:i32)  [unwired: 2 in, 1 out]
            n1973 = Decimal String To Number(string=w2801) -> (number=w2826:i32)  [unwired: 2 in, 1 out]
            n1974 = case shown="False" w2823 {
              tunnel: w2824 -> [w2834 _]
              tunnel: w2825 -> [w2833 _]
              tunnel: w2827 -> [w2832 _]
              tunnel: w2826 -> [w2831 _]
              tunnel: w2827 -> [w2830 _]
              tunnel: w2828 -> [w2829 _]
              frame False {
                n1975 = case shown="False" w2833 {
                  tunnel: w2834 -> [w2852 _]
                  tunnel: w2832 -> [w2847 _]
                  frame False {
                    n1976 = Greater Or Equal?(x=w2847, y=w2852) -> (x >= y?=w2845:bool)
                    n1977 = call "Is Value Changed.vim"("value"=w2845) -> ("changed or first call?"=w2848:bool)
                    n1978 = call "Is New Trial.vi"("Position data"=w2847) -> ("Boolean"=w2850:bool)  [unwired: 1 in]
                    n1979 = Compound Arithmetic op=OR(w2848, w2850) -> (w2849:bool)
                    n1980 = Not(x=w2845) -> (.not. x?=w2846:bool)
                    n1981 = And(x=w2845, y=w2849) -> (x .and. y?=w2851:bool)
                    n1982 = case shown="True" w2851 {
                      frame False {
                      }
                      frame True {
                        n1983 = local write "Start mask stim"(TRUE ("Start light stim")) -> ()
                        n1984 = local write "Stop mask stim"(FALSE ("Stop light stim")) -> ()
                      }
                    }
                    n1985 = case shown="True" w2846 {
                      frame False {
                      }
                      frame True {
                        n1986 = local write "Stop mask stim"(TRUE ("Stop light stim")) -> ()
                      }
                    }
                  }
                  frame True {
                    n1987 = local read "Reward given"() -> (w2857:bool)
                    n1988 = call "Is Value Changed.vim"("value"=w2857) -> ("changed or first call?"=w2858:bool)
                    n1989 = And(x=w2857, y=w2858) -> (x .and. y?=w2856:bool)
                    n1990 = case shown="True" w2856 {
                      frame False {
                      }
                      frame True {
                        n1991 = local write "Start mask stim"(TRUE ("Start light stim")) -> ()
                        n1992 = local write "Stop mask stim"(FALSE ("Stop light stim")) -> ()
                      }
                    }
                  }
                }
                n1993 = case shown="True" w2829 {
                  tunnel: w2831 -> [w2838 _]
                  tunnel: w2830 -> [w2839 _]
                  frame False {
                    n1994 = Greater?(x=w2839, y=w2838) -> (0:w2837:bool)
                    n1995 = call "Is Value Changed.vim"("value"=w2837) -> ("changed or first call?"=w2836:bool)
                    n1996 = And(x=w2837, y=w2836) -> (x .and. y?=w2835:bool)
                    n1997 = case shown="True" w2835 {
                      frame False {
                      }
                      frame True {
                        n1998 = local write "Stop mask stim"(TRUE ("Stop light stim")) -> ()
                      }
                    }
                  }
                  frame True {
                    n1999 = local read "Reward given"() -> (w2842:bool)
                    n2000 = call "Is Value Changed.vim"("value"=w2842) -> ("changed or first call?"=w2843:bool)
                    n2001 = And(x=w2842, y=w2843) -> (x .and. y?=w2841:bool)
                    n2002 = case shown="True" w2841 {
                      frame False {
                      }
                      frame True {
                        n2003 = local write "Stop mask stim"(TRUE ("Stop light stim")) -> ()
                      }
                    }
                  }
                }
              }
              frame True {
                n2004 = local write "Stop mask stim"(TRUE ("Stop light stim")) -> ()
              }
            }
            n2005 = local read "Start mask stim"() -> (w2798:bool)
            n2006 = case shown="False" w2798 {
              tunnel: [w2863 w2873] -> w2795
              tunnel: 5.0 -> [_ w2872]
              tunnel: 0.0 -> [_ w2871]
              tunnel: w2820 -> [_ w2869]
              tunnel: w2822 -> [_ w2868]
              frame False {
                n2007 = local read "Start light stim"() -> (w2862:bool)
                n2008 = case shown="False" w2862 {
                  tunnel: [w2864 w2866] -> w2863
                  frame True {
                    n2009 = call "Simulate Signal2"("Offset"=0.0) -> ("DC"=w2864:dynamicdata)  [unwired: 13 in, 1 out]
                  }
                  frame False {
                    n2010 = call "Simulate Signal9"("Offset"=0.0) -> ("DC"=w2866:dynamicdata)  [unwired: 13 in, 1 out]
                  }
                }
              }
              frame True {
                # "min V value"
                # "max V value"
                n2011 = local read "Stop mask stim"() -> (w2876:bool)
                n2012 = call "Simulate Signal5"("Offset"=w2871) -> ("DC"=w2874:dynamicdata)  [unwired: 13 in, 1 out]
                n2013 = Subtract(x=w2872, y=w2871) -> (x-y=w2870:dbl)
                n2014 = case shown="False" w2868 {
                  tunnel: [w2879 w2885] -> w2878
                  tunnel: w2870 -> [w2880 w2883]
                  tunnel: w2869 -> [_ w2881]
                  frame True {
                    n2015 = call "Simulate Signal6"("Offset"=w2880) -> ("Sine"=w2879:dynamicdata)  [unwired: 13 in, 1 out]
                  }
                  frame False {
                    n2016 = Divide(x=w2883, y=2.0) -> (x/y=w2882:dbl)
                    n2017 = call "Simulate Signal7"("Offset"=w2882, "Frequency"=w2881, "Amplitude"=w2882) -> ("Sine"=w2885:dynamicdata)  [unwired: 11 in, 1 out]
                  }
                }
                n2018 = case shown="True" w2876 {
                  tunnel: [w2886 w2889] -> w2877
                  frame False {
                    n2019 = call "Simulate Signal3"() -> ("DC"=w2886:dynamicdata)  [unwired: 14 in, 1 out]
                  }
                  frame True {
                    n2020 = call "Simulate Signal4"() -> ("Triangle"=w2889:dynamicdata)  [unwired: 14 in, 1 out]
                    n2021 = local write "Stop mask stim"(FALSE ("Stop light stim")) -> ()
                    n2022 = local write "Start mask stim"(FALSE ("Start light stim")) -> ()
                  }
                }
                n2023 = Multiply(1:w2877, 2:w2878) -> (0:w2875:dynamicdata)  [unwired: 1 in, 1 out]
                n2024 = Add(1:w2874, 2:w2875) -> (0:w2873:dynamicdata)  [unwired: 1 in, 1 out]
              }
            }
          }
          frame Enabled {
          }
        }
        n2025 = local read "Stim prot command"() -> (w2751:u16)
        n2026 = local read "protocol array"() -> (w2747:string[][])
        n2027 = Tick Count (ms)() -> (millisecond timer value=w2725:u32)
        n2028 = Subtract(x=w2725, y=w2726) -> (x-y=w2724:u32)
        n2029 = Divide(x=u32 1000, y=w2724) -> (x/y=→"stim loop rate":dbl)
        n2030 = Index Array(array=w2747, index (row)=w2751, index (col)=4) -> (element=w2749:string)
        n2031 = Index Array(array=w2747, index (row)=w2751, index (col)=3 ("disabled index (col)")) -> (element=w2761:string)
        n2032 = Index Array(array=w2747, index (row)=w2751, index (col)=0 ("index (row)")) -> (element=w2757:string)
        n2033 = Index Array(array=w2747, index (row)=w2751, index (col)=1 ("disabled index (col)")) -> (element=w2786:string)
        n2034 = Index Array(array=w2747, index (row)=w2751, index (col)=2 ("disabled index (col)")) -> (element=w2791:string)
        n2035 = local read "Relative position"() -> (w2771:dbl)
        n2036 = Match Pattern(string=w2761, regular expression="int. ") -> (after substring=w2759:string)  [unwired: 1 in, 3 out]
        n2037 = Match Pattern(string=w2749, regular expression="duty cycle ") -> (after substring=w2745:string)  [unwired: 1 in, 3 out]
        n2038 = Match Pattern(string=w2757, regular expression="continuous") -> (match substring=w2754:string)  [unwired: 1 in, 3 out]
        n2039 = Match Pattern(string=w2757, regular expression="sinus") -> (match substring=w2753:string)  [unwired: 1 in, 3 out]
        n2040 = Match Pattern(string=w2757, regular expression="square") -> (match substring=w2752:string)  [unwired: 1 in, 3 out]
        n2041 = local read "Enable stim."() -> (w2764:bool)
        n2042 = Subtract(x=w2725, y=w2733) -> (x-y=w2732:u32)
        n2043 = Match Pattern(string=w2759, regular expression=w2744) -> (before substring=w2792:string)  [unwired: 1 in, 3 out]
        n2044 = Match Pattern(string=w2757, regular expression=" Hz") -> (before substring=w2746:string)  [unwired: 1 in, 3 out]
        n2045 = Match Pattern(string=w2757, regular expression=w2766) -> (match substring=w2765:string)  [unwired: 1 in, 3 out]
        n2046 = Match Pattern(string=w2786, regular expression="from ") -> (after substring=w2783:string)  [unwired: 1 in, 3 out]
        n2047 = Match Pattern(string=w2786, regular expression=w2785) -> (match substring=w2784:string)  [unwired: 1 in, 3 out]
        n2048 = Match Pattern(string=w2791, regular expression="to ") -> (after substring=w2789:string)  [unwired: 1 in, 3 out]
        n2049 = Match Pattern(string=w2791, regular expression=w2787) -> (match substring=w2788:string)  [unwired: 1 in, 3 out]
        n2050 = Match Pattern(string=w2745, regular expression=w2744) -> (before substring=w2743:string)  [unwired: 1 in, 3 out]
        n2051 = Concatenate Strings(w2754, w2753, w2752) -> (w2737:string)
        n2052 = Greater?(x=w2732, y=u32 10000) -> (0:w2730:bool)
        n2053 = Not(x=w2764) -> (.not. x?=w2763:bool)
        n2054 = Equal?(x=w2765, y=w2766) -> (x = y?=w2762:bool)
        n2055 = Equal?(x=w2784, y=w2785) -> (x = y?=w2768:bool)
        n2056 = Equal?(x=w2788, y=w2787) -> (x = y?=w2770:bool)
        n2057 = Decimal String To Number(string=w2792) -> (number=w2735:i32)  [unwired: 2 in, 1 out]
        n2058 = Decimal String To Number(string=w2743) -> (number=w2742:i32)  [unwired: 2 in, 1 out]
        n2059 = Decimal String To Number(string=w2746) -> (number=w2775:i32)  [unwired: 2 in, 1 out]
        n2060 = Decimal String To Number(string=w2783) -> (number=w2773:i32)  [unwired: 2 in, 1 out]
        n2061 = Decimal String To Number(string=w2789) -> (number=w2772:i32)  [unwired: 2 in, 1 out]
        n2062 = Or(x=w2763, y=w2762) -> (x .or. y?=w2767:bool)
        n2063 = case shown="False" w2767 {
          tunnel: w2773 -> [w2908 _]
          tunnel: w2768 -> [w2907 _]
          tunnel: w2771 -> [w2906 _]
          tunnel: w2772 -> [w2905 _]
          tunnel: w2771 -> [w2904 _]
          tunnel: w2770 -> [w2903 _]
          tunnel: w2737 -> [w2900 _]
          tunnel: [w2899 w2943] -> w2736
          tunnel: w2735 -> [w2897 _]
          tunnel: [w2895 w2944] -> w2728
          tunnel: w2730 -> [w2894 _]
          frame False {
            n2064 = case shown="False" w2907 {
              tunnel: w2908 -> [w2934 _]
              tunnel: w2906 -> [w2929 _]
              frame False {
                n2065 = Greater Or Equal?(x=w2929, y=w2934) -> (x >= y?=w2927:bool)
                n2066 = call "Is New Trial.vi"("Position data"=w2929) -> ("Boolean"=w2930:bool)  [unwired: 1 in]
                n2067 = call "Is Value Changed.vim"("value"=w2927) -> ("changed or first call?"=w2932:bool)
                n2068 = Compound Arithmetic op=OR(w2932, w2930) -> (w2931:bool)
                n2069 = Not(x=w2927) -> (.not. x?=w2928:bool)
                n2070 = And(x=w2927, y=w2931) -> (x .and. y?=w2933:bool)
                n2071 = case shown="True" w2928 {
                  frame False {
                  }
                  frame True {
                    n2072 = local write "Stop light stim"(TRUE ("Stop light stim")) -> ()
                  }
                }
                n2073 = case shown="True" w2933 {
                  frame False {
                  }
                  frame True {
                    n2074 = local write "Start light stim"(TRUE ("Start light stim")) -> ()
                    n2075 = local write "Stop light stim"(FALSE ("Stop light stim")) -> ()
                  }
                }
              }
              frame True {
                n2076 = local read "Reward given"() -> (w2939:bool)
                n2077 = call "Is Value Changed.vim"("value"=w2939) -> ("changed or first call?"=w2940:bool)
                n2078 = And(x=w2939, y=w2940) -> (x .and. y?=w2938:bool)
                n2079 = case shown="True" w2938 {
                  frame False {
                  }
                  frame True {
                    n2080 = local write "Start light stim"(TRUE ("Start light stim")) -> ()
                    n2081 = local write "Stop light stim"(FALSE ("Stop light stim")) -> ()
                  }
                }
              }
            }
            n2082 = case shown="False" w2903 {
              tunnel: w2905 -> [w2918 _]
              tunnel: w2904 -> [w2919 _]
              tunnel: w2894 -> [w2913 w2921]
              frame False {
                n2083 = Greater?(x=w2919, y=w2918) -> (0:w2917:bool)
                n2084 = call "Is Value Changed.vim"("value"=w2917) -> ("changed or first call?"=w2916:bool)
                n2085 = And(x=w2917, y=w2916) -> (x .and. y?=w2915:bool)
                n2086 = Or(x=w2915, y=w2913) -> (x .or. y?=w2914:bool)
                n2087 = case shown="True" w2914 {
                  frame False {
                  }
                  frame True {
                    n2088 = local write "Stop light stim"(TRUE ("Stop light stim")) -> ()
                  }
                }
              }
              frame True {
                n2089 = local read "Reward given"() -> (w2924:bool)
                n2090 = call "Is Value Changed.vim"("value"=w2924) -> ("changed or first call?"=w2925:bool)
                n2091 = And(x=w2924, y=w2925) -> (x .and. y?=w2923:bool)
                n2092 = Or(x=w2923, y=w2921) -> (x .or. y?=w2922:bool)
                n2093 = case shown="True" w2922 {
                  frame False {
                  }
                  frame True {
                    n2094 = local write "Stop light stim"(TRUE ("Stop light stim")) -> ()
                  }
                }
              }
            }
            n2095 = Divide(x=w2897, y=100) -> (x/y=w2896:dbl)
            n2096 = Equal?(x=w2900, y="") -> (x = y?=w2902:bool)
            n2097 = case shown="False" w2902 {
              tunnel: w2900 -> [w2910 _]
              tunnel: [w2910 w2912] -> w2899
              tunnel: w2896 -> [w2909 _]
              tunnel: [w2909 w2911] -> w2895
              frame False {
                n2098 = local write "prev. max stim. V"(w2909) -> ()
                n2099 = local write "prev. stim. type"(w2910) -> ()
              }
              frame True {
                n2100 = local read "prev. stim. type"() -> (w2912:string)
                n2101 = local read "prev. max stim. V"() -> (w2911:dbl)
              }
            }
          }
          frame True {
            n2102 = local write "Stop light stim"(TRUE ("Stop light stim")) -> ()
            n2103 = local read "prev. max stim. V"() -> (w2944:dbl)
            n2104 = local read "prev. stim. type"() -> (w2943:string)
          }
        }
        n2105 = Subtract(x=w2729, y=w2739) -> (x-y=w2738:dbl)
        n2106 = local read "Start light stim"() -> (w2793:bool)
        n2107 = local read "Exit"() -> (w2741:bool)
        n2108 = Multiply(x=w2729, y=w2728) -> (x*y=w2727:dbl)
        n2109 = Multiply(x=w2738, y=w2728) -> (x*y=w2776:dbl)
        n2110 = case shown="True" w2741 {
          tunnel: [FALSE w2997] -> w2794
          frame False {
          }
          frame True {
            n2111 = flat-sequence {
              tunnel: [TRUE] -> w2997
              frame #0 {
                n2112 = Wait (ms)(milliseconds to wait=u32 100) -> ()  [unwired: 1 out]
              }
              frame #1 {
              }
            }
          }
        }
        n2113 = case shown="True" w2793 {
          selector: w2793 -> [w2946 w2954]
          tunnel: [w2949 w2964] -> w2758
          tunnel: w2776 -> [_ w2959]
          tunnel: w2739 -> [_ w2956]
          tunnel: w2775 -> [_ w2963]
          tunnel: w2736 -> [_ w2962]
          tunnel: w2742 -> [_ w2961]
          tunnel: [w2947 w2958] -> w2734
          tunnel: w2733 -> [_ w2958]
          tunnel: w2727 -> [_ w2957]
          frame False {
            n2114 = local read "Start mask stim"() -> (w2948:bool)
            n2115 = local write "stim started"(w2946) -> ()
            n2116 = case shown="False" w2948 {
              tunnel: [w2950 w2952] -> w2949
              frame True {
                n2117 = call "Simulate Signal77"("Offset"=0.0) -> ("DC"=w2950:dynamicdata)  [unwired: 13 in, 1 out]
              }
              frame False {
                n2118 = call "Simulate Signal8"("Offset"=0.0) -> ("DC"=w2952:dynamicdata)  [unwired: 13 in, 1 out]
              }
            }
            n2119 = Tick Count (ms)() -> (millisecond timer value=w2947:u32)
          }
          frame True {
            # "min V value"
            # "max V value"
            n2120 = local write "stim started"(w2954) -> ()
            n2121 = local read "Stop light stim"() -> (w2967:bool)
            n2122 = case shown="\"continuous\", Default" w2962 {
              tunnel: [w2970 w2977 w2984] -> w2960
              tunnel: w2959 -> [w2971 w2975 _]
              tunnel: w2963 -> [_ w2973 w2981]
              tunnel: w2961 -> [_ _ w2980]
              tunnel: w2957 -> [_ _ w2979]
              tunnel: w2956 -> [w2969 w2972 _]
              tunnel: [w2969 w2972 0.0] -> w2955
              frame "continuous", Default {
                n2123 = call "Simulate Signal78"("Offset"=w2971) -> ("Sine"=w2970:dynamicdata)  [unwired: 13 in, 1 out]
              }
              frame "sinus" {
                n2124 = Divide(x=w2975, y=2.0) -> (x/y=w2974:dbl)
                n2125 = call "Simulate Signal"("Offset"=w2974, "Frequency"=w2973, "Amplitude"=w2974) -> ("Sine"=w2977:dynamicdata)  [unwired: 11 in, 1 out]
              }
              frame "square" {
                n2126 = Divide(x=w2979, y=2.0) -> (x/y=w2982:dbl)
                n2127 = call "Simulate Signal10"("Offset"=w2982, "Duty Cycle (%)"=w2980, "Frequency"=w2981, "Amplitude"=w2982) -> ("Square"=w2984:dynamicdata)  [unwired: 10 in, 1 out]
              }
            }
            n2128 = call "Simulate Signal81"("Offset"=w2955) -> ("DC"=w2965:dynamicdata)  [unwired: 13 in, 1 out]
            n2129 = case shown="True" w2967 {
              tunnel: [w2988 w2995] -> w2968
              frame False {
                n2130 = local read "start with ramp"() -> (w2986:bool)
                n2131 = local read "start of stim"() -> (w2987:bool)
                n2132 = And(x=w2987, y=w2986) -> (x .and. y?=w2985:bool)
                n2133 = case shown="False" w2985 {
                  tunnel: [w2990 w2991] -> w2988
                  frame True {
                    n2134 = call "Simulate Signal12"() -> ("Triangle"=w2990:dynamicdata)  [unwired: 14 in, 1 out]
                    n2135 = local write "start of stim"(FALSE ("start of stim")) -> ()
                  }
                  frame False {
                    n2136 = call "Simulate Signal79"() -> ("DC"=w2991:dynamicdata)  [unwired: 14 in, 1 out]
                  }
                }
              }
              frame True {
                n2137 = call "Simulate Signal80"() -> ("Triangle"=w2995:dynamicdata)  [unwired: 14 in, 1 out]
                n2138 = local write "Stop light stim"(FALSE ("Stop light stim")) -> ()
                n2139 = local write "Start light stim"(FALSE ("Start light stim")) -> ()
                n2140 = local write "start of stim"(TRUE ("start of stim")) -> ()
              }
            }
            n2141 = Multiply(1:w2968, 2:w2960) -> (0:w2966:dynamicdata)  [unwired: 1 in, 1 out]
            n2142 = Add(1:w2965, 2:w2966) -> (0:w2964:dynamicdata)  [unwired: 1 in, 1 out]
          }
        }
        n2143 = disable-structure shown="Disabled" {
          disable-tunnel: w2769 -> [w2892 _]
          disable-tunnel: w2758 -> [w2891 w2893]
          disable-tunnel: [w2890 w2893] -> w2740
          frame Disabled {
            n2144 = Merge Signals(w2891, w2892) -> (w2890:dynamicdata)
          }
          frame Enabled {
          }
        }
        "Waveform Graph" <- w2740
        n2145 = call "DAQ Assistant"("data"=w2740, "stop (T)"=w2741) -> ()  [unwired: 16 in, 2 out]
      }
      n2146 = call <vilib>:"DAQmx Clear Task.vi"("task in"=w2248, "error in"=w2247) -> ()  [unwired: 13 in, 1 out]
    }
  }
  n2147 = while {
    shift-right: [w3024] -> _
    shift-left: _ -> [w3023]
    stop <- w3025 stop-if-true
    n2148 = local read "VR Mode"() -> (w3020:bool)
    n2149 = case shown="True" w3020 {
      tunnel: [w3074 w3168] -> w3024
      tunnel: w3023 -> [w3069 w3163]
      frame True {
        w3046 = FALSE ("t")
        # "Clear graph history in every 3 min"
        n2150 = local read "Stim trial"() -> (w3065:bool)
        n2151 = Tick Count (ms)() -> (millisecond timer value=w3073:u32)
        n2152 = Divide(x=w3073, y=u32 60000) -> (x/y=w3071:dbl)
        n2153 = Not(x=w3065) -> (.not. x?=w3064:bool)
        n2154 = Subtract(x=w3071, y=w3069) -> (x-y=w3070:dbl)
        n2155 = case shown="False" w3064 {
          tunnel: [TRUE ("Enable") FALSE ("Enable")] -> w3047
          tunnel: [TRUE ("Enable") FALSE ("Enable")] -> w3061
          tunnel: [TRUE ("Enable") FALSE ("Enable")] -> w3058
          tunnel: [FALSE ("Enable") TRUE ("Enable")] -> w3055
          tunnel: [FALSE ("Enable") TRUE ("Enable")] -> w3049
          tunnel: [FALSE ("Enable") TRUE ("Enable")] -> w3052
          frame True {
          }
          frame False {
          }
        }
        n2156 = Greater?(x=w3070, y=3.0) -> (0:w3066:bool)
        n2157 = local read "Unity position:"() -> (w3039:sgl)
        n2158 = local read "velocity (cm/s)"() -> (w3045:dbl)
        n2159 = Select(t=w3046, s=w3046, f=w3047) -> (s? t:f=w3063:bool)
        n2160 = Select(t=FALSE, s=w3046, f=w3061) -> (s? t:f=w3062:bool)
        n2161 = Select(t=FALSE, s=w3046, f=w3058) -> (s? t:f=w3059:bool)
        n2162 = Select(t=FALSE, s=w3046, f=w3055) -> (s? t:f=w3056:bool)
        n2163 = Select(t=FALSE, s=w3046, f=w3052) -> (s? t:f=w3053:bool)
        n2164 = Select(t=FALSE, s=w3046, f=w3049) -> (s? t:f=w3050:bool)
        n2165 = call "Is New Trial - graph loop.vi"("Position data"=w3039) -> ("Boolean"=w3040:bool)  [unwired: 1 in]
        n2166 = case shown="False" w3066 {
          tunnel: [w3126 w3135] -> w3074
          tunnel: w3069 -> [w3127 _]
          tunnel: ["Reset bottom plot" w3134] -> w3067
          tunnel: ["Reset top plot" w3134] -> w3044
          frame False {
            n2167 = Or(x="Reset bottom plot", y="Reset top plot") -> (x .or. y?=w3125:bool)
            n2168 = case shown="True" w3125 {
              tunnel: w3127 -> [w3130 _]
              tunnel: [w3130 w3131] -> w3126
              frame False {
              }
              frame True {
                n2169 = Tick Count (ms)() -> (millisecond timer value=w3133:u32)
                n2170 = Divide(x=w3133, y=u32 60000) -> (x/y=w3131:dbl)
              }
            }
          }
          frame True {
            w3134 = TRUE ("Reset NBC plot")
            n2171 = Tick Count (ms)() -> (millisecond timer value=w3136:u32)
            n2172 = Divide(x=w3136, y=u32 60000) -> (x/y=w3135:dbl)
          }
        }
        n2173 = local read "Valve open"() -> (w3089:bool)
        n2174 = local read "Unity position:"() -> (w3085:sgl)
        n2175 = local read "lick signal"() -> (w3110:i8[])
        n2176 = local read "Unity position:"() -> (w3116:sgl)
        n2177 = call "Is Value Changed.vim"("value"=w3040) -> ("changed or first call?"=w3043:bool)
        n2178 = local read "Valve open"() -> (w3083:bool)
        n2179 = local read "Unity position:"() -> (w3095:sgl)
        n2180 = local read "Unity position:"() -> (w3094:sgl)
        n2181 = local read "lick signal"() -> (w3101:i8[])
        n2182 = case shown="False" w3040 {
          tunnel: [w3119 w3123] -> w3041
          tunnel: w3045 -> [w3120 w3123]
          tunnel: w3039 -> [w3122 _]
          tunnel: [w3122 inf ("velocity (cm/s)")] -> w3042
          tunnel: w3043 -> [w3118 _]
          frame False {
            n2183 = Select(t=-inf ("velocity (cm/s)"), s=w3118, f=w3120) -> (s? t:f=w3119:dbl)
          }
          frame True {
          }
        }
        n2184 = Boolean To (0,1)(Boolean=w3089) -> (0, 1=w3087:i16)
        n2185 = Index Array(array=w3110, index=0) -> (element=w3107:i8)
        n2186 = Multiply(x=w3107, y=100) -> (x*y=w3106:i32)
        n2187 = Multiply(x=w3087, y=-20) -> (x*y=w3088:i32)
        n2188 = Boolean To (0,1)(Boolean=w3083) -> (0, 1=w3081:i16)
        n2189 = Index Array(array=w3101, index=0) -> (element=w3103:i8)
        n2190 = Multiply(x=w3081, y=-20) -> (x*y=w3082:i32)
        n2191 = Multiply(x=w3103, y=100) -> (x*y=w3075:i32)
        n2192 = call "Build XY Graph"("Enable"=w3063, "Reset"=w3044, "Y Input"=w3041, "X Input"=w3042) -> ("XY Graph"=w3112:cluster{"X":dbl[], "Y":dbl[]}[])  [unwired: 6 in, 1 out]
        n2193 = call "Build XY Graph4"("Enable"=w3062, "Reset"=w3044, "Y Input"=w3106, "X Input"=w3116) -> ("XY Graph"=w3115:cluster{"X":dbl[], "Y":dbl[]}[])  [unwired: 6 in, 1 out]
        n2194 = call "Build XY Graph3"("Enable"=w3059, "Reset"=w3044, "Y Input"=w3088, "X Input"=w3085) -> ("XY Graph"=w3100:cluster{"X":dbl[], "Y":dbl[]}[])  [unwired: 6 in, 1 out]
        n2195 = call "Build XY Graph2"("Enable"=w3053, "Reset"=w3067, "Y Input"=w3075, "X Input"=w3095) -> ("XY Graph"=w3090:cluster{"X":dbl[], "Y":dbl[]}[])  [unwired: 6 in, 1 out]
        n2196 = call "Build XY Graph5"("Enable"=w3056, "Reset"=w3067, "Y Input"=w3041, "X Input"=w3042) -> ("XY Graph"=w3097:cluster{"X":dbl[], "Y":dbl[]}[])  [unwired: 6 in, 1 out]
        n2197 = call "Build XY Graph6"("Enable"=w3050, "Reset"=w3067, "Y Input"=w3082, "X Input"=w3094) -> ("XY Graph"=w3093:cluster{"X":dbl[], "Y":dbl[]}[])  [unwired: 6 in, 1 out]
        n2198 = Index Array(array=w3112, index=0) -> (element=w3076:cluster{"X":dbl[], "Y":dbl[]})
        n2199 = Index Array(array=w3115, index=0) -> (element=w3111:cluster{"X":dbl[], "Y":dbl[]})
        n2200 = Index Array(array=w3100, index=0) -> (element=w3096:cluster{"X":dbl[], "Y":dbl[]})
        n2201 = Index Array(array=w3097, index=0) -> (element=w3080:cluster{"X":dbl[], "Y":dbl[]})
        n2202 = Index Array(array=w3090, index=0) -> (element=w3079:cluster{"X":dbl[], "Y":dbl[]})
        n2203 = Index Array(array=w3093, index=0) -> (element=w3078:cluster{"X":dbl[], "Y":dbl[]})
        n2204 = Build Array(w3080, w3079, w3078) -> (→"Bottom Graph":cluster{"X":dbl[], "Y":dbl[]}[])
        n2205 = Build Array(w3076, w3111, w3096) -> (→"Top Graph":cluster{"X":dbl[], "Y":dbl[]}[])
        n2206 = Wait (ms)(milliseconds to wait=u32 20) -> ()  [unwired: 1 out]
      }
      frame False {
        # "Clear graph history in every 5 min"
        n2207 = local read "Reward zone"() -> (w3157:bool)
        n2208 = Tick Count (ms)() -> (millisecond timer value=w3167:u32)
        n2209 = case shown="False" w3157 {
          tunnel: [w3219 w3225] -> w3159
          frame False {
            n2210 = local read "total distance cm"() -> (w3221:sgl[])
            n2211 = local read "Prev. rew. pos."() -> (w3222:dbl)
            n2212 = Array Max & Min(array=w3221) -> (max value=w3220:sgl)  [unwired: 3 out]
            n2213 = Subtract(x=w3220, y=w3222) -> (x-y=w3219:dbl)
          }
          frame True {
            n2214 = local read "total distance cm"() -> (w3224:sgl[])
            n2215 = local read "prev. diode position"() -> (w3226:dbl)
            n2216 = Array Max & Min(array=w3224) -> (max value=w3223:sgl)  [unwired: 3 out]
            n2217 = Subtract(x=w3223, y=w3226) -> (x-y=w3225:dbl)
          }
        }
        n2218 = local read "Reward freq. (cm)"() -> (w3155:dbl)
        n2219 = local read "Prev. rew. pos."() -> (w3156:dbl)
        n2220 = local read "total distance cm"() -> (w3152:sgl[])
        n2221 = Divide(x=w3167, y=u32 60000) -> (x/y=w3165:dbl)
        n2222 = Subtract(x=w3165, y=w3163) -> (x-y=w3164:dbl)
        n2223 = local read "prev. diode position"() -> (w3153:dbl)
        n2224 = Greater?(x=w3164, y=2.0) -> (0:w3160:bool)
        n2225 = Compound Arithmetic op=ADD(w3156, w3155, 20.0 ("value")) -> ()  [unwired: 1 out]
        n2226 = case shown="True" w3160 {
          tunnel: [w3228 w3235] -> w3168
          tunnel: w3163 -> [w3229 _]
          tunnel: ["Reset wheel pos. graph" TRUE ("Reset NBC plot")] -> w3161
          frame False {
            n2227 = case shown="False" "Reset wheel pos. graph" {
              tunnel: w3229 -> [w3230 _]
              tunnel: [w3230 w3231] -> w3228
              frame False {
              }
              frame True {
                n2228 = Tick Count (ms)() -> (millisecond timer value=w3233:u32)
                n2229 = Divide(x=w3233, y=u32 60000) -> (x/y=w3231:dbl)
              }
            }
          }
          frame True {
            n2230 = Tick Count (ms)() -> (millisecond timer value=w3236:u32)
            n2231 = Divide(x=w3236, y=u32 60000) -> (x/y=w3235:dbl)
          }
        }
        n2232 = Array Max & Min(array=w3152) -> (max value=w3151:sgl)  [unwired: 3 out]
        n2233 = Subtract(x=w3151, y=w3153) -> ()  [unwired: 1 out]
        n2234 = local read "lick signal"() -> (w3182:i8[])
        n2235 = local read "Valve open"() -> (w3173:bool)
        n2236 = local read "velocity (cm/s)"() -> (w3150:dbl)
        n2237 = Index Array(array=w3182, index=0) -> (element=w3179:i8)
        n2238 = local read "Run experiment"() -> (w3158:bool)
        n2239 = Boolean To (0,1)(Boolean=w3173) -> (0, 1=w3171:i16)
        n2240 = Multiply(x=w3179, y=100) -> (x*y=w3178:i32)
        n2241 = Multiply(x=w3171, y=-20) -> (x*y=w3172:i32)
        n2242 = call "Build XY Graph7"("Reset"=w3161, "Y Input"=w3150, "X Input"=w3159) -> ("XY Graph"=w3184:cluster{"X":dbl[], "Y":dbl[]}[])  [unwired: 7 in, 1 out]
        n2243 = call "Build XY Graph8"("Reset"=w3161, "Y Input"=w3178, "X Input"=w3159) -> ("XY Graph"=w3187:cluster{"X":dbl[], "Y":dbl[]}[])  [unwired: 7 in, 1 out]
        n2244 = call "Build XY Graph9"("Reset"=w3161, "Y Input"=w3172, "X Input"=w3159) -> ("XY Graph"=w3176:cluster{"X":dbl[], "Y":dbl[]}[])  [unwired: 7 in, 1 out]
        n2245 = disable-structure shown="Disabled" {
          disable-tunnel: w3158 -> [w3189 _]
          frame Disabled {
            n2246 = case shown="True" w3189 {
              frame False {
              }
              frame True {
                # "Light ON/OFF  indicators"
                n2247 = local read "shuffled array"() -> (w3212:i16[])
                n2248 = local read "Trial types"() -> (w3213:u16[][])
                n2249 = Index Array(array=w3213, index (row)=1) -> (element=w3206:u16[])  [unwired: 1 in]
                n2250 = Index Array(array=w3212, index=0) -> (element=w3211:i16)
                n2251 = Index Array(array=w3212, index=1) -> (element=w3207:i16)
                n2252 = Index Array(array=w3212, index=2) -> (element=w3208:i16)
                n2253 = Index Array(array=w3212, index=3) -> (element=w3209:i16)
                n2254 = Index Array(array=w3212, index=4) -> (element=w3210:i16)
                n2255 = Index Array(array=w3206, index=w3211) -> (element=w3205:u16)
                n2256 = Index Array(array=w3206, index=w3207) -> (element=w3204:u16)
                n2257 = Index Array(array=w3206, index=w3208) -> (element=w3203:u16)
                n2258 = Index Array(array=w3206, index=w3209) -> (element=w3201:u16)
                n2259 = Index Array(array=w3206, index=w3210) -> (element=w3202:u16)
                n2260 = Number To Boolean Array(number=w3205) -> (Boolean array=w3214:bool[])
                n2261 = Number To Boolean Array(number=w3203) -> (Boolean array=w3217:bool[])
                n2262 = Number To Boolean Array(number=w3201) -> (Boolean array=w3216:bool[])
                n2263 = Number To Boolean Array(number=w3202) -> (Boolean array=w3218:bool[])
                n2264 = Number To Boolean Array(number=w3204) -> (Boolean array=w3215:bool[])
                n2265 = Index Array(array=w3214, index=0) -> ()  [unwired: 1 out]
                n2266 = Index Array(array=w3215, index=0) -> ()  [unwired: 1 out]
                n2267 = Index Array(array=w3217, index=0) -> ()  [unwired: 1 out]
                n2268 = Index Array(array=w3216, index=0) -> ()  [unwired: 1 out]
                n2269 = Index Array(array=w3218, index=0) -> ()  [unwired: 1 out]
                n2270 = local read item#-1() -> ()  [unwired: 1 in]
                n2271 = local read item#-1() -> ()  [unwired: 1 in]
                n2272 = local read item#-1() -> ()  [unwired: 1 in]
                n2273 = local read item#-1() -> ()  [unwired: 1 in]
                n2274 = local read item#-1() -> ()  [unwired: 1 in]
              }
            }
          }
          frame Enabled {
          }
        }
        n2275 = Index Array(array=w3184, index=0) -> (element=w3169:cluster{"X":dbl[], "Y":dbl[]})
        n2276 = Index Array(array=w3187, index=0) -> (element=w3183:cluster{"X":dbl[], "Y":dbl[]})
        n2277 = Index Array(array=w3176, index=0) -> (element=w3174:cluster{"X":dbl[], "Y":dbl[]})
        n2278 = Build Array(w3169, w3183, w3174) -> (→"Wheel position graph":cluster{"X":dbl[], "Y":dbl[]}[])
        n2279 = Wait (ms)(milliseconds to wait=u32 20) -> ()  [unwired: 1 out]
      }
    }
    n2280 = local write "Stop recording"("Stop recording") -> ()
    n2281 = local write "Lab book notes"("Lab book notes") -> ()
    n2282 = local write "SciScan"("SciScan") -> ()
    n2283 = local write "Reward zone"("Reward zone") -> ()
    n2284 = Not(x="Reward zone") -> (.not. x?=w3012:bool)
    n2285 = property on="Reward freq. (cm)" class="DigNum (strict)"("Visible"=w3012) -> ()  [unwired: 2 in, 2 out]
    n2286 = property on="Timed reward (s)" class="DigNum (strict)"("Visible"=w3012) -> ()  [unwired: 2 in, 2 out]
    n2287 = local read "Exit"() -> (w3025:bool)
    n2288 = local read "Active licking"() -> (w3014:bool)
    n2289 = local read "Reward zone"() -> (w3015:bool)
    n2290 = local read "Frame signal 2"() -> (w3001:i8[])
    n2291 = local read "Frame signal"() -> (w3002:i8[])
    n2292 = call "Is Value Changed.vim"("value"=w3014) -> ("changed or first call?"=w3013:bool)
    n2293 = call "Is Value Changed.vim"("value"=w3015) -> ("changed or first call?"=w3016:bool)
    n2294 = case shown="True" w3016 {
      tunnel: w3015 -> [_ w3030]
      frame False {
      }
      frame True {
        n2295 = case shown="True" w3030 {
          frame False {
            n2296 = local write "Active licking"(FALSE ("Enable")) -> ()
            n2297 = property on="Random reward" class="Bool (strict)"("DisabledEnum"=T7."Enabled" ("Disabled"), "Visible"=TRUE) -> ()  [unwired: 2 in, 2 out]
          }
          frame True {
            n2298 = local write "Active licking"(TRUE ("Enable")) -> ()
            n2299 = local write "Random reward"(FALSE ("Random reward")) -> ()
            n2300 = property on="Random reward" class="Bool (strict)"("DisabledEnum"=T7."Disabled" ("Disabled"), "Visible"=FALSE) -> ()  [unwired: 2 in, 2 out]
          }
        }
      }
    }
    n2301 = case shown="True" w3013 {
      frame False {
      }
      frame True {
        n2302 = local read "Active licking"() -> (w3026:bool)
        n2303 = Select(t=T7."Enabled" ("Disabled"), s=w3026, f=T7."Disabled and Grayed Out") -> (s? t:f=w3028:T7)
        n2304 = property on="Hybrid licking" class="Bool (strict)"("DisabledEnum"=w3028) -> ()  [unwired: 2 in, 2 out]
      }
    }
    n2305 = case shown="True" "Random reward" {
      frame False {
      }
      frame True {
        n2306 = local write "Active licking"(FALSE ("Enable")) -> ()
      }
    }
    n2307 = Add Array Elements(numeric array=w3001) -> (sum=w3006:i8)
    n2308 = Add Array Elements(numeric array=w3002) -> (sum=w3007:i8)
    n2309 = Array Size(array=w3001) -> (size(s)=w3003:i32)
    n2310 = Array Size(array=w3002) -> (size(s)=w3011:i32)
    n2311 = Divide(x=w3006, y=w3003) -> (x/y=w3004:dbl)
    n2312 = Divide(x=w3007, y=w3011) -> (x/y=w3010:dbl)
    n2313 = Greater?(x=w3004, y=0.5) -> (0:→"Frame signal indicator 2":bool)
    n2314 = Greater?(x=w3010, y=0.5) -> (0:→"Frame signal indicator":bool)
  }
  n2315 = property on="Stop light stim" class="Bool (strict)"("Visible"=FALSE) -> ()  [unwired: 2 in, 2 out]
  n2316 = property on="Light ON" class="Bool (strict)"("Visible"=FALSE) -> ()  [unwired: 2 in, 2 out]
  n2317 = property on="Start light stim" class="Bool (strict)"("Visible"=FALSE) -> ()  [unwired: 2 in, 2 out]
  n2318 = property on="Stop mask stim" class="Bool (strict)"("Visible"=FALSE) -> ()  [unwired: 2 in, 2 out]
  n2319 = property on="Start mask stim" class="Bool (strict)"("Visible"=FALSE) -> ()  [unwired: 2 in, 2 out]
  n2320 = local write "Reset bottom plot"(w77) -> ()
  n2321 = local write "Reset wheel pos. graph"(w77) -> ()
  n2322 = disable-structure shown="Disabled" {
    frame Disabled {
      n2323 = local read "stim. num. 2"() -> ()  [unwired: 1 out]
      n2324 = local read "stim. num. 3"() -> ()  [unwired: 1 out]
      n2325 = local read "stim. num. 4"() -> ()  [unwired: 1 out]
      n2326 = local read "stim. num. 5"() -> ()  [unwired: 1 out]
      n2327 = local read "mask. num. 2"() -> ()  [unwired: 1 in]
      n2328 = local read "mask. num. 3"() -> ()  [unwired: 1 in]
      n2329 = local read "mask. num. 4"() -> ()  [unwired: 1 in]
      n2330 = local read "mask. num. 5"() -> ()  [unwired: 1 in]
    }
    frame Enabled {
    }
  }
  n2331 = local write "Reset top plot"(w77) -> ()
  n2332 = local write "Random reward"(FALSE ("Random reward")) -> ()
  n2333 = disable-structure shown="Disabled" {
    frame Disabled {
      n2334 = local read "Reward given"() -> (w3238:bool)
      n2335 = Not(x=w3238) -> (.not. x?=w3239:bool)
      n2336 = case shown="True" w3239 {
        tunnel: _ -> [w3242 w3248]
        tunnel: _ -> [w3241 w3250]
        tunnel: [w3242 w3243] -> _
        tunnel: [w3241 w3244] -> _
        frame False {
          n2337 = Wait (ms)(milliseconds to wait=u32 20) -> ()  [unwired: 1 out]
        }
        frame True {
          n2338 = call <vilib>:"DAQmx Start Task.vi"("task/channels in"=w3248, "error in"=w3250) -> ("task out"=w3247:refnum<k21>, "error out"=w3249:errorcluster)  [unwired: 12 in]
          n2339 = while {
            tunnel: w3247 -> [w3262]
            tunnel: w3249 -> [w3261]
            tunnel: [w3259] -> w3245
            tunnel: [w3260] -> w3246
            stop <- w3257 stop-if-true
            n2340 = local read "Primary masking light"() -> (w3252:T3)
            n2341 = call <vilib>:"DAQmx Is Task Done.vi"("task/channels in"=w3262, "error in"=w3261) -> ("task out"=w3260:refnum<k21>, "error out"=w3259:errorcluster)  [unwired: 11 in, 1 out]
            n2342 = local read "Reward given"() -> (w3256:bool)
            n2343 = Unbundle By Name(w3259) -> ("status"=w3254:bool)
            n2344 = local read "Exit"() -> (w3255:bool)
            n2345 = Not Equal?(x=w3252, y=T18."20 Hz until reward ") -> (x != y?=w3253:bool)
            n2346 = Wait (ms)(milliseconds to wait=u32 20) -> ()  [unwired: 1 out]
            n2347 = Compound Arithmetic op=OR(w3254, w3255, w3256, w3253) -> (w3257:bool)
          }
          n2348 = call <vilib>:"DAQmx Stop Task.vi"("task/channels in"=w3246, "error in"=w3245) -> ("task out"=w3243:refnum<k21>, "error out"=w3244:errorcluster)  [unwired: 12 in]
        }
      }
    }
    frame Enabled {
    }
  }
  n2349 = local read "Run experiment"() -> (w14:bool)
  n2350 = disable-structure shown="Disabled" {
    disable-tunnel: w14 -> [w3263 _]
    frame Disabled {
      n2351 = case shown="True" w3263 {
        frame False {
        }
        frame True {
          # "Light ON/OFF  indicators"
          # "Trial type indicators"
          n2352 = local read "shuffled array"() -> (w3270:i16[])
          n2353 = local read "All trials"() -> (w3271:i32)
          n2354 = local read "shuffled array"() -> (w3323:i16[])
          n2355 = local read "shuffled array"() -> (w3278:i16[])
          n2356 = local read "Trial types"() -> (w3324:u16[][])
          n2357 = local read "Trial types"() -> (w3277:u16[][])
          n2358 = local read "Trial types"() -> (w3268:u16[][])
          n2359 = Quotient & Remainder(x=w3271, y=5.0) -> (x-y*floor(x/y)=w3269:dbl)  [unwired: 1 out]
          n2360 = Index Array(array=w3270, index=w3269) -> (element=w3267:i16)
          n2361 = Index Array(array=w3324, index (row)=0) -> (element=w3317:u16[])  [unwired: 1 in]
          n2362 = Index Array(array=w3277, index (row)=1) -> (element=w3284:u16[])  [unwired: 1 in]
          n2363 = Index Array(array=w3323, index=0) -> (element=w3322:i16)
          n2364 = Index Array(array=w3323, index=1) -> (element=w3318:i16)
          n2365 = Index Array(array=w3323, index=2) -> (element=w3319:i16)
          n2366 = Index Array(array=w3323, index=3) -> (element=w3320:i16)
          n2367 = Index Array(array=w3323, index=4) -> (element=w3321:i16)
          n2368 = Index Array(array=w3278, index=0) -> (element=w3279:i16)
          n2369 = Index Array(array=w3278, index=1) -> (element=w3283:i16)
          n2370 = Index Array(array=w3278, index=2) -> (element=w3282:i16)
          n2371 = Index Array(array=w3278, index=3) -> (element=w3281:i16)
          n2372 = Index Array(array=w3278, index=4) -> (element=w3280:i16)
          n2373 = Index Array(array=w3268, index (row)=0, index (col)=w3267) -> (element=w3264:u16)
          n2374 = Index Array(array=w3317, index=w3322) -> (element=w3316:u16)
          n2375 = Index Array(array=w3317, index=w3318) -> (element=w3315:u16)
          n2376 = Index Array(array=w3317, index=w3319) -> (element=w3314:u16)
          n2377 = Index Array(array=w3317, index=w3320) -> (element=w3312:u16)
          n2378 = Index Array(array=w3317, index=w3321) -> (element=w3313:u16)
          n2379 = Index Array(array=w3284, index=w3279) -> (element=w3285:u16)
          n2380 = Index Array(array=w3284, index=w3283) -> (element=w3286:u16)
          n2381 = Index Array(array=w3284, index=w3282) -> (element=w3287:u16)
          n2382 = Index Array(array=w3284, index=w3281) -> (element=w3289:u16)
          n2383 = Index Array(array=w3284, index=w3280) -> (element=w3288:u16)
          n2384 = Number To Boolean Array(number=w3264) -> (Boolean array=w3332:bool[])
          n2385 = Number To Boolean Array(number=w3316) -> (Boolean array=w3325:bool[])
          n2386 = Number To Boolean Array(number=w3314) -> (Boolean array=w3328:bool[])
          n2387 = Number To Boolean Array(number=w3312) -> (Boolean array=w3327:bool[])
          n2388 = Number To Boolean Array(number=w3313) -> (Boolean array=w3329:bool[])
          n2389 = Number To Boolean Array(number=w3285) -> (Boolean array=w3276:bool[])
          n2390 = Number To Boolean Array(number=w3287) -> (Boolean array=w3273:bool[])
          n2391 = Number To Boolean Array(number=w3289) -> (Boolean array=w3274:bool[])
          n2392 = Number To Boolean Array(number=w3288) -> (Boolean array=w3272:bool[])
          n2393 = Number To Boolean Array(number=w3315) -> (Boolean array=w3326:bool[])
          n2394 = Number To Boolean Array(number=w3286) -> (Boolean array=w3275:bool[])
          n2395 = Index Array(array=w3332, index=0) -> (element=→"Next":bool)
          n2396 = Index Array(array=w3325, index=0) -> ()  [unwired: 1 out]
          n2397 = Index Array(array=w3326, index=0) -> ()  [unwired: 1 out]
          n2398 = Index Array(array=w3328, index=0) -> ()  [unwired: 1 out]
          n2399 = Index Array(array=w3327, index=0) -> ()  [unwired: 1 out]
          n2400 = Index Array(array=w3329, index=0) -> ()  [unwired: 1 out]
          n2401 = Index Array(array=w3276, index=0) -> ()  [unwired: 1 out]
          n2402 = Index Array(array=w3275, index=0) -> ()  [unwired: 1 out]
          n2403 = Index Array(array=w3273, index=0) -> ()  [unwired: 1 out]
          n2404 = Index Array(array=w3274, index=0) -> ()  [unwired: 1 out]
          n2405 = Index Array(array=w3272, index=0) -> ()  [unwired: 1 out]
          n2406 = local read item#-1() -> ()  [unwired: 1 in]
          n2407 = local read item#-1() -> ()  [unwired: 1 in]
          n2408 = local read item#-1() -> ()  [unwired: 1 in]
          n2409 = local read item#-1() -> ()  [unwired: 1 in]
          n2410 = local read item#-1() -> ()  [unwired: 1 in]
          n2411 = local read item#-1() -> ()  [unwired: 1 in]
          n2412 = local read item#-1() -> ()  [unwired: 1 in]
          n2413 = local read item#-1() -> ()  [unwired: 1 in]
          n2414 = local read item#-1() -> ()  [unwired: 1 in]
          n2415 = local read item#-1() -> ()  [unwired: 1 in]
        }
      }
    }
    frame Enabled {
    }
  }
